vi "UHR-Fleezers Control (host) - 9.4.vi"() -> ()   [LabVIEW 2009]
uses:
  <vilib>/Utility/miscctls.llb/LVPoint32TypeDef.ctl
  <vilib>/Utility/miscctls.llb/LVMinMaxIncTypeDef.ctl
  <vilib>/userDefined/High Color/nirio_resource_hc.ctl
  <vilib>/Instr/_visa.llb/VISA Configure Serial Port (Instr).vi
  <vilib>/Platform/TimedLoop/XDataNode/XDataNode.xnode
  <vilib>/Platform/TimedLoop/XDataNode/loadlvalarms.vi
  <vilib>/Platform/TimedLoop/XDataNode/timing_clust.ctl
  <vilib>/Platform/TimedLoop/XDataNode/nitl_modes.ctl
  <vilib>/Platform/TimedLoop/XDataNode/wakeup.ctl
  <vilib>/rvi/interface/nirviOpenFPGA/nirviOpenFPGA.xnode
  FPGA Bitfiles/UHR-Fleezers Instr~3C_FPGA Target_UHR-Fleezers Contr~C3.lvbitx
  UHR-Fleezers Control (fpga) - 9.2.vi
  <vilib>/FPGAPlugInAG/PCIe-7852R/nirviIntfOpen_PCIe-7852R.vi
  <vilib>/rvi/interface/nirviMethod/nirviMethod.xnode
  <vilib>/Utility/error.llb/Merge Errors.vi
  <vilib>/LabVIEW Targets/FPGA/Rio/nirio_HostInterface/nirio_Reset.vi
  <vilib>/LabVIEW Targets/FPGA/Rio/nirio_HostInterface/nirio_DMAStopAll.vi
  <vilib>/rvi/interface/common/niFpgaNodeNameForErrorReporting.ctl
  <vilib>/rvi/errors/niLvFpgaWhatHappensToTopLevelVI.ctl
  <vilib>/LabVIEW Targets/FPGA/Rio/nirio_HostInterface/nirio_DisableInterrupts.vi
  <vilib>/Utility/error.llb/Error Cluster From Error Code.vi
  <vilib>/rvi/errors/niLvFpgaAdjustHostInterfaceError.vi
  <vilib>/rvi/interface/nirviReadWriteControl/nirviReadWriteControl.xnode
  <vilib>/LabVIEW Targets/FPGA/Rio/nirio_HostInterface/nirio_WriteBig.vi
  <vilib>/LabVIEW Targets/FPGA/Rio/nirio_HostInterface/nirio_DMAConfigure.vi
  <vilib>/LabVIEW Targets/FPGA/Rio/nirio_HostInterface/nirio_DMAStop.vi
  <vilib>/RVI Host/nirviSupport.llb/nirviErrorClusterFromErrorCode.vi
  <vilib>/LabVIEW Targets/FPGA/Rio/nirio_HostInterface/nirio_EnableInterrupts.vi
  <vilib>/rvi/errors/niLvFpgaReportInternalErrorWithAdditionalInfo.vi
  <vilib>/express/express analysis/Spectral/XNode/ExpressSpectralMeasurementsBlockNode.xnode
  <vilib>/express/express analysis/Spectral/Block/exnSpectralBlock spectral measurements PSD poly.vi
  <vilib>/express/express analysis/Spectral/Block/exnSpectralBlock spectral measurements PSD WFM.vi
  <vilib>/Waveform/WDTOps.llb/WDT Append Waveforms DBL.vi
  <vilib>/LabVIEW Targets/FPGA/Rio/nirio_HostInterface/nirio_ReadBig.vi
  <vilib>/rvi/interface/nirviCloseFPGA/nirviCloseFPGA.xnode
  <vilib>/FPGAPlugInAG/PCIe-7852R/nirviIntfClose_PCIe-7852R.vi
  <vilib>/vision/Avi1.llb/AviRefnum.ctl
  <vilib>/Analysis/NI_AALBase.lvlib
  <vilib>/Platform/TimedLoop/XDataNode/XDNodeRunTimeDep.lvlib
  openfpgaref.8.6.ctl
  NiRioSrv.dll
  <vilib>/vision/NI_Vision_Development_Module.lvlib
panel:
  out "Primary Video Display":T1(plugin-control)
  in  "Force Reset":bool
  in  "Force Yank":bool
  in  "Random Choice":bool=TRUE
  in  "N Array El":u8=3 min=1 step=1
  in  "Yank to Delta Array (MHz)":dbl[](array[numeric])=[16.3, 15.85, 14.85]
  in  "Yank Delay (s)":dbl=3.5
  in  "N pts to average":u16=6
  out "Fl. High":bool
  out "Waiting":bool
  in  "Fl. Delta Thresh. (kHz)":dbl=0.6
  in  "Fl. Triggered...":bool
  in  "Action":string(combo)="Yank"
  out "Duration (s)":dbl
  out "Waveform Graph":dbl[](graph) caption="APD Line Scan"
  in  "Total Volume\nFlushed (uL)":dbl
  in  "Inject Pump 2":bool caption="Inject Pump 2\n(Flush Center)"
  in  "Inject Pump 3":bool caption="Inject Pump 3\n(ADig Beads)"
  in  "Inject Pump 1 (DNA)":bool caption="Inject Pump 1 \n(DNA Beads)"
  out "Messages":string
  in  "APD Ave N":dbl=10.0
  out "Int. Time (s)":dbl
  in  "Stop All":bool
  out "sigma/mean":dbl
  out "Rate sigma (Hz)":dbl format="%0.2f"
  in  "Index":dbl=1.0 caption="Save File Index" min=1.0 step=1.0
  in  "Tab Control 6":T2(tab)=enum."Dual Display (Trap + APD)"
  out "All Signals":waveform(dbl)[](graph)
  in  "Signals to Plot":i32(listbox)
  out "Trap Disp. Freq. (Hz)":dbl caption="Freq. (Hz)" format="%#_6p"
  out "Display Period (s)":dbl caption="Period (s)" format="%#_6p"
  in  "Trap Disp. Downsample":dbl=20000.0 caption="Downsample"
  in  "APD Disp. Scale":dbl=0.1 caption="Scale (Divide,\nfor above plot only)"
  in  "APD Disp. Downsample":dbl=30.0 caption="Integrate" min=1.0 step=1.0
  out "APD Display Freq. (Hz)":dbl caption="Freq. (Hz)"
  out "APD Display Period (s)":dbl caption="Period (s)"
  out "RMS (Ang)":dbl format="%_2g"
  in  "Bead Sep. Int. Time (s)":dbl=5.0 caption="Int. Time (s)"
  in  "Below (kHz)":dbl=0.5
  in  "Above (kHz)":dbl=2.0
  in  "Adjust Scale\nto Mean":bool
  in  "Rescale on Mean":bool
  in  "Offset (nm)":dbl
  out "Mean":dbl caption="Mean (pN)" format="%#_3g"
  out "Force":waveform(dbl)[](graph)
  out "APD 1 Chart":waveform(dbl)(graph)
  in  "Calibration":u16(ring)=2 items=["None", "Position", "Force"]
  out "T1 X":dbl caption="T1 X (pN)" format="%0.2f"
  out "T2 X":dbl caption="T2 X (pN)" format="%0.2f"
  out "Bead Separation":waveform(dbl)(graph)
  in  "Amplitude (nm)":dbl=1.0
  out "Bead Mean (nm)":dbl caption="Mean (nm)" format="%0.2f"
  out "Difference":dbl caption="Difference (pN)" format="%.2g"
  out "APD 1 Graph":dbl[](graph) caption="Most Recent Time Trace"
  out "Trap Delta Graph":dbl[](graph) caption="Most Recent Time Trace"
  out "size(s) APD array":i32
  out "size(s) of 1 acq array":i32
  out "Delta Fl. (Hz)":dbl
  out "APD 1 Graph 2":dbl[](graph) caption="Most Recent Time Trace"
  in  "Flip Green Filter":bool
  in  "Set X Only":bool
  in  "Set Y Only":bool
  out "Detection Laser X":T1(plugin-control)
  out "APD 1":T1(plugin-control)
  out "Detection Laser Y":T1(plugin-control)
  out "Pointer Y (V)":dbl format="%_3g"
  out "Pointer X (V)":dbl format="%_3g"
  in  "Set Confocal Spot (X-Y)":bool
  out "FFT 1":cluster{"f0":dbl, "df":dbl, "magnitude":dbl[]}[](graph)
  out "FFT 2":cluster{"f0":dbl, "df":dbl, "magnitude":dbl[]}[](graph)
  in  "FFT 1 Choice 1":u16(ring) items=["T1 Y", "T1 X", "T1 Sum", "T2 Y", "T2 X", "T2 Sum", "T1 FB X", "T1 FB Sum", "T2 FB X", "T2 FB Sum", "PSD Y", "PSD X", "PSD Y Sum", "none"]
  in  "FFT 2 Choice 1":u16(ring)=13 items=["T1 Y", "T1 X", "T1 Sum", "T2 Y", "T2 X", "T2 Sum", "T1 FB X", "T1 FB Sum", "T2 FB X", "T2 FB Sum", "PSD Y", "PSD X", "PSD Y Sum", "none"]
  in  "FFT 1 Choice 2":u16(ring)=1 items=["T1 Y", "T1 X", "T1 Sum", "T2 Y", "T2 X", "T2 Sum", "T1 FB X", "T1 FB Sum", "T2 FB X", "T2 FB Sum", "PSD Y", "PSD X", "PSD Y Sum", "none"]
  in  "FFT 2 Choice 2":u16(ring)=13 items=["T1 Y", "T1 X", "T1 Sum", "T2 Y", "T2 X", "T2 Sum", "T1 FB X", "T1 FB Sum", "T2 FB X", "T2 FB Sum", "PSD Y", "PSD X", "PSD Y Sum", "none"]
  in  "Compute FFT":bool
  in  "Reset FFT":bool
  in  "# Spectra to Ave.":dbl=100.0
  out "Ave. Time (s)":dbl
  out "1 Channel":waveform(dbl)(graph)
  out "Slow mean":dbl format="%0.2f"
  in  "Slow mean N ave.":dbl=1.0 min=1.0 step=1.0
  out "Mean Intensity":dbl
  out "Sigma":dbl
  out "Sigma/Mean":dbl
  in  "Subtract mean":bool
  in  "High Res. Display":u16(ring) items=["T1 Y", "T1 X", "T1 Sum", "T2 Y", "T2 X", "T2 Sum", "T1 FB X", "T1 FB Sum", "T2 FB X", "T2 FB Sum", "PSD Y", "PSD X", "PSD Y Sum"]
  out "APD 1 Rate (Hz)":dbl format="%#_3p"
  in  "Tab Control":T3(tab)
  in  "TA Green Off?":bool
  in  "TA Cancel Save?":bool
  in  "Cal @ (MHz)":dbl=15.0
  out "Stage Moving":bool
  in  "Lower Ch. Cap.":bool
  in  "W/ Offset":bool=TRUE
  in  "Read Cal":bool
  out "Tether":bool
  in  "Tether Alarm?":bool=TRUE
  in  "Move to Delta 1 (MHz)":dbl=14.85
  in  "Then...":string(combo)="5"
  in  "Data Acq. Spot":bool
  in  "Confocal Linescan":bool
  in  "Speed (nm/s)":dbl=100.0
  in  "Stop F (pN)":dbl=3.0
  in  "Furthest Withdraw (MHz)":dbl=15.0
  in  "Closest Delta (MHz)":dbl=9.75 step=0.25
  in  "Fish for Tether":bool
  in  "Confocal Image":bool
  in  "Round T1 X":bool caption="Round"
  in  "T1 offset_x (mV)":dbl=-26.302542012392074 format="%#_2g"
  in  "T1 kappa_x (pN/nm)":dbl=0.22546432407642192 min=0.0 step=0.001 format="%#_2g"
  out "Time (s)":dbl
  out "Total Time (s)":dbl
  in  "Start Saving":bool
  in  "Limits Enable":bool=TRUE caption="Enable"
  in  "Limit Max (MHz)":dbl=16.0 caption="Max (MHz)"
  in  "Limit Min (MHz)":dbl=10.0 caption="Min (MHz)"
  in  "Cal sets to save":u32=50 min=1 step=1
  in  "Comment (data description)":string="testing confocal setup"
  out "Calibrating Trap...":bool
  in  "Trap 2 (ON/OFF)":bool
  in  "Trap 1 (ON/OFF)":bool
  in  "Save Calibration":bool
  in  "N sets to save":u32=200 caption="N Sets"
  in  "Save N Sets":bool
  out "Save file name":path
  in  "Save ave N":dbl=500.0 caption="Averaging Factor"
  out "Saving...":bool
  in  "Stop Saving":bool
  out "Progress":u16(slide) scale=0.0..100.0
  out "Manipulating Trap":bool
  out "Buffer Status":dbl(slide) scale=0.0..1.0
  out "Overflow (data lost)":bool
  in  "Reset":bool
  out "Data Rate (Hz)":dbl caption="Trap Data Rate (Hz)" format="%#_3p"
  out "Data Period (s)":dbl caption="Trap Data Period (s)" format="%#_6p"
  out "Save Data Rate (Hz)":dbl caption="Rate (Hz)" format="%#_6p"
  out "Save Data Period (s)":dbl caption="Period (s)" format="%#_6p"
  in  "T1 alpha_x (nm/V)":dbl=630.439304367558 step=10.0 format="%#_3g"
  in  "T2 alpha_x (nm/V)":dbl=704.7738222964198 step=10.0 format="%#_3g"
  in  "T2 kappa_x (pN/nm)":dbl=0.2030110880477556 min=0.0 step=0.001 format="%#_2g"
  in  "T2 offset_x (mV)":dbl=-26.67973517613748 format="%#_2g"
  in  "BD 1 Frequency 1 (MHz)":dbl=70.15 caption="T1 X (MHz)" min=60.0 max=90.0 step=1.0 format="%#_6p"
  in  "BD 1 Frequency 2 (MHz)":dbl=85.0 caption="T2 X (MHz)" min=60.0 max=90.0 step=1.0 format="%#_6p"
  in  "Green Laser ON/Interlacing":bool
  in  "Round T2 X":bool caption="Round"
  in  "AO1":dbl(slide)=5.61 caption="Confocal Y (V)" min=0.0 max=10.0 step=0.01 scale=0.0..10.0 scale format="%_1f"
  in  "AO2":dbl(slide)=3.9 caption="Confocal X (V)" min=0.0 max=10.0 step=0.01 scale=0.0..10.0 scale format="%_1f"
  in  "Upper Cap.":bool
  in  "Lower Cap.":bool
  in  "Trap Raster Scan":bool
  out "Raster Scanning...":bool
  in  "Trap Delta (MHz)":dbl=15.0
  in  "Dump Beads":bool
  in  "Wait Before Save (s)":u32=1
  out "Attempts":dbl
  in  "Attempt Limit":dbl=30.0 caption="Limit"
  in  "Setpoints (V)":cluster{"Set 1":dbl, "Set 2":dbl}={"Set 1"=9.0, "Set 2"=9.0}
  in  "Offset @ (MHz)":dbl=13.0
  in  "Move to Delta 2 (MHz)":dbl=15.0
  in  "Position Label 5":string="Lower Channel Cap" caption="5"
  in  "Move to Position":bool
  in  "Position":dbl=1.0 min=1.0 max=10.0 step=1.0
  in  "Set Position":bool
  in  "Saved Stage Positions":dbl[][](array[numeric])=[[1.0, 1.06186, -0.64809, -0.00713], [2.0, 0.0, 0.0, 0.0], [3.0, 2.01611, -0.29927, -0.00713], [4.0, 2.01611, 0.31655, -0.00713], [5.0, 0.0, 0.0, 0.0], [6.0, 0.0, 0.0, 0.0], [7.0, 0.0, 0.0, 0.0], [8.0, 0.0, 0.0, 0.0], [9.0, 0.0, 0.0, 0.0], [10.0, 0.0, 0.0, 0.0]]
  in  "Move to Position 5":bool
  in  "z nudge increment (um)":dbl=0.5
  in  "+z":bool
  in  "Position 1 Label":string="Upper capillary" caption="1"
  in  "Set Position 1":bool
  in  "Set Position 2":bool
  in  "Set Position 3":bool
  in  "Set Position 4":bool
  in  "Move to Position 3":bool
  in  "Move to Position 4":bool
  in  "Move to Position 2":bool
  in  "Move to Position 1":bool
  in  "Position 2 Label":string="Lower capillary" caption="2"
  in  "Position 3 Label":string="Measurement spot" caption="3"
  in  "Position 4 Label":string="Dump beads" caption="4"
  in  "-z":bool
  in  "Set Position 5":bool
  out "Stage Control Serial Error":errorcluster
  in  "Top Ch Inject Rate (ul/h)":dbl=10.0
  in  "Pump write delay (ms)":dbl=300.0
  in  "All Pump Parameters":T4={"Pump 1"={"Diameter (mm)"=4.61, "Units"=3.0, "Volume"=0.0, "Rate"=0.0}, "Pump 2"={"Diameter (mm)"=4.61, "Units"=3.0, "Volume"=0.0, "Rate"=0.0}, "Pump 3"={"Diameter (mm)"=4.61, "Units"=3.0, "Volume"=0.0, "Rate"=0.0}}
  in  "Top Ch Inject Volume (uL)":dbl=100.0
  in  "Pump pause delay (ms)":u32
  in  "Bottom Ch Inject Volume (uL)":dbl=100.0
  in  "Bottom Ch Inject Rate (ul/h)":dbl=10.0
  in  "Flush Center Ch Volume (uL)":dbl=15.0
  in  "Flush Center Ch Rate (ul/m)":dbl=100.0
  in  "Tab Control 2":T5(tab)=enum."AOD Raster Scan"
  out "Total Counts (ticks)":u32
  in  "Trap ON/OFF X or Y Amp?":bool=TRUE
  in  "Oscillate Set 1":bool
  in  "Trap 1 ON":bool
  in  "Number Interlace Sets":u8=3 min=1 max=3
  in  "DIO count 3 (ticks)":u32=200
  in  "DIO count 2 (ticks)":u32=200
  in  "DIO count 1 (ticks)":u32=200
  in  "BD 2 Amplitude 3 (%)":dbl min=0.0 max=50.0 step=1.0
  in  "BD 2 Amplitude 2 (%)":dbl min=0.0 max=50.0 step=1.0
  in  "BD 2 Amplitude 1 (%)":dbl min=0.0 max=50.0 step=1.0
  in  "BD 1 Amplitude 3 (%)":dbl min=0.0 max=50.0 step=1.0
  in  "BD 1 Amplitude 2 (%)":dbl=35.0 min=0.0 max=50.0 step=1.0
  in  "BD 1 Amplitude 1 (%)":dbl=10.0 min=0.0 max=50.0 step=1.0
  in  "BD 2 Frequency 3 (MHz)":dbl=26.0 min=0.0 max=40.0 step=1.0 format="%#_6p"
  in  "BD 1 Frequency 3 (MHz)":dbl=70.0 min=60.0 max=90.0 step=1.0 format="%#_6p"
  in  "BD 2 Frequency 2 (MHz)":dbl=26.0 min=0.0 max=40.0 step=1.0 format="%#_6p"
  in  "BD 2 Frequency 1 (MHz)":dbl=26.0 min=0.0 max=40.0 step=1.0 format="%#_6p"
  in  "Not-Interlacing Set":enum32{"Set 1", "Set 2", "Set 3"}(radio)
  in  "Interlace":bool=TRUE
  in  "Trap 2 ON":bool
  in  "Trap 3 ON":bool
  in  "Scan axis 2":bool=TRUE
  in  "Osc. freq. (Hz)":dbl=0.25
  in  "Osc. amp. (MHz)":dbl=2.0
  out "Coords":T6
  in  "Manipulation Scaling":cluster{"Horizontal":dbl, "Vertical":dbl}={"Horizontal"=0.075, "Vertical"=0.01}
  in  "Freq or Amp switch first":bool=TRUE
  in  "Swap F1 and F2":bool
  in  "Freq switch delay":u16
  in  "Amp switch delay":u16=5
  in  "MCL Step Increment (V_int)":dbl=3.0
  out "Time to Finish All (min)":dbl format="%#_2p"
  in  "Scan Speed (nm/s)":dbl=100.0
  in  "Scan Range (nm)":dbl=200.0
  in  "Step Size (nm)":dbl=1.0
  in  "MCL/AOM Scale Tweak":dbl=1.0
  in  "MCL Step Position Ratio":dbl=0.5
  in  "Move MCL Also?":bool=TRUE
  out "Final sep (nm)":dbl
  out "Initial sep (nm)":dbl
  out "Save index":dbl
  out "Final delta (MHz)":dbl
  out "Initial delta (MHz)":dbl
  out "Final freq. (MHz)":dbl
  out "Initial freq. (MHz)":dbl
  in  "Saved AOD Raster Scan Parameter Sets":T7(array[cluster])=[{"Scan Range AOD (nm) 2"=500.0, "Step Size AOD (nm) 2"=1.0, "Scan Speed AOD (nm/s) 2"=200.0, "Number of scans (AOD) 2"=1, "Label"=""}, {"Scan Range AOD (nm) 2"=1000.0, "Step Size AOD (nm) 2"=1.0, "Scan Speed AOD (nm/s) 2"=200.0, "Number of scans (AOD) 2"=5, "Label"="wide offset scan"}, {"Scan Range AOD (nm) 2"=20.0, "Step Size AOD (nm) 2"=0.68, "Scan Speed AOD (nm/s) 2"=0.68, "Number of scans (AOD) 2"=1, "Label"="2 bp steps"}]
  in  "Load parameters":bool
  out "Scan Range (MHz)":dbl=10.0
  in  "Restart DMA? (AOD)":bool=TRUE caption="Restart DMA?"
  out "Incr. int (AOD)":i64
  out "Time/Scan (s) (AOD)":dbl format="%#_2p"
  out "Data points/scans":dbl
  out "Data points/scan (f/b)":dbl
  in  "Save scans":bool=TRUE
  out "AOD Scan I":u64 caption="Scan I"
  in  "Continuous AOD Scanning":bool caption="Continuous Scanning"
  in  "Abort AOD Scan":bool caption="Abort Scan"
  in  "Scan BD":bool=TRUE
  out "Cycles/step (AOD)":u64=400 format="%.0p"
  in  "Number of F/B Scans (AOD)":u16=3 min=1
  out "Scan steps (AOD)":u64=1000
  out "Scan Increment (MHz)":dbl=0.2
  out "AOD Scanning":bool caption="Scanning"
  in  "Start AOD Scan":bool caption="Start Scan"
  out "N sets should be saved":dbl
  out "Progress 2":u16(slide) caption="Progress" scale=0.0..100.0
  in  "Abort save 2":bool caption="Abort save"
  in  "Trap 1 Bead Size (nm)":dbl=860.0
  in  "Trap 2 Bead Size (nm)":dbl=790.0
  out "MCL Count":dbl
  in  "All FB On/Off":bool=TRUE
  in  "AI2 to Setpoint":cluster{"Set 1":bool, "Set 2":bool}
  out "AI2 (V)":cluster{"Set 1":dbl, "Set 2":dbl}
  in  "Reset Feedback":cluster{"Set 1":bool, "Set 2":bool}
  in  "PID Gains":T8={"Set 1"={"proportional gain (Kc)"=0, "integral gain (Kc*Ts/Ti)"=5, "derivative gain (Kc*Td/Ts)"=0}, "Set 2"={"proportional gain (Kc)"=0, "integral gain (Kc*Ts/Ti)"=5, "derivative gain (Kc*Td/Ts)"=0}}
  in  "Feedback On/Off":cluster{"Set 1":bool, "Set 2":bool}={"Set 1"=TRUE, "Set 2"=TRUE}
  in  "Tab Control 3":enum32{"Timing", "MCL Scan", "Analog Out"}(tab)=enum."MCL Scan"
  out "APD Gate Late Counter":u32
  in  "- phase (APD Gate)":bool
  in  "+ phase (APD Gate)":bool
  out "APD Gate Relative Phase":i16
  in  "Phase Adj. (APD Gate)":i16=20
  in  "Initial Phase Adjustment (APD Gate)":i16=50
  in  "Save APD Data\nwith Trap Data":bool=TRUE
  out "APD FIFO Elements Remaining":u32
  in  "- phase (APD Acq)":bool
  in  "+ phase (APD Acq)":bool
  out "APD Acq Late Counter":u32
  out "APD Acq Relative Phase":i16
  in  "Phase Adj. (APD Acq)":i16=20
  in  "Initial Phase Adjustment (APD Acq)":i16
  in  "Invert APD Gate":bool caption="Invert Gate"
  in  "APD Gate OFF Count":u32=450 caption="Gate OFF Count"
  in  "APD Gate ON Count":u32=150 caption="Gate ON Count"
  in  "APD Gate":enum32{"ON", "OFF", "Interlace"}(radio)=enum."Interlace"
  in  "APD Integration Time (s)":dbl=0.01 caption="Integration Time (s)"
  out "APD Acq Rate (Hz)":dbl=20000000.0 caption="Rate (Hz)"
  out "APD Samples/FIFO Acq.":dbl
  out "APD Elements/DMA read":u32
  out "APD Int. Count":u32 format="%.0p"
  in  "Tab Control 5":enum32{"PSD X", "PSD Y", "Other Data Channel"}(tab)
  out "Data map":dbl[][](graph)
  in  "Channel":i32=4
  in  "Abort MCL Scan":bool
  out "MCL Scan I":u64
  out "MCL Scanning":bool
  in  "Start MCL Scan":bool
  out "wait to reset values":bool
  in  "Tab Control 4":enum32{"Scan Settings", "MCL FPGA Loop Timing"}(tab)
  out "Total Time (s)":dbl
  in  "Scan lines (y)":u64=20
  in  "Fast Scan Dir":bool=TRUE
  in  "2D or 1D Scan":bool=TRUE
  out "Initial X":dbl
  out "Initial Y":dbl
  out "Time/f+b scan (s) (MCL)":dbl caption="Time/scan (s)"
  in  "Number of scans (MCL)":u64=1 caption="Scans"
  in  "Scan steps (MCL)":u64=40 caption="Scan steps (x)"
  in  "N APD Samp/step":dbl=3.0
  in  "Scan Range (V)\n(of steps)":dbl=3.5
  in  "Restart DMA? (MCL)":bool=TRUE caption="Restart DMA?"
  in  "Continuous MCL Scanning":bool caption="Cont. Scanning"
  in  "Center Scan":bool=TRUE
  in  "Save Data (MCL)":bool=TRUE caption="Save Data"
  out "Actual Incr. int (MCL)":i16 caption="Incr. int"
  out "Desired incr (int)":dbl
  out "Desired Scan Incr (V)":dbl
  out "N sets should be saved (MCL)":dbl caption="N sets should be saved"
  out "Data points/scans (MCL)":dbl caption="Data points/scans"
  out "Data points/scan (f+b)":dbl caption="points/scan (f+b)"
  out "Cycles/step (MCL)":u64 caption="Cycles/step" format="%.0p"
  out "Actual MCL Inc (V)":dbl
  in  "Phase adjust (MCL)":i16 caption="Phase adjust"
  out "Relative Phase (MCL)":i16 caption="Relative Phase"
  in  "Initial Phase Adj. (MCL)":i16 caption="Initial Phase Adj."
  in  "Update Count (MCL)":u32=600
  in  "+ phase (MCL)":bool
  in  "- phase (MCL)":bool
  out "MCL Late Counter":u32
  in  "APD 1 AO Mult.":i16=1 min=1
  in  "APD 2 AO Mult.":i16=1 min=1
  in  "APD 1 AO offset":i16
  in  "APD 2 AO offset":i16
  in  "Tab Control 7":enum32{"Green FB Signals", "Slow MCL Scan"}(tab)
  out "Green FB Plot":dbl(graph)
  out "MCL Scan 2":cluster{"Begin (V)":dbl, dbl, dbl[]}(graph)
  out "MCL Scan":cluster{"Begin (V)":dbl, dbl, dbl[]}(graph)
  in  "Green laser mode":enum32{"Laser ON", "Laser OFF", "Interlace"}(radio)=enum."Interlace"
  in  "GI Frequency, ON count":u32=150 min=1 step=1
  in  "Invert GI":bool
  out "GI Late Counter":u32
  in  "Phase adj. (GI)":i16=5
  out "GI relative phase":i16
  in  "+ phase (GI)":bool
  in  "Initial Phase Adjustment (GI)":i16=15
  in  "GI Frequency, OFF count":u32=450 min=1 step=1
  in  "- phase (GI)":bool
  out "Green FB Signals (V)":cluster{"Y":dbl, "X":dbl, "Sum":dbl}
  out "Relative phase (Green FB)":i16
  in  "+ phase (Green FB)":bool
  in  "- phase (Green FB)":bool
  in  "Green FB Count":u32=600
  in  "Phase adj. (Green FB)":i16=10
  in  "Initial Phase Adjustment (Green FB)":i16=50
  in  "Green FB On/Off":bool=TRUE
  in  "Current When FB OFF (%)":dbl=87.0 min=0.0 max=100.0 step=1.0
  in  "Green int current ON count adj":u32=150
  in  "Green FB Gains":T9={"proportional gain (Kc)"=10, "integral gain (Kc*Ts/Ti)"=5, "derivative gain (Kc*Td/Ts)"=0}
  in  "Green FB Setpoint (mV)":dbl=100.0
  in  "- phase (GI) 2":bool
  in  "Initial Phase Adjustment (GI) 2":i16=-100
  in  "+ phase (GI) 2":bool
  out "GI relative phase 2":i16
  in  "Phase adj. (GI) 2":i16=20
  out "GI Late Counter 2":u32
  in  "# Samples/trap":dbl=20000.0 format="%#_6p"
  out "Elements/DMA read":u32 format="%.0p"
  out "Ave. Rate (Hz)":dbl format="%#_6p"
  out "FIFO El. Rem.":u32 format="%.0p"
  in  "Phase adj. (AI1)":i16=15
  out "Relative phase (AI1)":i16
  in  "+ phase (AI1)":bool
  in  "- phase (AI1)":bool
  out "Late Counter (AI1)":u32
  in  "Initial Phase Adjustment (AI1)":i16=220
  out "AI rate (Hz)":dbl=50000.0 format="%#_6p"
  in  "AI Count (ticks)":u32=200
  out "# Samples/channel":u32=20000 format="%.0p"
  in  "FIFO Depth":u32=600000 format="%.0p"
  in  "Detector Type":string(combo)="IR-QPD + PSD + FB-QPD X position"
  in  "N Acq Sets (Traps + Fl.)":i16=3
  in  "Sets to FIFO (Traps)":T10={"Set 1"=TRUE, "Set 2"=TRUE, "Set 3"=FALSE}
  in  "FPGA Ave.":dbl=1.0 min=1.0 step=1.0
  out "Ave. Period (s)":dbl format="%#_6p"
  out "DMA Update Period (s)":dbl
  out "FPGA Averaging":bool
  out "Trap Sets":i16
  out "Counts/DMA":dbl format="%#_6p"
  in  "Video Capture Rate (Hz)":dbl=30.0
  in  "Video Index":dbl=1.0 min=1.0 step=1.0
  in  "New Video File":bool
  in  "Save Video":bool
  in  "Reset Averaging":bool
  in  "Averaging":bool
  in  "Save Image":bool
  in  "Image Index":dbl=1.0 min=1.0
  out "Path Out":path
  in  "Center Point":cluster{"X":i32, "Y":i32}={"X"=335, "Y"=271}
  in  "Zoom Factor":sgl=7.0
  out "Window Size":cluster{"Width":i32, "Height":i32}
  out "Window Position":cluster{"X Position":i32, "Y Position":i32}={"X Position"=40, "Y Position"=40}
  in  "Initial Window Size":cluster{"Width":i32, "Height":i32}={"Width"=884, "Height"=619}
  in  "Initial Window Position":cluster{"X Position":i32, "Y Position":i32}={"X Position"=796, "Y Position"=4}
  in  "Intensity Upper":dbl=88.0
  in  "Intensity Lower":dbl=66.0
  out "error out":errorcluster
  out "error out 2":errorcluster
  in  "Lost Tether Alarm Threshold (pN)":dbl=0.5
  in  "AOM X Cal (nm/MHz)":dbl=123.0
  in  "MCL X Cal (nm/V)":dbl=1070.0
  out "X RF Amplitude Limits (%)":T11={"Minimum"=0.0, "Maximum"=50.0, "Increment"=1.0}
  out "X RF Frequency Limits (MHz)":T11={"Minimum"=60.0, "Maximum"=90.0, "Increment"=1.0}
  out "Y RF Frequency Limits (MHz)":T11={"Minimum"=60.0, "Maximum"=90.0, "Increment"=1.0}
  out "Y RF Amplitude Limits (%)":T11={"Minimum"=0.0, "Maximum"=50.0, "Increment"=1.0}
  in  "Manip. X?":bool=TRUE
  in  "Manip. Y?":bool
  in  "Force Manip Abort":bool
  out "Read cal error":errorcluster
  in  "DAQ Delay (ms)":u32=1000
  in  "Start Scan":bool
  in  "Scan axis":bool=TRUE
  in  "Osc. amp. (V)":dbl=5.0
  in  "Osc. center (V)":dbl=5.0
  in  "Osc. freq. (Hz) 2":dbl=1.0
  in  "MCL Mode":u16(ring) items=["Manual Positioning", "Sinusoidal Wave", "Linear Scan"]
  in  "Begin (V)":dbl
  in  "End (V)":dbl=10.0
  in  "N Points":dbl=20.0
  in  "Delay to Interlace (s)":dbl
  in  "Delayed Interlace Start":bool
  in  "Read Lateness and Rel Phase":bool
  out "Vec Mean of T1 T2":dbl[](array[numeric])
  in  "Cal read wait (s)":u32=5
  out "Time tether formed":timestamp
  in  "Sample Chamber Stage Serial Port":refnum<visa-resource-name>="ChamberStageCOM4"
  in  "Syringe Pump Serial Port":refnum<visa-resource-name>="ChemyxPumpCOM3"
  # "Trap Display:"
  # "APD Display:"
  # "DAQ"
  # "Move Stage and Take Action"
  # "Trap Manipulation"
  # "Data Saving"
  # "Bead Calibration"
  # "Trap Position Difference Limits"
  # "DNA Beads"
  # "ADig Beads"
  # "Center channel"
  # "Units: \n1 = ml/m\n2 = ml/h\n3 = ul/m\n4 = ul/h"
  # "Rate param is ul/h\nVolume param is ul"
  # "X"
  # "Y"
  # "Oscillate Set 1 freq. (debugging)"
  # "BD 1"
  # "BD 2"
  # "AOD Raster Scan"
  # "Approx. trap separations"
  # "X"
  # "Y"
  # "Gate"
  # "X"
  # "2D"
  # "Y"
  # "1D"
  # "Green Laser Interlacing"
  # "Green FB Measurement"
  # "Digital Gate"
  # "Current Analog Control"
  # "Total AI Rates (NOT rates/trap)"
  # "(Samples/trap x Trap Sets)"
  # "(Samples/channel x\n8 if averaging (8 channels)\n4 if no averaging)"
  # "Trap 1"
  # "Trap 2"
  # "Flour./Trap 3"
  # "External Video Window"
  # "MCL Position Debugging"
  # "Temporary Control Storage\n(these used to be somewhere else, still want to keep them)"
  # "Y"
  # "X"
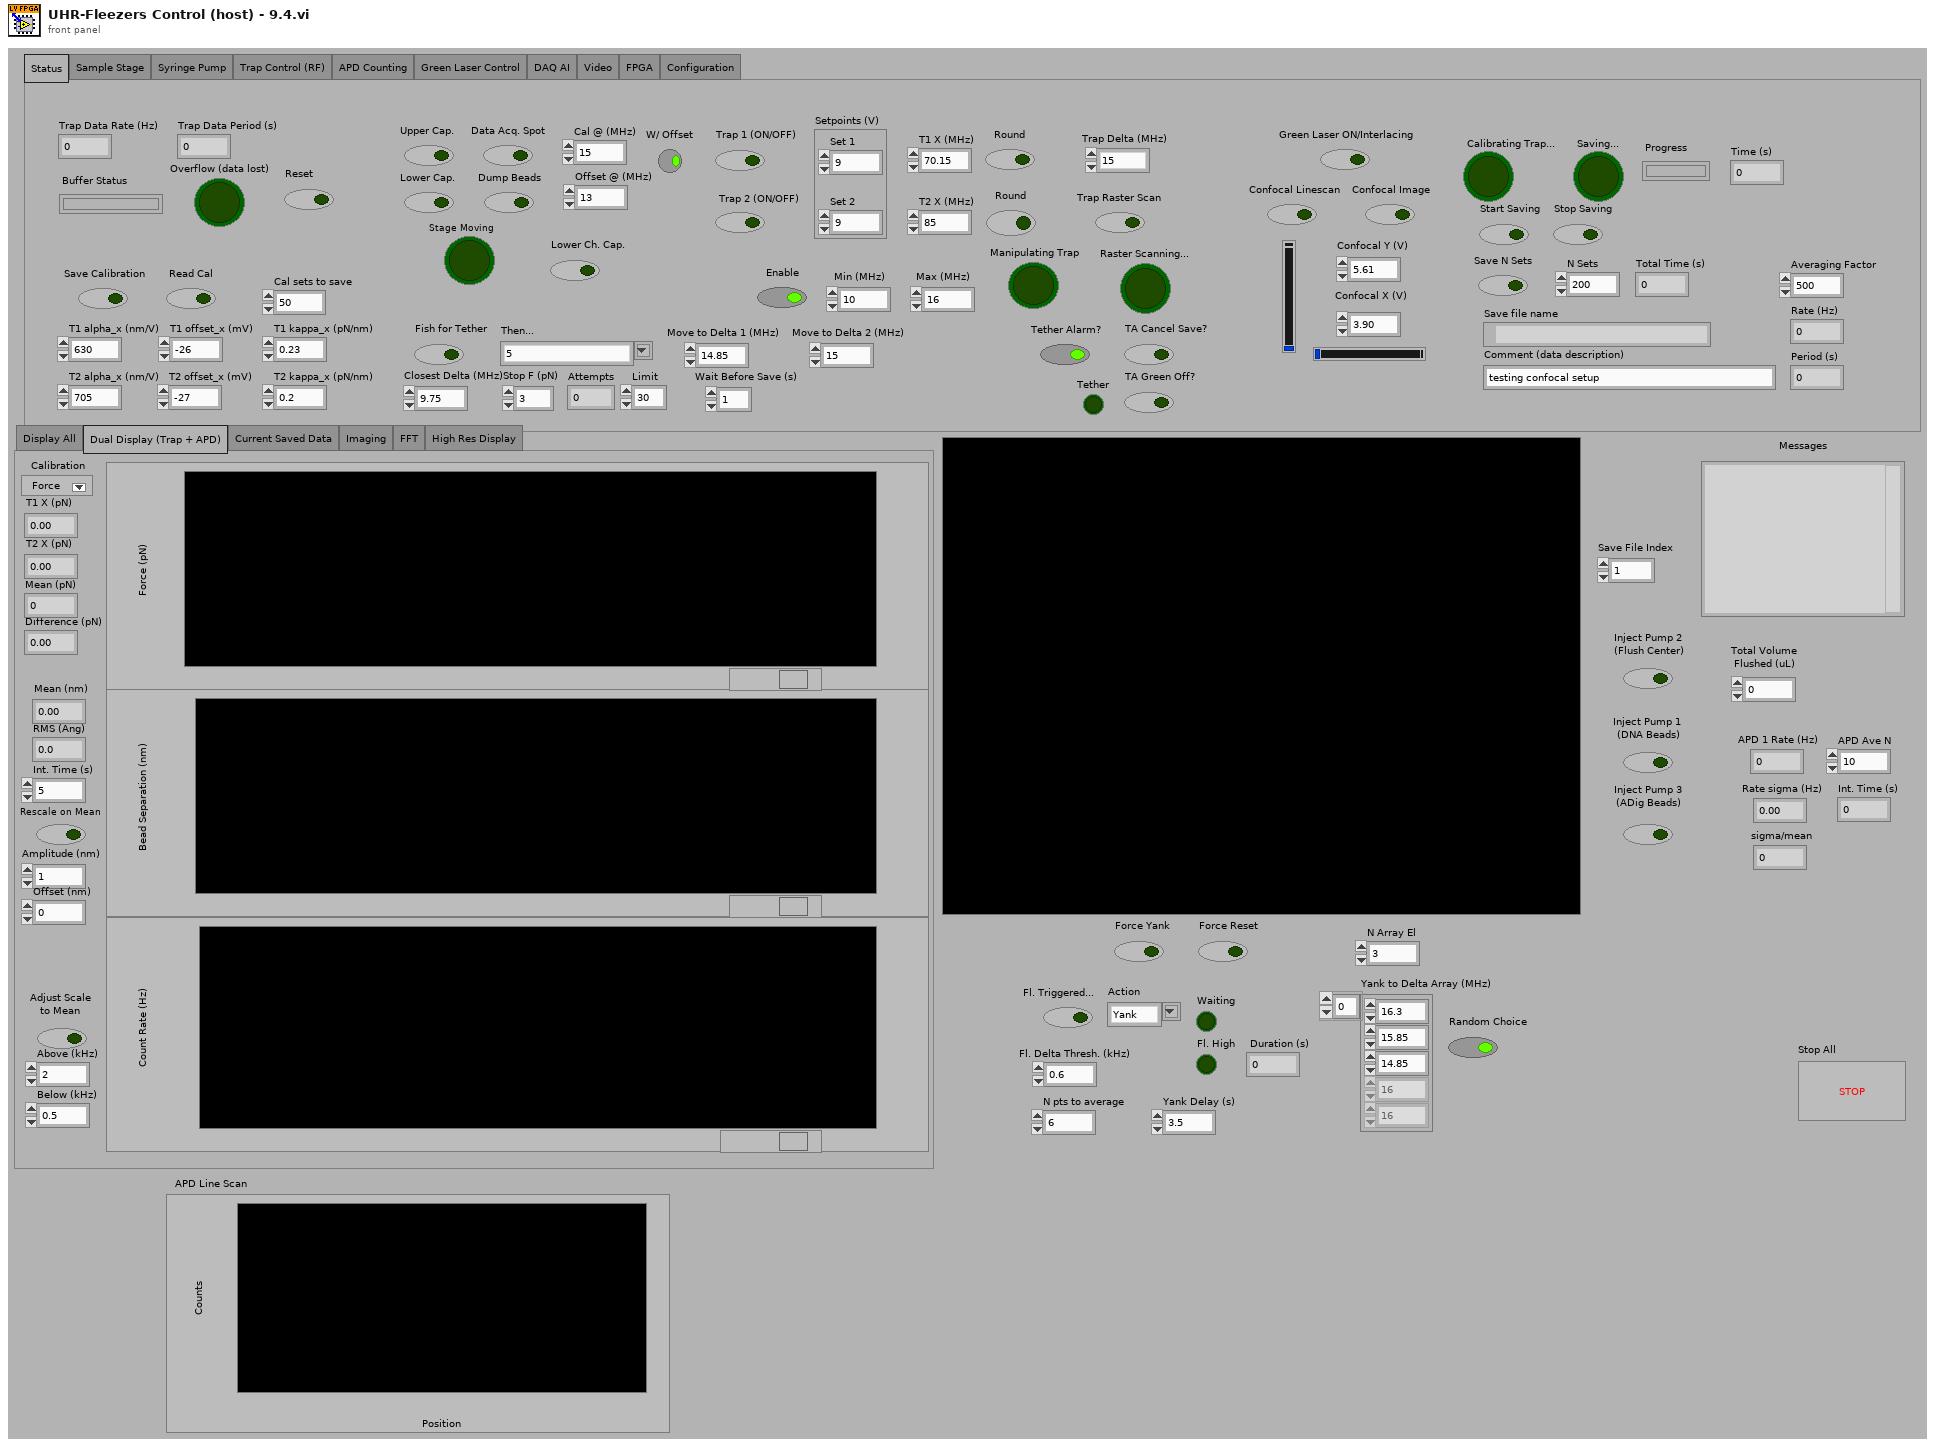
[diagram p1: front panel]
types:
  T1 = typedef "IMAQ Image.ctl" = refnum<image>
  T2 = enum32{"Display All", "Dual Display (Trap + APD)", "Current Saved Data", "Imaging", "FFT", "High Res Display"}
  T3 = enum32{"Status", "Sample Stage", "Syringe Pump", "Trap Control (RF)", "APD Counting", "Green Laser Control", "DAQ AI", "Video", "FPGA", "Configuration"}
  T4 = cluster{"Pump 1":cluster{"Diameter (mm)":dbl, "Units":dbl, "Volume":dbl, "Rate":dbl}, "Pump 2":cluster{"Diameter (mm)":dbl, "Units":dbl, "Volume":dbl, "Rate":dbl}, "Pump 3":cluster{"Diameter (mm)":dbl, "Units":dbl, "Volume":dbl, "Rate":dbl}}
  T5 = enum32{"IR Laser Interlacing (Direct RF Board Control Method)", "AOD Raster Scan", "Feedback on BD 1 Amp to Control AI2"}
  T6 = typedef "LVPoint32TypeDef.ctl" = cluster{"Horizontal":i32, "Vertical":i32}
  T7 = cluster{"Scan Range AOD (nm) 2":dbl, "Step Size AOD (nm) 2":dbl, "Scan Speed AOD (nm/s) 2":dbl, "Number of scans (AOD) 2":u16, "Label":string}[]
  T8 = cluster{"Set 1":cluster{"proportional gain (Kc)":i16, "integral gain (Kc*Ts/Ti)":i16, "derivative gain (Kc*Td/Ts)":i16}, "Set 2":cluster{"proportional gain (Kc)":i16, "integral gain (Kc*Ts/Ti)":i16, "derivative gain (Kc*Td/Ts)":i16}}
  T9 = cluster{"proportional gain (Kc)":i16, "integral gain (Kc*Ts/Ti)":i16, "derivative gain (Kc*Td/Ts)":i16}
  T10 = cluster{"Set 1":bool, "Set 2":bool, "Set 3":bool}
  T11 = typedef "LVMinMaxIncTypeDef.ctl" = cluster{"Minimum":dbl, "Maximum":dbl, "Increment":dbl}
  T12 = typedef "Image Type" = u32
  T13 = typedef "nirio_resource_hc.ctl" = tag
  T14 = typedef "openfpgaref.8.6.ctl" = refnum<k20>
  T15 = typedef "niFpgaNodeNameForErrorReporting.ctl" = enum16{"Open FPGA VI Reference", "Read/Write Control", "Invoke Method: Abort", "Invoke Method: Acknowledge IRQ", "Invoke Method: Download", "Invoke Method: FIFO.Configure", "Invoke Method: FIFO.Read", "Invoke Method: FIFO.Start", "Invoke Method: FIFO.Stop", "Invoke Method: FIFO.Write", "Invoke Method: Reset", "Invoke Method: Run", "Invoke Method: Wait on IRQ", "Close FPGA VI Reference"}
  T16 = typedef "niLvFpgaWhatHappensToTopLevelVI.ctl" = enum16{"top level VI scripted behind XNode", "top level VI inlined behind XNode"}
  T17 = typedef "XDNodeRunTimeDep.lvlib/timing_clust.ctl" = cluster{"Expected End [f-1]":u64, "Actual End [f-1]":u64, "Finished Late? [f-1]":bool, "Expected End [i-1]":u64, "Actual End [i-1]":u64, "Finished Late? [i-1]":bool, "Expected Start [i]":u64, "Actual Start [i]":u64, "Expected Start [f]":u64, "Actual Start [f]":u64, "Source Name":string, "Structure Name":string, "Period":i64, "Deadline":i64, "Offset":i64, "Start":i64, "Priority":i32, "Timeout":i32, "Mode":T18, "Wakeup Reason":T19, "Error":errorcluster, "Source Type":string, "Secondary Source Type":string, "Global End Time":u64, "Global Start Time":u64, "Frame Duration":u64, "Iteration Duration":u64, "Assigned CPU":i32, "I/O Scan Engine Mode":u32}
  T18 = typedef "XDNodeRunTimeDep.lvlib/nitl_modes.ctl" = enum32{"No Change", "Process missed periods, maintain original phase", "Discard missed periods, maintain original phase", "Process missed periods, ignore original phase", "Discard missed periods, ignore original phase"}
  T19 = typedef "XDNodeRunTimeDep.lvlib/wakeup.ctl" = enum32{"Normal", "Aborted", "Asynchronous wakeup", "Timing source error", "Timed loop error", "Timeout"}
  T20 = enum16{"big-endian, network order", "native, host order", "little-endian"}
  T21 = enum16{"open", "replace", "create", "open or create", "replace or create", "replace or create with confirmation"}
  T22 = cluster{"Scan Range AOD (nm) 2":dbl, "Step Size AOD (nm) 2":dbl, "Scan Speed AOD (nm/s) 2":dbl, "Number of scans (AOD) 2":u16, "Label":string}
  T23 = cluster{"[0]":dbl, "[1]":dbl, "[2]":dbl, "[3]":dbl, "[4]":dbl, "[5]":dbl}
  T24 = cluster{"Diameter (mm)":dbl, "Units":dbl, "Volume":dbl, "Rate":dbl}
  T25 = cluster{"Left":i32, "Top":i32, "Width":u32, "Height":u32}
  T26 = cluster{cluster{"Left":i32, "Top":i32, "Width":u32, "Height":u32}}[]
  T27 = enum32{"setting", "request", "request control", "info", "statistics", "system settings", "I/O sub system", "HRT control", "camera descriptions", "device specific data", "event sub system settings", "event sub system results", "image memory manager"}
  T28 = typedef "AviRefnum.ctl" = refnum<k1>
  T29 = typedef "imagedata.ctl" = cluster{"image type":i32, "image depth":i32, "image":u8[], "mask":u8[], "colors":u32[], "Rectangle":cluster{"left":i16, "top":i16, "right":i16, "bottom":i16}}
  T30 = enum32{"Normal Display", "Dual Display (APD)", "FFT", "High Res Display"}
  T31 = cluster{"Origin Pixel":cluster{"X":sgl, "Y":sgl}, "Angle Relative to Horizontal (deg)":sgl, "Axis Reference":u32}
  T32 = typedef "Simple Grid Descriptor" = cluster{"X Step":sgl, "Y Step":sgl, "Unit":T33}
  T33 = typedef "Image Unit" = enum32{"Undefined", "Angström", "Micrometer", "Millimeter", "Centimeter", "Meter", "Kilometer", "Microinch", "Inch", "Feet", "Nautical miles", "Standard miles", "Steps"}
  T34 = cluster{"averaging mode":u16, "weighting mode":u16, "number of averages":u32}
  T35 = cluster{"dB On (F)":bool, "unwrap phase (F)":bool, "convert to degree (F)":bool}
  T36 = cluster{"Green FB Ch 0":i16, "Green FB Ch 1":i16, "Green FB Ch 2":i16}
  T37 = cluster{string, string, string, string, string, string, string, string}
  T38 = cluster{string, string, string, string, string, string, string, string, string, string, string, string}
  T39 = cluster{string, string, string, string, string, string, string, string, string, string, string, string, string}
  T40 = cluster{string, string, string, string, string, string, string, string, string, string, string, string, string, string}
  T41 = cluster{"f0":dbl, "df":dbl, "magnitude":dbl[]}[][]
  T42 = cluster{"Green FB Ch 0":dbl, "Green FB Ch 1":dbl, "Green FB Ch 2":dbl}
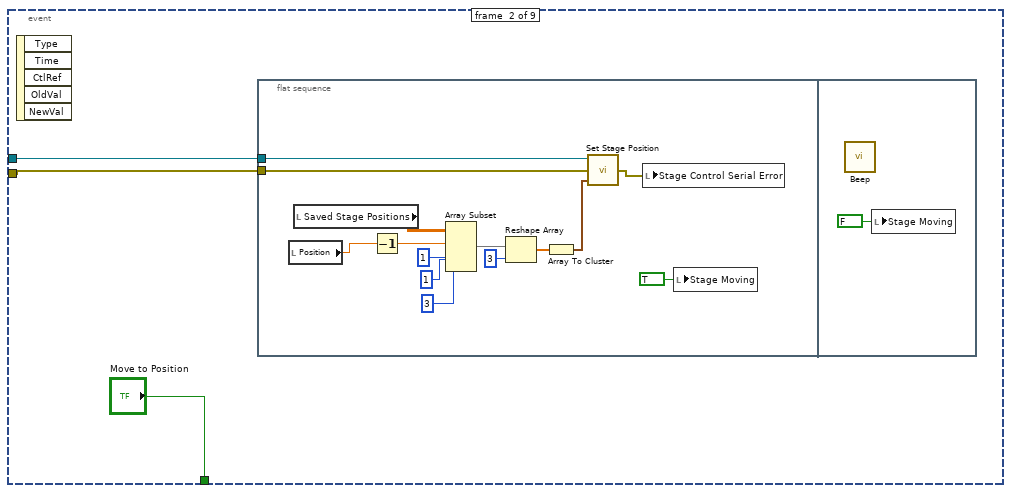
[diagram p2: hidden frame]
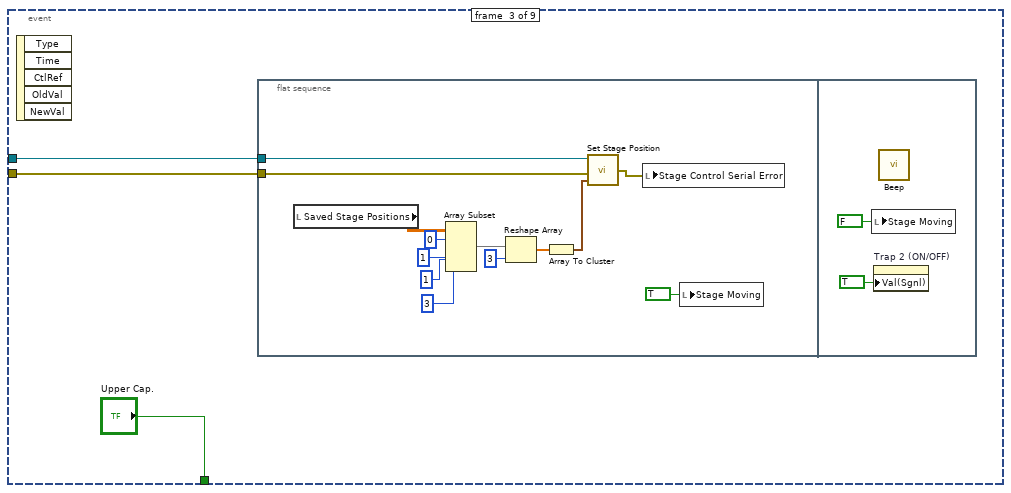
[diagram p3: hidden frame]
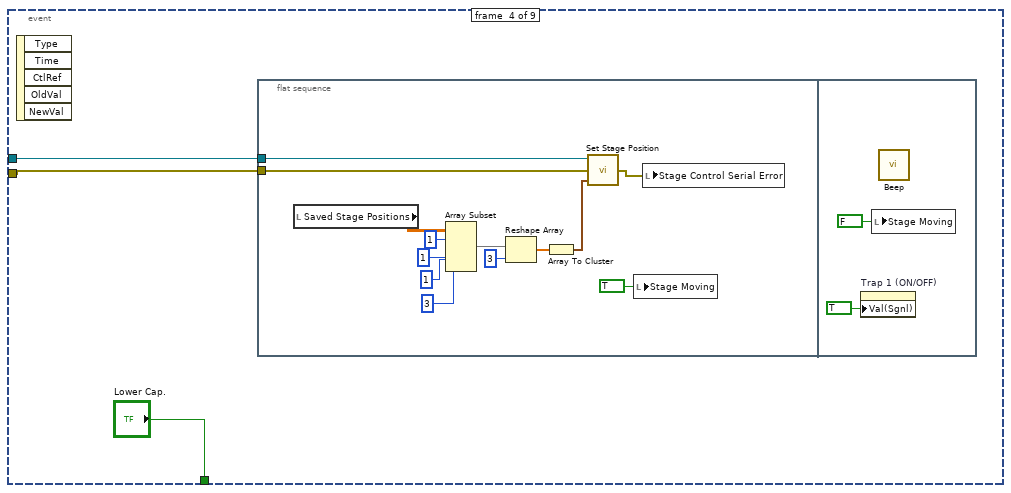
[diagram p4: hidden frame]
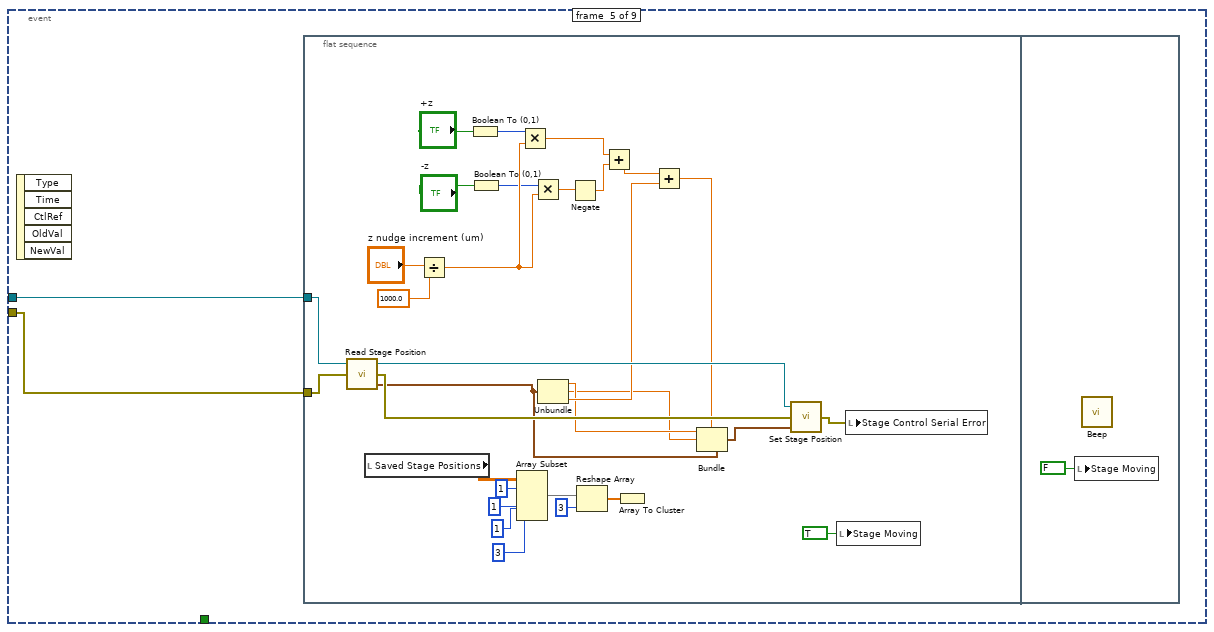
[diagram p5: hidden frame]
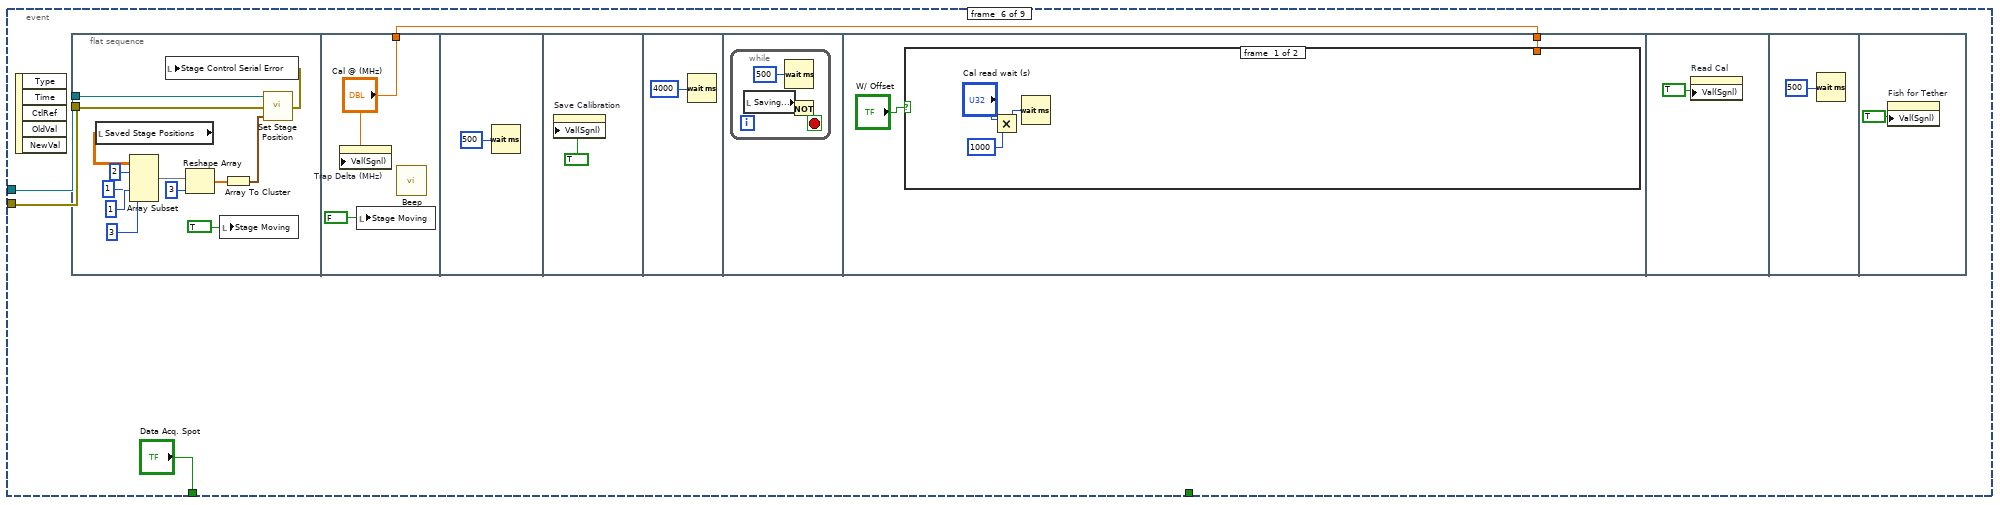
[diagram p6: hidden frame]
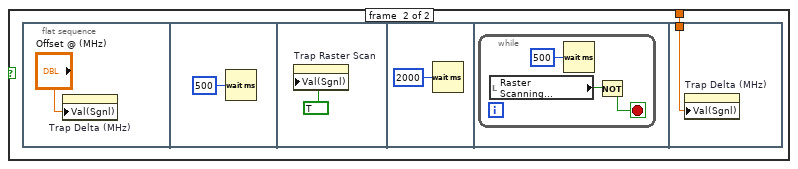
[diagram p7: hidden frame]
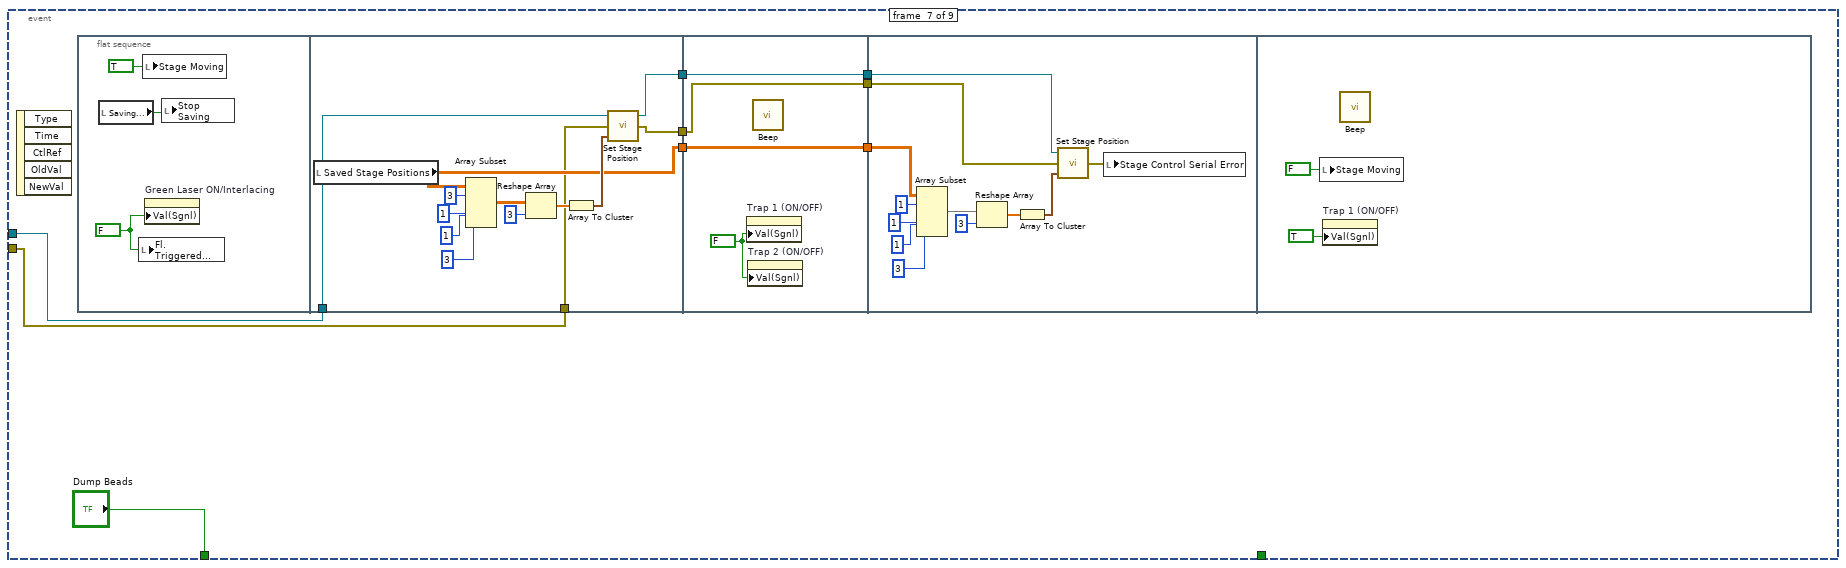
[diagram p8: hidden frame]
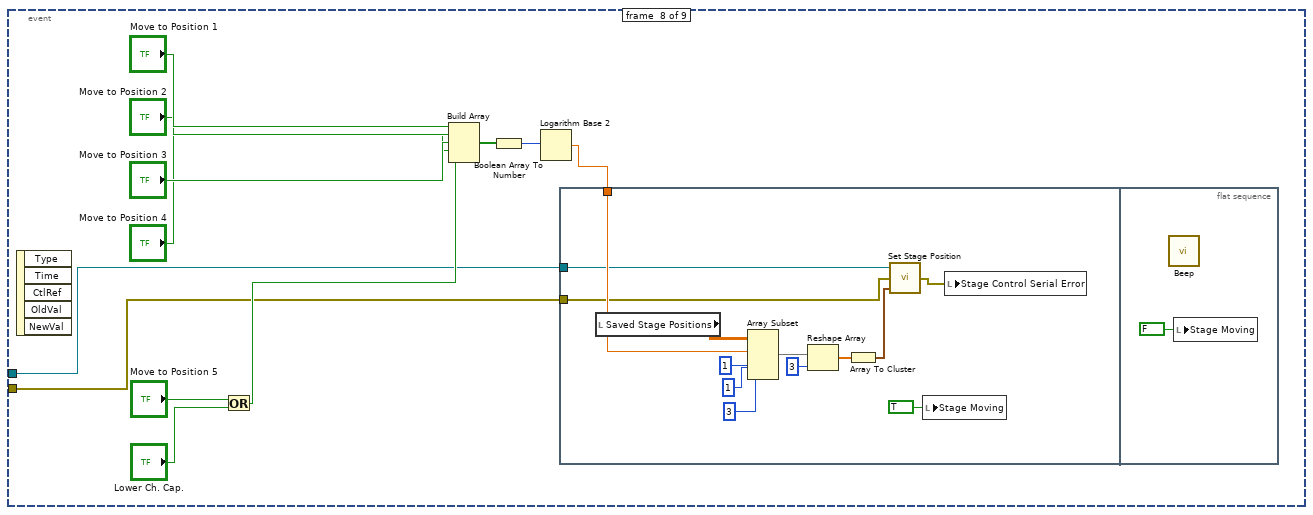
[diagram p9: hidden frame]
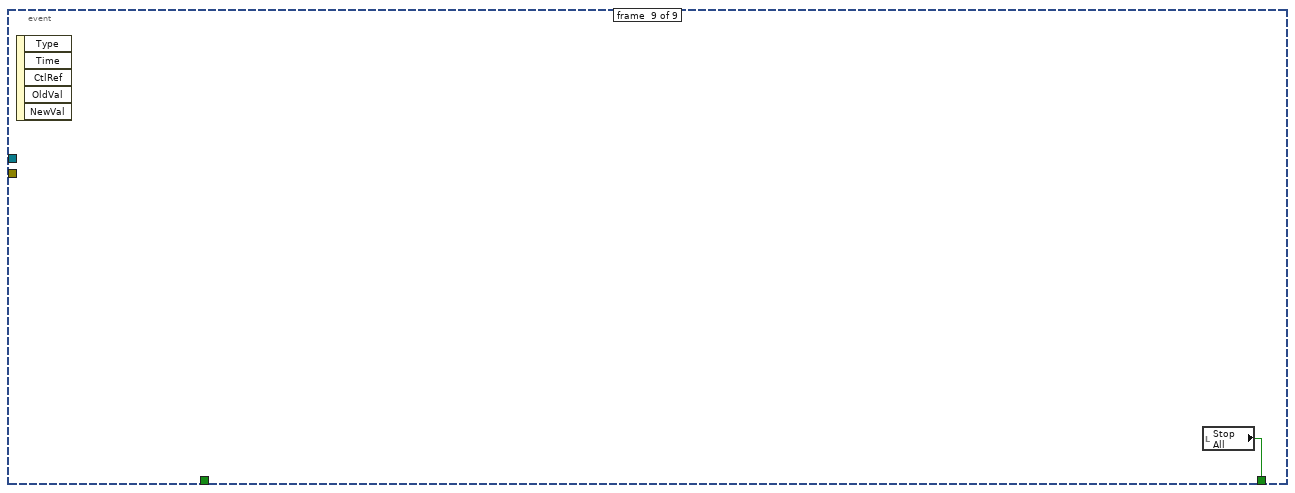
[diagram p10: hidden frame]
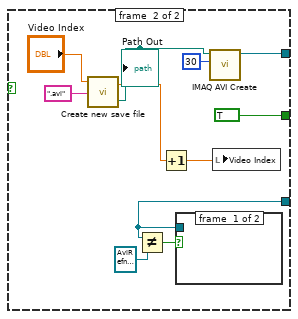
[diagram p11: hidden frame]
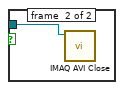
[diagram p12: hidden frame]
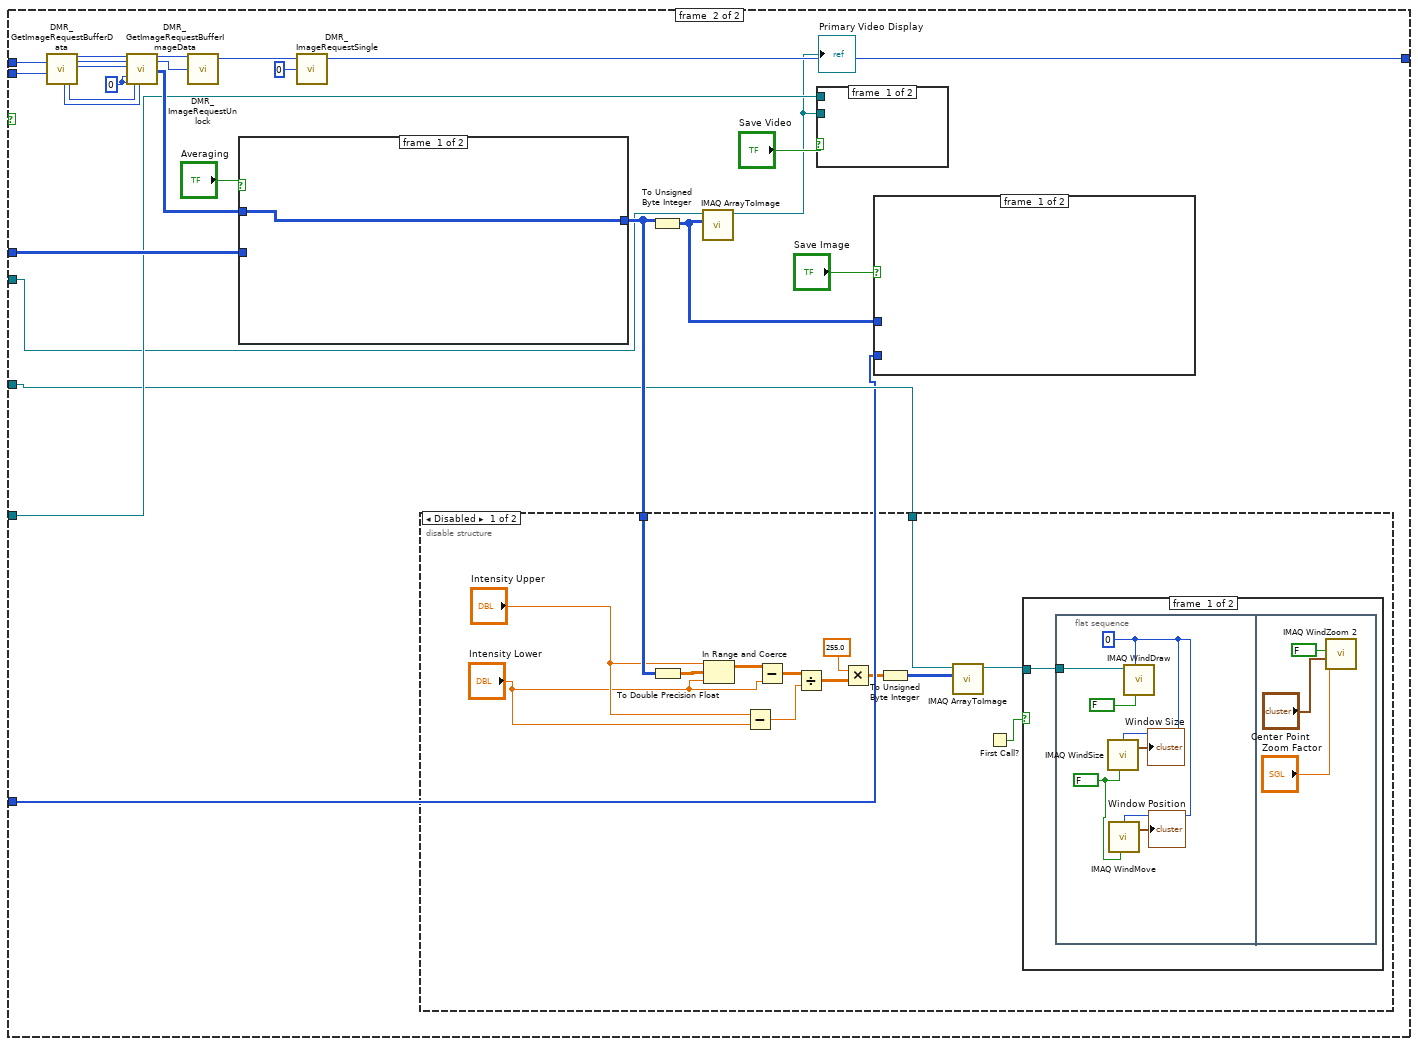
[diagram p13: hidden frame]
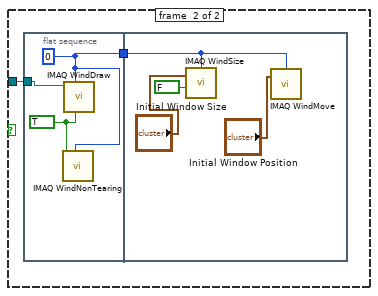
[diagram p14: hidden frame]
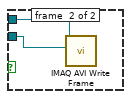
[diagram p16: hidden frame]
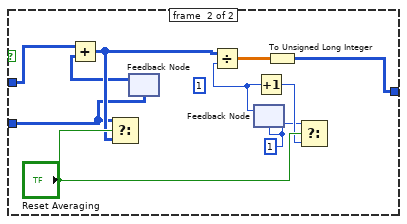
[diagram p17: hidden frame]
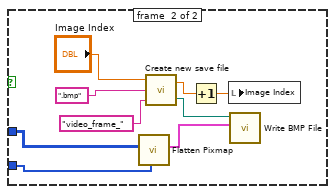
[diagram p18: hidden frame]
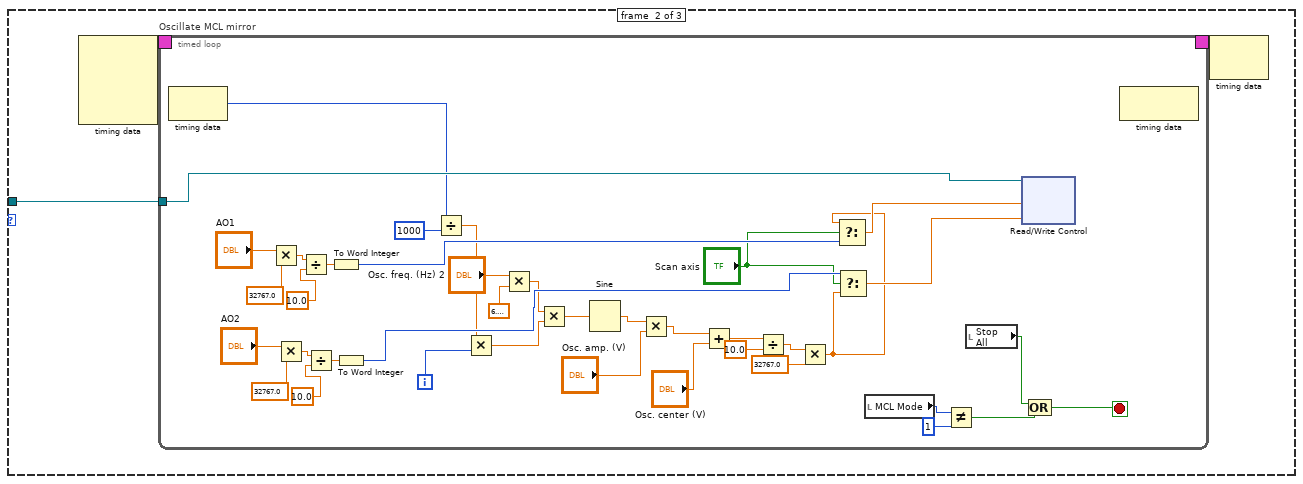
[diagram p19: hidden frame]
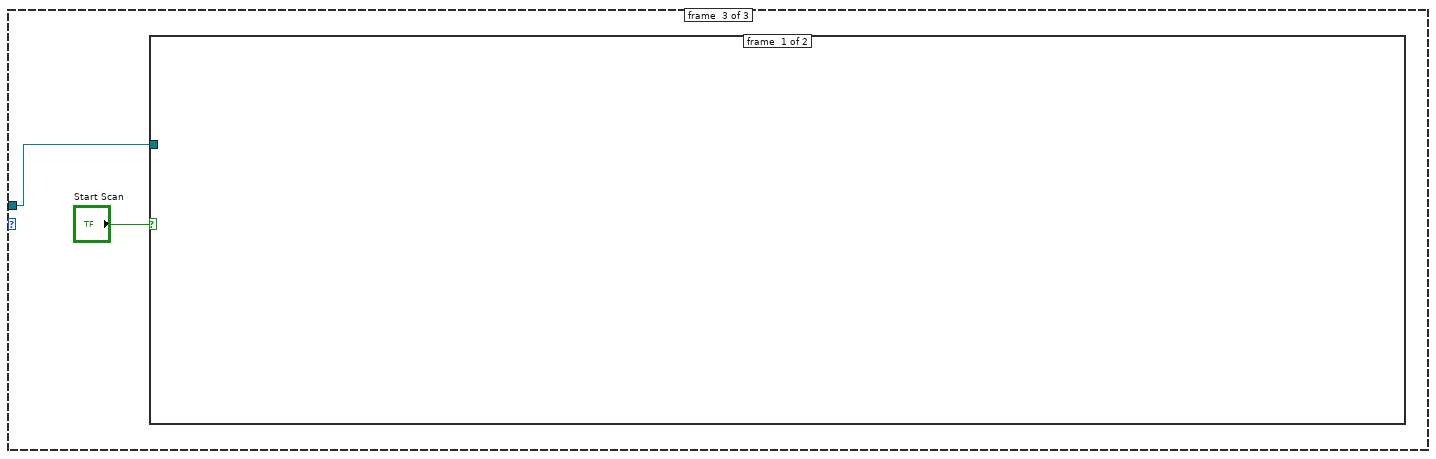
[diagram p20: hidden frame]
diagram:
  w10 = T12 2 items=["Grayscale (U8)", "Grayscale (I16)", "Grayscale (SGL)", "Complex (CSG)", "RGB (U32)", "HSL (U32)", "RGB (U64)", "Grayscale (U16)"] ("Image Type")
  w69 = cluster{"output high":i16, "output low":i16} {"output high"=3000, "output low"=0} ("FB output range 1")
  w75 = TRUE ("AI to FIFO")
  w160 = 10.0 ("y")
  w159 = 32767.0 ("y")
  w175 = 6.0  # clock mult.
  w176 = 49152000.0  # TCXO frequ.
  n1 = Build Array("DIO count 1 (ticks)", "DIO count 2 (ticks)", "DIO count 3 (ticks)") -> (w56:u32[])
  n2 = Multiply(x="APD Integration Time (s)", y=40000000.0) -> (x*y=w83:dbl)
  n3 = Reciprocal(x="APD Integration Time (s)") -> (1/x=w80:dbl)
  n4 = local write "APD Acq Rate (Hz)"(w80) -> ()
  n5 = local read "AO1"() -> (w154:dbl)
  n6 = local read "AO2"() -> (w153:dbl)
  n7 = To Unsigned Long Integer(number=w83) -> (unsigned 32bit integer=w82:u32)
  "APD Int. Count" <- w82
  n8 = local read "Scan Increment (MHz)"() -> (w171:dbl)
  n9 = local read "Continuous MCL Scanning"() -> (w141:bool)
  n10 = local read "Fast Scan Dir"() -> (w140:bool)
  n11 = Multiply(x=w154, y=w159) -> (x*y=w156:dbl)
  n12 = local read "Number of scans (MCL)"() -> (w142:u64)
  n13 = Multiply(x=w153, y=w159) -> (x*y=w158:dbl)
  n14 = Divide(x=w156, y=w160) -> (x/y=w155:dbl)
  n15 = Divide(x=w158, y=w160) -> (x/y=w157:dbl)
  n16 = To Word Integer(number=w155) -> (16bit integer=w152:i16)
  n17 = To Word Integer(number=w157) -> (16bit integer=w151:i16)
  n18 = Not(x=w140) -> (.not. x?=w135:bool)
  n19 = local read "Cycles/step (MCL)"() -> (w143:u64)
  n20 = Multiply(x=w171, y=1000.0) -> (x*y=w178:dbl)
  n21 = local read "Scan steps (MCL)"() -> (w144:u64)
  n22 = local read "Desired Scan Incr (V)"() -> (w146:dbl)
  n23 = Scale By Power Of 2(n=48, x=w178) -> (x*2^n=w179:dbl)
  n24 = Multiply(x=w176, y=w175) -> (x*y=w174:dbl)
  n25 = Divide(x=w179, y=w174) -> (x/y=w173:dbl)
  n26 = local read "Setpoints (V)"() -> (w196:cluster{"Set 1":dbl, "Set 2":dbl})
  n27 = property on="AI Count (ticks)" class="DigNum (strict)"("Val(Sgnl)"="AI Count (ticks)") -> ()  [unwired: 2 in, 2 out]
  n28 = local read "Number Interlace Sets"() -> (w49:u8)
  n29 = Split 1D Array(array=w56, index=w49) -> (first subarray=w58:u32[])  [unwired: 1 out]
  n30 = Add Array Elements(numeric array=w58) -> (sum=w57:u32)
  n31 = local read "# Samples/channel"() -> (w163:u32)
  n32 = To Quad Integer(1:w173) -> (0:w170:i64)
  n33 = local read "Sets to FIFO (Traps)"() -> (w203:T10)
  n34 = local read "Number of F/B Scans (AOD)"() -> (w164:u16)
  n35 = local read "Not-Interlacing Set"() -> (w48:enum32{"Set 1", "Set 2", "Set 3"})
  n36 = To Unsigned Byte Integer(number=w48) -> (unsigned 8bit integer=w54:u8)
  n37 = Index Array(array=w56, index=w54) -> (element=w55:u32)
  n38 = Divide(x=40000000.0, y="AI Count (ticks)") -> (x/y=w131:dbl)
  n39 = Multiply(x=w146, y=32767.0) -> (x*y=w148:dbl)
  n40 = local read "Feedback On/Off"() -> (w199:cluster{"Set 1":bool, "Set 2":bool})
  n41 = local read "PID Gains"() -> (w191:T8)
  n42 = local read "Scan steps (AOD)"() -> (w169:u64)
  n43 = local read "All FB On/Off"() -> (w200:bool)
  n44 = local read "Cycles/step (AOD)"() -> (w168:u64)
  n45 = local write "AI rate (Hz)"(w131) -> ()
  n46 = Divide(x=w148, y=10.0) -> (x/y=w147:dbl)
  n47 = Multiply(x=w169, y=w168) -> (x*y=w167:u64)
  n48 = Multiply(x=3276.7, y=w196) -> (x*y=w195:cluster{"Set 1":dbl, "Set 2":dbl})
  n49 = To Word Integer(number=w147) -> (16bit integer=w145:i16)
  n50 = Multiply(x=w167, y=u64 2) -> (x*y=w165:u64)
  n51 = Divide(x=w131, y="FPGA Ave.") -> (x/y=w132:dbl)
  n52 = To Word Integer(number=w195) -> (16bit integer=w194:cluster{"Set 1":i16, "Set 2":i16})
  n53 = xnode "Open FPGA VI Reference"("resource name"=T13 "750kHzDAQ") -> ("FPGA VI Reference Out"=w186:T14, "error out"=w185:errorcluster)  [unwired: 1 in]
  n54 = Unbundle By Name(w191) -> ("Set 1"=w190:T9, "Set 2"=w189:T9)
  n55 = Multiply(x=w165, y=w164) -> (x*y=w162:u64)
  n56 = Divide(x=w162, y=w163) -> (x/y=w161:dbl)
  n57 = local write "Ave. Rate (Hz)"(w132) -> ()
  n58 = Unbundle By Name(w194) -> ("Set 1"=w193:i16, "Set 2"=w192:i16)
  n59 = local read "2D or 1D Scan"() -> (w72:bool)
  n60 = local write "Data points/scans"(w162) -> ()
  n61 = And(x=w199, y=w200) -> (x .and. y?=w198:cluster{"Set 1":bool, "Set 2":bool})
  n62 = local read "Scan BD"() -> (w180:bool)
  n63 = Reciprocal(x=w132) -> (1/x=w133:dbl)
  n64 = local write "Data points/scan (f/b)"(w165) -> ()
  n65 = local read "N Acq Sets (Traps + Fl.)"() -> (w124:i16)
  n66 = local write "N sets should be saved"(w161) -> ()
  n67 = Unbundle By Name(w198) -> ("Set 1"=w202:bool, "Set 2"=w201:bool)
  n68 = xnode "Invoke Method"("FPGA VI Reference In"=w186, "error in"=w185) -> ("FPGA VI Reference Out"=w68:T14, "error out"=w98:errorcluster)
  n69 = local read "Interlace"() -> (w50:bool)
  n70 = Select(t=w57, s=w50, f=w55) -> (s? t:f=w47:u32)
  n71 = local write "Update Count (MCL)"(w47) -> ()
  n72 = local write "Total Counts (ticks)"(w47) -> ()
  n73 = local write "Ave. Period (s)"(w133) -> ()
  n74 = property on="2D or 1D Scan" class="Bool (strict)"("Val(Sgnl)"=w72) -> ()  [unwired: 2 in, 2 out]
  n75 = xnode "Read/Write Control"("FPGA VI Reference In"=w67, "error in"=w98, "ai count"="AI Count (ticks)", "AI Averages"="FPGA Ave.", "DMA buffer timeout"=0, "AI to FIFO"=FALSE, "Interlace ON/OFF"=w50, "Number Interlace Cycles"=w49, "AI1 Sets to FIFO"=w203, "FB On/Off Set 1"=w202, "FB On/Off Set 2"=w201, "Interlace Off Parameters"=w48, "FB Setpoint Set 1"=w193, "FB Setpoint Set 2"=w192, "FB Gains Set 1"=w190, "FB Gains Set 2"=w189, "FB output range 1"=w69, "FB output range 2"=w69, "Cycles per step"=w168, "Scan BD"=w180, "Number of scans"=w164, "Scan steps"=w169, "Scan freq.  increment"=w170, "AO1"=w152, "AO2"=w151, "Scan freq.  increment (MCL)"=w145, "Scan steps (MCL)"=w144, "Cycles per step (MCL)"=w143, "Number of scans (MCL)"=w142, "MCL count"=w47, "Cont. Scan (MCL)"=w141, "MCL Scan Axis"=w135, "1D or 2D Scan?"=w72, "N of AI1 Int Acq Sets"=w124, "Freq or Amp switch first"="Freq or Amp switch first", "Freq switch delay"="Freq switch delay", "Amp switch delay"="Amp switch delay", "Swap F1 and F2"="Swap F1 and F2", "APD Acq Rate Count"=w82, "APD to FIFO"=FALSE, "APD Gate Operating Mode"="APD Gate", "APD Gate ON Count"="APD Gate ON Count", "APD Gate OFF Count"="APD Gate OFF Count", "Invert APD Gate"="Invert APD Gate", "DIO count 1 (ticks)"="DIO count 1 (ticks)", "DIO count 2 (ticks)"="DIO count 2 (ticks)", "DIO count 3 (ticks)"="DIO count 3 (ticks)", "APD 1 AO scale factor"="APD 1 AO Mult.", "APD 2 AO scale factor"="APD 2 AO Mult.", "APD 1 AO offset"="APD 1 AO offset", "APD 2 AO offset"="APD 2 AO offset") -> ("FPGA VI Reference Out"=w42:T14, "error out"=w44:errorcluster)
  n76 = local read "Green Laser ON/Interlacing"() -> (w45:bool)
  n77 = local read "GI Frequency, OFF count"() -> (w38:u32)
  n78 = local read "GI Frequency, ON count"() -> (w37:u32)
  n79 = Multiply(x="Current When FB OFF (%)", y=655.35) -> (x*y=w28:dbl)
  n80 = local read "Green laser mode"() -> (w46:enum32{"Laser ON", "Laser OFF", "Interlace"})
  n81 = local read "Green FB Count"() -> (w36:u32)
  n82 = To Unsigned Word Integer(number=w28) -> (unsigned 16bit integer=w26:u16)
  n83 = local read "Invert GI"() -> (w40:bool)
  n84 = Multiply(x="Green FB Setpoint (mV)", y=3.2767) -> (x*y=w25:dbl)
  n85 = case shown="False" w45 {
    tunnel: w46 -> [_ w230]
    tunnel: [enum32{"Laser ON", "Laser OFF", "Interlace"}."Laser OFF" ("Green laser mode") w230] -> w39
    frame #0 {
    }
    frame #1 {
    }
  }
  n86 = To Word Integer(number=w25) -> (16bit integer=w23:i16)
  n87 = xnode "Read/Write Control"("FPGA VI Reference In"=w42, "error in"=w44, "Green interlace ON count 2"=w37, "Green interlace OFF count 2"=w38, "Invert GI 2"=w40, "Operating Mode 2"=w39, "Green FB Gains"="Green FB Gains", "Green FB Setpoint"=w23, "Green FB On/Off"="Green FB On/Off", "Current Out"=w26, "Green int current ON count adj"="Green int current ON count adj", "Green FB Count"=w36, "Operating Mode"=w39, "Green interlace OFF count"=w38, "Green interlace ON count"=w37, "Invert GI"=w40) -> ("FPGA VI Reference Out"=w41:T14, "error out"=w43:errorcluster)
  n88 = flat-sequence {
    tunnel: w68 -> [w235]
    tunnel: [w235] -> w67
    tunnel: [w234] -> w66
    tunnel: [w233] -> w65
    tunnel: [w231] -> w63
    tunnel: [w232] -> w64
    frame #0 {
      w232 = T11 {"Minimum"=0.0, "Maximum"=40.0, "Increment"=1.0} ("Min Max Inc")
      w231 = T11 {"Minimum"=0.0, "Maximum"=50.0, "Increment"=1.0} ("Data Entry Limits")
      w234 = T11 {"Minimum"=60.0, "Maximum"=90.0, "Increment"=1.0} ("Min Max Inc")
      w233 = T11 {"Minimum"=0.0, "Maximum"=50.0, "Increment"=1.0} ("Data Entry Limits")
      n89 = property on="BD 2 Frequency 1 (MHz)" class="DigNum (strict)"("Data Range"=w232) -> ()  [unwired: 2 in, 2 out]
      n90 = property on="BD 2 Frequency 3 (MHz)" class="DigNum (strict)"("Data Range"=w232) -> ()  [unwired: 2 in, 2 out]
      n91 = property on="BD 2 Frequency 2 (MHz)" class="DigNum (strict)"("Data Range"=w232) -> ()  [unwired: 2 in, 2 out]
      n92 = property on="BD 1 Frequency 1 (MHz)" class="DigNum (strict)"("Data Range"=w234) -> ()  [unwired: 2 in, 2 out]
      n93 = property on="BD 1 Frequency 2 (MHz)" class="DigNum (strict)"("Data Range"=w234) -> ()  [unwired: 2 in, 2 out]
      n94 = property on="BD 1 Frequency 3 (MHz)" class="DigNum (strict)"("Data Range"=w234) -> ()  [unwired: 2 in, 2 out]
      n95 = property on="BD 2 Amplitude 1 (%)" class="DigNum (strict)"("Data Range"=w231) -> ()  [unwired: 2 in, 2 out]
      n96 = property on="BD 2 Amplitude 2 (%)" class="DigNum (strict)"("Data Range"=w231) -> ()  [unwired: 2 in, 2 out]
      n97 = property on="BD 2 Amplitude 3 (%)" class="DigNum (strict)"("Data Range"=w231) -> ()  [unwired: 2 in, 2 out]
      n98 = property on="BD 1 Amplitude 3 (%)" class="DigNum (strict)"("Data Range"=w233) -> ()  [unwired: 2 in, 2 out]
      n99 = property on="BD 1 Amplitude 2 (%)" class="DigNum (strict)"("Data Range"=w233) -> ()  [unwired: 2 in, 2 out]
      n100 = property on="BD 1 Amplitude 1 (%)" class="DigNum (strict)"("Data Range"=w233) -> ()  [unwired: 2 in, 2 out]
      "X RF Frequency Limits (MHz)" <- w234
      "X RF Amplitude Limits (%)" <- w233
      "Y RF Amplitude Limits (%)" <- w231
      "Y RF Frequency Limits (MHz)" <- w232
    }
  }
  n101 = xnode "Invoke Method"("FPGA VI Reference In"=w41, "error in"=w43, "Depth"="FIFO Depth") -> ("FPGA VI Reference Out"=w188:T14, "error out"=w187:errorcluster)
  n102 = xnode "Invoke Method"("FPGA VI Reference In"=w188, "error in"=w187) -> ("FPGA VI Reference Out"=w97:T14, "error out"=w96:errorcluster)
  n103 = xnode "Invoke Method"("FPGA VI Reference In"=w97, "error in"=w96) -> ("FPGA VI Reference Out"=w95:T14, "error out"=w94:errorcluster)  [unwired: 1 out]
  n104 = flat-sequence "Initial FPGA Loop Relative Phase Adjustment" {
    tunnel: "Initial Phase Adjustment (AI1)" -> [w245]
    tunnel: "Initial Phase Adjustment (GI)" -> [w244]
    tunnel: w95 -> [w243]
    tunnel: w94 -> [w242]
    tunnel: "Initial Phase Adj. (MCL)" -> [w241]
    tunnel: [w246] -> w106
    tunnel: [w240] -> w102
    tunnel: "Initial Phase Adjustment (APD Acq)" -> [w239]
    tunnel: "Initial Phase Adjustment (APD Gate)" -> [w238]
    tunnel: "Initial Phase Adjustment (Green FB)" -> [w237]
    tunnel: "Initial Phase Adjustment (GI) 2" -> [w236]
    tunnel: w106 -> [w398]
    tunnel: [w399] -> w103
    tunnel: w102 -> [w399]
    tunnel: [w398] -> w101
    tunnel: w103 -> [w402]
    tunnel: w101 -> [w401]
    tunnel: [w404] -> w100
    tunnel: [w403] -> w99
    tunnel: [w563] -> w104
    tunnel: [w564] -> w105
    tunnel: w100 -> [w564]
    tunnel: w99 -> [w563]
    frame #0 {
      n105 = xnode "Read/Write Control"("FPGA VI Reference In"=w243, "error in"=w242, "Phase count adjustment"=w245, "Phase count adjustment (GI)"=w244, "Phase count adjustment (MCL)"=w241, "Phase Count Adjustment (APD Acq)"=w239, "Phase count adjustment (APD Gate)"=w238, "Phase count adjustment (Green FB)"=w237, "Phase count adjustment (GI) 2"=w236) -> ("FPGA VI Reference Out"=w240:T14, "error out"=w246:errorcluster)
    }
    frame #1 {
      n106 = Wait (ms)(milliseconds to wait=u32 1000) -> ()  [unwired: 1 out]
    }
    frame #2 {
      w400 = TRUE
      n107 = xnode "Read/Write Control"("FPGA VI Reference In"=w402, "error in"=w401, "+ phase"=w400, "+ phase (GI)"=w400, "+ phase (MCL)"=w400, "+ phase (APD Acq)"=w400, "+ phase (APD Gate)"=w400, "+ phase (Green FB)"=w400, "+ phase (GI) 2"=w400) -> ("FPGA VI Reference Out"=w403:T14, "error out"=w404:errorcluster)
    }
    frame #3 {
      n108 = Wait (ms)(milliseconds to wait=u32 1000) -> ()  [unwired: 1 out]
    }
  }
  n109 = local read "Phase adj. (Green FB)"() -> (w59:i16)
  n110 = local read "Phase adj. (GI) 2"() -> (w29:i16)
  n111 = local read "Phase adjust (MCL)"() -> (w136:i16)
  n112 = local read "Phase adj. (AI1)"() -> (w138:i16)
  n113 = local read "Phase adj. (GI)"() -> (w137:i16)
  n114 = xnode "Read/Write Control"("FPGA VI Reference In"=w104, "error in"=w105, "Phase count adjustment"=w138, "Phase count adjustment (GI)"=w137, "Phase count adjustment (MCL)"=w136, "Phase Count Adjustment (APD Acq)"="Phase Adj. (APD Acq)", "Phase count adjustment (APD Gate)"="Phase Adj. (APD Gate)", "Phase count adjustment (Green FB)"=w59, "Phase count adjustment (GI) 2"=w29) -> ("FPGA VI Reference Out"=w15:T14, "error out"=w113:errorcluster)
  n115 = call "Initialize RF boards - interlace 3.vi"("error in"=w113, "FPGA VI Reference In"=w15) -> ("error out"=w111:errorcluster, "FPGA VI Reference Out"=w112:T14)
  n116 = call "set RF board frequency - interlace.vi"("Board 2 Frequency Limits"=w64, "Board 1 Frequency Limits"=w66, "error in"=w111, "FPGA VI Reference In"=w112, "Board 2 Frequency 3 (MHz)"="BD 2 Frequency 3 (MHz)", "Board 1 Frequency 3 (MHz)"="BD 1 Frequency 3 (MHz)", "Board 2 Frequency 2 (MHz)"="BD 2 Frequency 2 (MHz)", "Board 2 Frequency 1 (MHz)"="BD 2 Frequency 1 (MHz)", "Board 1 Frequency 2 (MHz)"="BD 1 Frequency 2 (MHz)", "Board 1 Frequency 1  (MHz)"="BD 1 Frequency 1 (MHz)") -> ("error out"=w219:errorcluster, "FPGA VI Reference Out"=w220:T14)
  n117 = call "set RF board amplitude - interlace.vi"("Board 2 Amplitude Limits"=w63, "Board 1 Amplitude Limits"=w65, "error in"=w219, "FPGA VI Reference In"=w220, "Board 2 Amplitude 3 (%)"="BD 2 Amplitude 3 (%)", "Board 1 Amplitude 3 (%)"="BD 1 Amplitude 3 (%)", "Board 2 Amplitude 2 (%)"="BD 2 Amplitude 2 (%)", "Board 2 Amplitude 1 (%)"="BD 2 Amplitude 1 (%)", "Board 1 Amplitude 2 (%)"="BD 1 Amplitude 2 (%)", "Board 1 Amplitude 1 (%)"="BD 1 Amplitude 1 (%)") -> ("error out"=w207:errorcluster, "FPGA VI Reference Out"=w208:T14)
  n118 = flat-sequence {
    tunnel: w208 -> [w573]
    tunnel: w207 -> [w572]
    tunnel: [w571] -> w212
    tunnel: [w570] -> w211
    tunnel: [w614] -> w210
    tunnel: w212 -> [w614]
    tunnel: [w613] -> w209
    tunnel: w211 -> [w613]
    tunnel: w210 -> [w622]
    tunnel: w209 -> [w621]
    tunnel: [w620] -> w77
    tunnel: [w619] -> w76
    frame #0 {
      n119 = local read "Trap 1 (ON/OFF)"() -> (w565:bool)
      n120 = xnode "Read/Write Control"("FPGA VI Reference In"=w573, "error in"=w572, "Direct RF Box  Communication"=FALSE) -> ("FPGA VI Reference Out"=w571:T14, "error out"=w570:errorcluster)
      n121 = local write "Saving..."(FALSE ("Saving Data")) -> ()
      n122 = local write "Stop All"(FALSE ("Stop All")) -> ()
      n123 = local write "Index"(1.0 ("Index")) -> ()
      n124 = property on="Trap 1 ON" class="Bool (strict)"("Value"=w565) -> ()  [unwired: 2 in, 2 out]
      "Manipulating Trap" <- FALSE ("Manipulating Trap")
    }
    frame #1 {
      n125 = local read "Trap 2 (ON/OFF)"() -> (w612:bool)
      n126 = Wait (ms)(milliseconds to wait=u32 10) -> ()  [unwired: 1 out]
      n127 = property on="Trap 2 ON" class="Bool (strict)"("Val(Sgnl)"=w612) -> ()  [unwired: 2 in, 2 out]
    }
    frame #2 {
      n128 = xnode "Read/Write Control"("FPGA VI Reference In"=w622, "error in"=w621, "FPGA Controls  RF Box"=TRUE ("Direct RF Box  Communication")) -> ("FPGA VI Reference Out"=w620:T14, "error out"=w619:errorcluster)
      n129 = call "Update messages.vi"("Message to add"="UHR-Fleezers ready.", "Old message string"="") -> ("New message string"=w618:string)
      n130 = local write "Messages"(w618) -> ()
    }
  }
  n131 = Subtract(x="BD 1 Frequency 1 (MHz)", y="BD 1 Frequency 2 (MHz)") -> (x-y=w123:dbl)
  n132 = Subtract(x="BD 2 Frequency 1 (MHz)", y="BD 2 Frequency 2 (MHz)") -> (x-y=w122:dbl)
  n133 = Square(x=w122) -> (x^2=w120:dbl)
  n134 = Square(x=w123) -> (x^2=w121:dbl)
  n135 = Add(x=w121, y=w120) -> (x+y=w119:dbl)
  n136 = Square Root(x=w119) -> (sqrt(x)=w118:dbl)
  n137 = local write "Trap Delta (MHz)"(w118) -> ()
  n138 = xnode "Read/Write Control"("FPGA VI Reference In"=w77, "error in"=w76, "AI to FIFO"=w75, "APD to FIFO"=w75) -> ("FPGA VI Reference Out"=w74:T14, "error out"=w73:errorcluster)
  n139 = call "IMAQ Create"("Image Name"="Det. Y Image", "Image Type"=w10) -> ("New Image"=w8:T1)  [unwired: 3 in, 1 out]
  n140 = call "IMAQ Create"("Image Name"="Det. X Image", "Image Type"=w10) -> ("New Image"=w9:T1)  [unwired: 3 in, 1 out]
  n141 = call "IMAQ Create"("Image Name"="APD1 Image", "Image Type"=w10) -> ("New Image"=w13:T1)  [unwired: 3 in, 1 out]
  n142 = call-poly "VISA Configure Serial Port"("VISA resource name"="Sample Chamber Stage Serial Port") -> ("VISA resource name out"=w6:refnum<visa-resource-name>, "error out"=w7:errorcluster)  [unwired: 5 in, 8 out]
  "Stage Control Serial Error" <- w7
  n143 = node-c288() -> (w19:T17)  [unwired: 4 out]
  n144 = node-c288() -> (w21:T17)  [unwired: 4 out]
  n145 = node-c288() -> (w2:T17)  [unwired: 4 in]
  n146 = timed-loop "Control parameters (event loop)" {
    tunnel: w77 -> [w664]
    shift-right: [w663] -> _
    shift-left: errorcluster {"status"=FALSE, "code"=0, "source"=""} ("error out") -> [w662]
    tunnel: [w661] -> w181
    timing: w19 -> [_]
    timing-out: [_] -> w18
    stop <- w661 stop-if-true
    n147 = node-c288() -> ()  [unwired: 2 out]
    n148 = event shown="[5] \"BD 1 Frequency 1 (MHz)\", \"BD 1 Frequency 2 (MHz)\", \"BD 1 Frequency 3 (MHz)\", \"BD 2 Frequency 1 (MHz)\", \"BD 2 Frequency 2 (MHz)\", \"BD 2 Frequency 3 (MHz)\", \"Trap Delta (MHz)\": Value Change" {
      selector: _ -> [_ _ _ _ _ _ _ _ _ _ _ _ _ _ _ _ _ _ _ _ _ _ _ _ _ _ _ _ _ _ _ _ _ _ _ _ _ _ _ _ _ _]
      dyn-events: _ -> [_ _ _ _ _ _ _ _ _ _ _ _ _ _ _ _ _ _ _ _ _ _ _ _ _ _ _ _ _ _ _ _ _ _ _ _ _ _ _ _ _ _]
      timeout: _ -> [_ _ _ _ _ _ _ _ _ _ _ _ _ _ _ _ _ _ _ _ _ _ _ _ _ _ _ _ _ _ _ _ _ _ _ _ _ _ _ _ _ _]
      tunnel: w664 -> [w705 _ _ w832 _ w927 _ _ _ _ w993 _ _ w1093 w1231 w1293 w1336 w1486 w1561 w1672 w1765 w1849 w1933 w2017 w2101 w2194 w2389 w2589 w2682 w2815 _ w2985 w3026 w3073 w3150 w3191 _ w3236 _ _ _ w3384]
      tunnel: [w704 _ _ w822 _ w926 _ _ w958 _ w972 _ _ w1092 w1227 w1290 w1333 w1485 w1559 w1671 w1759 w1843 w1927 w2011 w2095 w2192 w2388 w2587 w2680 w2813 _ w2983 w3024 w3063 w3148 w3189 _ w3234 _ _ _ w3382] -> w663
      tunnel: w662 -> [w703 _ _ w831 _ w925 _ _ w958 _ w992 _ _ w1091 w1226 w1289 w1332 w1484 w1560 w1670 w1764 w1848 w1932 w2016 w2100 w2193 w2387 w2588 w2681 w2814 _ w2984 w3025 w3072 w3149 w3190 _ w3235 _ _ _ w3383]
      tunnel: [_ _ _ _ _ _ _ _ w957 _ _ _ _ _ _ _ _ _ _ _ _ _ _ _ _ _ _ _ _ _ _ _ _ _ _ _ _ _ _ _ _ _] -> w661
      tunnel: [_ _ _ _ _ _ "Round T1 X" _ _ _ _ "Load parameters" _ _ _ _ _ _ _ _ _ _ _ _ _ _ _ _ _ _ _ _ _ _ _ _ _ _ _ _ _ _] -> _
      tunnel: [_ _ "Adjust Scale\nto Mean" _ _ _ _ _ _ _ _ _ _ _ _ _ _ _ _ _ _ _ _ _ _ _ _ _ _ _ _ _ _ _ _ _ _ _ _ _ _ _] -> _
      tunnel: [_ _ _ _ _ _ _ "Round T2 X" _ "Delayed Interlace Start" _ _ _ _ _ _ _ _ _ _ _ _ _ _ _ _ _ _ _ _ _ _ _ _ _ _ _ _ _ _ _ _] -> _
      tunnel: [_ "Rescale on Mean" _ _ _ _ _ _ _ _ _ _ _ _ _ _ _ _ _ _ _ _ _ _ _ _ _ _ _ _ _ _ _ _ _ _ _ _ _ _ _ _] -> _
      tunnel: [_ _ _ _ _ _ _ _ _ _ _ _ _ _ _ _ _ _ _ _ _ _ _ _ _ _ _ _ _ _ _ _ _ _ _ _ _ _ _ _ _ "Flip Green Filter"] -> _
      event #0 {
        # "So that if 'Save ave N' is updated, the AOD scanning code updates too."
        n149 = event-data() -> ()  [unwired: 6 out]
        n150 = local read "AI Count (ticks)"() -> (w675:u32)
        n151 = local read "FPGA Ave."() -> (w679:dbl)
        n152 = Boolean To (0,1)(Boolean="Sets to FIFO (Traps)") -> (0, 1=w693:cluster{"Set 1":i16, "Set 2":i16, "Set 3":i16})
        n153 = xnode "Read/Write Control"("FPGA VI Reference In"=w705, "error in"=w703, "ai count"=w675, "AI1 Sets to FIFO"="Sets to FIFO (Traps)", "AI Averages"=w679, "N of AI1 Int Acq Sets"="N Acq Sets (Traps + Fl.)") -> ("error out"=w704:errorcluster)  [unwired: 1 out]
        n154 = Cluster To Array(cluster=w693) -> (array=w692:i16[])
        n155 = local read "Scan steps (AOD)"() -> (w694:u64)
        n156 = Multiply(x=w675, y="N Acq Sets (Traps + Fl.)") -> (x*y=w673:u32)
        n157 = Divide(x=40000000.0, y=w675) -> (x/y=w701:dbl)
        "AI rate (Hz)" <- w701
        n158 = Add Array Elements(numeric array=w692) -> (sum=w677:i16)
        "Trap Sets" <- w677
        n159 = Divide(x=w701, y=w679) -> (x/y=w702:dbl)
        "Ave. Rate (Hz)" <- w702
        n160 = Reciprocal(x=w702) -> (1/x=→"Ave. Period (s)":dbl)
        n161 = property on="Scan steps (AOD)" class="DigNum (strict)"("Val(Sgnl)"=w694) -> ()  [unwired: 2 in, 2 out]
        n162 = Divide(x=w702, y="N Acq Sets (Traps + Fl.)") -> (x/y=w698:dbl)
        "Data Rate (Hz)" <- w698
        n163 = Reciprocal(x=w698) -> (1/x=→"Data Period (s)":dbl)
        n164 = local read "Save ave N"() -> (w697:dbl)
        n165 = Divide(x=w698, y=w697) -> (x/y=w696:dbl)
        "Save Data Rate (Hz)" <- w696
        n166 = Reciprocal(x=w696) -> (1/x=→"Save Data Period (s)":dbl)
        n167 = Multiply(x=w673, y="# Samples/trap") -> (x*y=w669:dbl)
        "Counts/DMA" <- w669
        n168 = Multiply(x=w677, y="# Samples/trap") -> (x*y=w676:dbl)
        "# Samples/channel" <- w676
        n169 = Greater?(x=w679, y=1.0) -> (0:w682:bool)
        "FPGA Averaging" <- w682
        n170 = local read "APD Int. Count"() -> (w671:u32)
        n171 = Divide(x=w676, y=u32 2) -> (x/y=w685:dbl)
        n172 = Select(t=w676, s=w682, f=w685) -> (s? t:f=w690:dbl)
        n173 = Divide(x=w669, y=w671) -> (x/y=w670:dbl)
        "APD Samples/FIFO Acq." <- w670
        n174 = Divide(x=w669, y=40000000.0) -> (x/y=w667:dbl)
        "DMA Update Period (s)" <- w667
        n175 = Multiply(x=w690, y=u32 8) -> (x*y=→"Elements/DMA read":dbl)
        n176 = Multiply(x=2.0, y=w670) -> (x*y=→"APD Elements/DMA read":dbl)
        n177 = local read "N sets to save"() -> (w687:u32)
        n178 = Multiply(x=w667, y=w687) -> (x*y=→"Total Time (s)":dbl)
      }
      event #1 {
        n179 = event-data() -> ()  [unwired: 7 out]
        n180 = local read "Bead Mean (nm)"() -> (w810:dbl)
        n181 = Add(x="Amplitude (nm)", y=w810) -> (x+y=w808:dbl)
        n182 = Subtract(x=w810, y="Amplitude (nm)") -> (x-y=w807:dbl)
        n183 = property on="Bead Separation" class="WFChart (strict)"("YScale.Minimum"=w807) -> ()  [unwired: 2 in, 2 out]
        n184 = property on="Bead Separation" class="WFChart (strict)"("YScale.Maximum"=w808) -> ()  [unwired: 2 in, 2 out]
      }
      event #2 {
        n185 = event-data() -> ()  [unwired: 7 out]
        n186 = local read "APD 1 Rate (Hz)"() -> (w819:dbl)
        n187 = Multiply(x=1000.0, y="Above (kHz)") -> (x*y=w817:dbl)
        n188 = Multiply(x=1000.0, y="Below (kHz)") -> (x*y=w815:dbl)
        n189 = Add(x=w817, y=w819) -> (x+y=w812:dbl)
        n190 = Subtract(x=w819, y=w815) -> (x-y=w813:dbl)
        n191 = property on="APD 1 Chart" class="WFChart (strict)"("YScale.Minimum"=w813) -> ()  [unwired: 2 in, 2 out]
        n192 = property on="APD 1 Chart" class="WFChart (strict)"("YScale.Maximum"=w812) -> ()  [unwired: 2 in, 2 out]
      }
      event #3 {
        n193 = event-data() -> ()  [unwired: 7 out]
        n194 = Negate(x="Phase adj. (AI1)") -> (-x=w829:i16)
        n195 = Select(t=w829, s="- phase (AI1)", f="Phase adj. (AI1)") -> (s? t:f=w828:i16)
        n196 = xnode "Read/Write Control"("FPGA VI Reference In"=w832, "error in"=w831, "Phase count adjustment"=w828) -> ("FPGA VI Reference Out"=w827:T14, "error out"=w826:errorcluster)
        n197 = Or(x="- phase (AI1)", y="+ phase (AI1)") -> (x .or. y?=w823:bool)
        n198 = xnode "Read/Write Control"("FPGA VI Reference In"=w827, "error in"=w826, "+ phase"=w823) -> ("error out"=w822:errorcluster)  [unwired: 1 out]
      }
      event #4 {
        w908 = u32 9868950 ("Color Box")
        n199 = event-data() -> ("Row"=w910:i32)  [unwired: 9 out]
        n200 = property on="All Signals" class="WFChart (strict)"("Active Plot"=w910) -> (error out=w921:errorcluster)  [unwired: 2 in, 1 out]
        n201 = property on="All Signals" class="WFChart (strict)" props=["Plot", "Visible?", "Plot", "Plot Color"](error in=w921) -> (error out=w920:errorcluster, "Plot.Visible?"=w919:bool)  [unwired: 1 in, 2 out]
        n202 = Select(t=FALSE ("Plot.Visible"), s=w919, f=TRUE ("Plot.Visible")) -> (s? t:f=w914:bool)
        n203 = property on="All Signals" class="WFChart (strict)"(error in=w920, "Plot.Visible?"=w914) -> (error out=w916:errorcluster)  [unwired: 1 in, 1 out]
        n204 = property on="All Signals" class="WFChart (strict)"(error in=w916) -> (error out=w911:errorcluster, "Plot.Plot Color"=w915:u32)  [unwired: 1 in, 1 out]
        n205 = property on="Signals to Plot" class="LstBox (strict)"(error in=w911, "Active Row"=w910) -> (error out=w909:errorcluster)  [unwired: 1 in, 1 out]
        n206 = Select(t=w915, s=w914, f=u32 0) -> (s? t:f=w912:u32)
        n207 = property on="Signals to Plot" class="LstBox (strict)"(error in=w909, "CellFontColor"=w912, "SelColor"=w908, "CellBG"=w908, "CellFontSize"=u32 20 ("Active Row:Cell Font:Size"), "CellFontBold"=TRUE ("Active Row:Cell Font:Bold")) -> ()  [unwired: 1 in, 2 out]
      }
      event #5 {
        n208 = event-data() -> ("CtlRef"=w924:refnum<vi>)  [unwired: 6 out]
        n209 = control-ref of="Trap Delta (MHz)"() -> (w923:refnum<vi>)
        n210 = Equal?(x=w923, y=w924) -> (x = y?=w922:bool)
        n211 = case shown="False" "Oscillate Set 1" {
          tunnel: w927 -> [w947 _]
          tunnel: [w946 w950] -> w926
          tunnel: w925 -> [w945 w950]
          tunnel: w922 -> [w930 _]
          frame #0 {
            n212 = local read "BD 1 Frequency 2 (MHz)"() -> (w934:dbl)
            n213 = local read "BD 1 Frequency 1 (MHz)"() -> (w932:dbl)
            n214 = Subtract(x=w934, y="Trap Delta (MHz)") -> (x-y=w931:dbl)
            n215 = Select(t=w931, s=w930, f=w932) -> (s? t:f=w929:dbl)
            n216 = local read "Y RF Frequency Limits (MHz)"() -> (w935:T11)
            n217 = local read "X RF Frequency Limits (MHz)"() -> (w936:T11)
            n218 = local read "BD 1 Frequency 3 (MHz)"() -> (w948:dbl)
            n219 = local write "BD 1 Frequency 1 (MHz)"(w929) -> ()
            n220 = local read "BD 2 Frequency 1 (MHz)"() -> (w939:dbl)
            n221 = local read "BD 2 Frequency 2 (MHz)"() -> (w938:dbl)
            n222 = local read "BD 2 Frequency 3 (MHz)"() -> (w949:dbl)
            n223 = call "set RF board frequency - interlace.vi"("Board 2 Frequency Limits"=w935, "Board 1 Frequency Limits"=w936, "error in"=w945, "FPGA VI Reference In"=w947, "Board 2 Frequency 3 (MHz)"=w949, "Board 1 Frequency 3 (MHz)"=w948, "Board 2 Frequency 2 (MHz)"=w938, "Board 2 Frequency 1 (MHz)"=w939, "Board 1 Frequency 2 (MHz)"=w934, "Board 1 Frequency 1  (MHz)"=w929) -> ("error out"=w946:errorcluster)  [unwired: 1 out]
            n224 = Subtract(x=w939, y=w938) -> (x-y=w943:dbl)
            n225 = Subtract(x=w929, y=w934) -> (x-y=w944:dbl)
            n226 = Square(x=w943) -> (x^2=w941:dbl)
            n227 = Square(x=w944) -> (x^2=w942:dbl)
            n228 = Add(x=w942, y=w941) -> (x+y=w940:dbl)
            n229 = Square Root(x=w940) -> (sqrt(x)=w937:dbl)
            n230 = local write "Trap Delta (MHz)"(w937) -> ()
            n231 = property on="Initial delta (MHz)" class="DigNum (strict)"("Val(Sgnl)"=w937) -> ()  [unwired: 2 in, 2 out]
          }
          frame #1 {
          }
        }
      }
      event #6 {
        n232 = event-data() -> ()  [unwired: 7 out]
        n233 = local read "BD 1 Frequency 1 (MHz)"() -> (w953:dbl)
        n234 = Round To Nearest(number=w953) -> (nearest integer value=w952:dbl)
        n235 = property on="BD 1 Frequency 1 (MHz)" class="DigNum (strict)"("Val(Sgnl)"=w952) -> ()  [unwired: 2 in, 2 out]
      }
      event #7 {
        n236 = event-data() -> ()  [unwired: 7 out]
        n237 = local read "BD 1 Frequency 2 (MHz)"() -> (w955:dbl)
        n238 = Round To Nearest(number=w955) -> (nearest integer value=w954:dbl)
        n239 = property on="BD 1 Frequency 2 (MHz)" class="DigNum (strict)"("Val(Sgnl)"=w954) -> ()  [unwired: 2 in, 2 out]
      }
      event #8 {
        n240 = event-data() -> ()  [unwired: 7 out]
        n241 = local read "Stop All"() -> (w957:bool)
      }
      event #9 {
        n242 = event-data() -> ()  [unwired: 7 out]
        n243 = flat-sequence {
          frame #0 {
            n244 = Multiply(x="Delay to Interlace (s)", y=1000.0) -> (x*y=w960:dbl)
            n245 = Wait (ms)(milliseconds to wait=w960) -> ()  [unwired: 1 out]
          }
          frame #1 {
            n246 = property on="Green laser mode" class="RadioBtnsControl (strict)"("Val(Sgnl)"=enum32{"Laser ON", "Laser OFF", "Interlace"}."Interlace" ("Value (Signaling)")) -> ()  [unwired: 2 in, 2 out]
          }
        }
      }
      event #10 {
        w984 = i16 1 ("f")
        n247 = event-data() -> ()  [unwired: 7 out]
        n248 = local write "Trap 1 (ON/OFF)"("Trap 1 ON") -> ()
        n249 = local write "Trap 2 (ON/OFF)"("Trap 2 ON") -> ()
        n250 = Boolean To (0,1)(Boolean="Trap 3 ON") -> (0, 1=w985:i16)
        n251 = Boolean To (0,1)(Boolean="Trap 1 ON") -> (0, 1=w986:i16)
        n252 = Boolean To (0,1)(Boolean="Trap 2 ON") -> (0, 1=w987:i16)
        n253 = Select(t=w987, s="Trap ON/OFF X or Y Amp?", f=w984) -> (s? t:f=w982:i16)
        n254 = Select(t=w986, s="Trap ON/OFF X or Y Amp?", f=w984) -> (s? t:f=w983:i16)
        n255 = Select(t=w985, s="Trap ON/OFF X or Y Amp?", f=w984) -> (s? t:f=w981:i16)
        n256 = Select(t=w984, s="Trap ON/OFF X or Y Amp?", f=w987) -> (s? t:f=w979:i16)
        n257 = Select(t=w984, s="Trap ON/OFF X or Y Amp?", f=w986) -> (s? t:f=w980:i16)
        n258 = Select(t=w984, s="Trap ON/OFF X or Y Amp?", f=w985) -> (s? t:f=w978:i16)
        n259 = And(x="All FB On/Off", y="Feedback On/Off") -> (x .and. y?=w976:cluster{"Set 1":bool, "Set 2":bool})
        n260 = local read "BD 1 Amplitude 1 (%)"() -> (w996:dbl)
        n261 = local read "BD 1 Amplitude 2 (%)"() -> (w995:dbl)
        n262 = local read "BD 1 Amplitude 3 (%)"() -> (w994:dbl)
        n263 = Unbundle By Name(w976) -> ("Set 1"=w971:bool, "Set 2"=w968:bool)
        n264 = local read "Y RF Amplitude Limits (%)"() -> (w964:T11)
        n265 = local read "X RF Amplitude Limits (%)"() -> (w965:T11)
        n266 = local read "BD 2 Amplitude 1 (%)"() -> (w997:dbl)
        n267 = local read "BD 2 Amplitude 2 (%)"() -> (w998:dbl)
        n268 = local read "BD 2 Amplitude 3 (%)"() -> (w999:dbl)
        n269 = And(x="Trap 2 ON", y=w968) -> (x .and. y?=w966:bool)
        n270 = And(x="Trap 1 ON", y=w971) -> (x .and. y?=w969:bool)
        n271 = Multiply(x=w983, y=w996) -> (x*y=w991:dbl)
        n272 = Multiply(x=w995, y=w982) -> (x*y=w989:dbl)
        n273 = Multiply(x=w994, y=w981) -> (x*y=w990:dbl)
        n274 = Multiply(x=w997, y=w980) -> (x*y=w1000:dbl)
        n275 = Multiply(x=w998, y=w979) -> (x*y=w1001:dbl)
        n276 = Multiply(x=w999, y=w978) -> (x*y=w1002:dbl)
        n277 = call "set RF board amplitude - interlace.vi"("Board 2 Amplitude Limits"=w964, "Board 1 Amplitude Limits"=w965, "error in"=w992, "FPGA VI Reference In"=w993, "Board 2 Amplitude 3 (%)"=w1002, "Board 1 Amplitude 3 (%)"=w990, "Board 2 Amplitude 2 (%)"=w1001, "Board 2 Amplitude 1 (%)"=w1000, "Board 1 Amplitude 2 (%)"=w989, "Board 1 Amplitude 1 (%)"=w991) -> ("error out"=w973:errorcluster, "FPGA VI Reference Out"=w974:T14)
        n278 = xnode "Read/Write Control"("FPGA VI Reference In"=w974, "error in"=w973, "FB On/Off Set 1"=w969, "FB On/Off Set 2"=w966) -> ("error out"=w972:errorcluster)  [unwired: 1 out]
      }
      event #11 {
        n279 = event-data() -> ()  [unwired: 7 out]
        n280 = property on="Saved AOD Raster Scan Parameter Sets" class="Arr (strict)"() -> ("Index Values"=w1069:u32[])  [unwired: 2 in, 2 out]
        n281 = Index Array(array=w1069, index=0) -> (element=w1066:u32)
        n282 = Index Array(array="Saved AOD Raster Scan Parameter Sets", index=w1066) -> (element=w1065:T22)
        n283 = Unbundle By Name(w1065) -> ("Scan Range AOD (nm) 2"=w1064:dbl, "Step Size AOD (nm) 2"=w1063:dbl, "Scan Speed AOD (nm/s) 2"=w1062:dbl, "Number of scans (AOD) 2"=w1061:u16)
        n284 = flat-sequence {
          tunnel: w1064 -> [w1073]
          tunnel: w1063 -> [w1072]
          tunnel: w1062 -> [w1071]
          tunnel: w1061 -> [w1074]
          frame #0 {
            n285 = local write "Scan Speed (nm/s)"(w1071) -> ()
            n286 = local write "Scan Range (nm)"(w1073) -> ()
            n287 = local write "Step Size (nm)"(w1072) -> ()
          }
          frame #1 {
            n288 = property on="Number of F/B Scans (AOD)" class="DigNum (strict)"("Val(Sgnl)"=w1074) -> ()  [unwired: 2 in, 2 out]
          }
        }
      }
      event #12 {
        n289 = event-data() -> ()  [unwired: 7 out]
        n290 = property on="Trap 2 ON" class="Bool (strict)"("Val(Sgnl)"="Trap 2 (ON/OFF)") -> ()  [unwired: 2 in, 2 out]
        n291 = property on="Trap 1 ON" class="Bool (strict)"("Val(Sgnl)"="Trap 1 (ON/OFF)") -> ()  [unwired: 2 in, 2 out]
      }
      event #13 {
        n292 = event-data() -> ()  [unwired: 7 out]
        n293 = local read "DIO count 3 (ticks)"() -> (w1087:u32)
        n294 = local read "DIO count 1 (ticks)"() -> (w1089:u32)
        n295 = local read "DIO count 2 (ticks)"() -> (w1088:u32)
        n296 = To Unsigned Byte Integer(number="Not-Interlacing Set") -> (unsigned 8bit integer=w1078:u8)
        n297 = Add(x=w1078, y=u8 1) -> (x+y=w1082:u8)
        n298 = xnode "Read/Write Control"("FPGA VI Reference In"=w1093, "error in"=w1091, "DIO count 1 (ticks)"=w1089, "DIO count 2 (ticks)"=w1088, "DIO count 3 (ticks)"=w1087, "Interlace ON/OFF"="Interlace", "Number Interlace Cycles"="Number Interlace Sets", "Interlace Off Parameters"=w1082) -> ("error out"=w1092:errorcluster)  [unwired: 1 out]
        n299 = Build Array(w1089, w1088, w1087) -> (w1080:u32[])
        n300 = Split 1D Array(array=w1080, index="Number Interlace Sets") -> (first subarray=w1090:u32[])  [unwired: 1 out]
        n301 = Index Array(array=w1080, index=w1078) -> (element=w1079:u32)
        n302 = Add Array Elements(numeric array=w1090) -> (sum=w1084:u32)
        n303 = Select(t=w1084, s="Interlace", f=w1079) -> (s? t:f=→"Total Counts (ticks)":u32)
      }
      event #14 {
        n304 = event-data() -> ()  [unwired: 7 out]
        n305 = Unbundle By Name("Reset Feedback") -> ("Set 1"=w1229:bool, "Set 2"=w1228:bool)
        n306 = xnode "Read/Write Control"("FPGA VI Reference In"=w1231, "error in"=w1226, "FB Reset Set 1"=w1229, "FB Reset Set 2"=w1228) -> ("error out"=w1227:errorcluster)  [unwired: 1 out]
      }
      event #15 {
        n307 = event-data() -> ()  [unwired: 7 out]
        n308 = Unbundle By Name("PID Gains") -> ("Set 1"=w1292:T9, "Set 2"=w1291:T9)
        n309 = xnode "Read/Write Control"("FPGA VI Reference In"=w1293, "error in"=w1289, "FB Gains Set 1"=w1292, "FB Gains Set 2"=w1291) -> ("error out"=w1290:errorcluster)  [unwired: 1 out]
      }
      event #16 {
        n310 = event-data() -> ()  [unwired: 7 out]
        n311 = xnode "Read/Write Control"("FPGA VI Reference In"=w1336, "error in"=w1332) -> ("FPGA VI Reference Out"=w1335:T14, "error out"=w1334:errorcluster, "AI2 Y Sum Set 1"=w1343:i16, "AI2 Y Sum Set 2"=w1342:i16)
        n312 = Cluster To Array(cluster="AI2 to Setpoint") -> (array=w1346:bool[])
        n313 = local read "AI2 (V)"() -> (w1344:cluster{"Set 1":dbl, "Set 2":dbl})
        n314 = Or Array Elements(Boolean array=w1346) -> (logical OR=w1347:bool)
        n315 = Bundle By Name(cluster=w1344, "Set 1"=w1343, "Set 2"=w1342) -> (w1341:cluster{"Set 1":dbl, "Set 2":dbl})
        n316 = Divide(x=w1341, y=3276.7) -> (x/y=w1340:cluster{"Set 1":dbl, "Set 2":dbl})
        "AI2 (V)" <- w1340
        n317 = case shown="True" w1347 {
          tunnel: [w1409 w1426] -> w1339
          tunnel: "AI2 to Setpoint" -> [_ w1422]
          tunnel: "Setpoints (V)" -> [w1410 w1425]
          tunnel: w1340 -> [_ w1419]
          frame #0 {
            n318 = Multiply(x=3276.7, y=w1410) -> (x*y=w1411:cluster{"Set 1":dbl, "Set 2":dbl})
            n319 = To Word Integer(number=w1411) -> (16bit integer=w1409:cluster{"Set 1":i16, "Set 2":i16})
          }
          frame #1 {
            n320 = Unbundle By Name(w1419) -> ("Set 1"=w1418:dbl, "Set 2"=w1417:dbl)
            n321 = Unbundle By Name(w1425) -> ("Set 1"=w1424:dbl, "Set 2"=w1423:dbl)
            n322 = Unbundle By Name(w1422) -> ("Set 1"=w1421:bool, "Set 2"=w1420:bool)
            n323 = Select(t=w1418, s=w1421, f=w1424) -> (s? t:f=w1416:dbl)
            n324 = Select(t=w1417, s=w1420, f=w1423) -> (s? t:f=w1415:dbl)
            n325 = Bundle By Name(cluster=w1425, "Set 1"=w1416, "Set 2"=w1415) -> (w1413:cluster{"Set 1":dbl, "Set 2":dbl})
            n326 = Multiply(x=3276.7, y=w1413) -> (x*y=w1414:cluster{"Set 1":dbl, "Set 2":dbl})
            n327 = local write "Setpoints (V)"(w1413) -> ()
            n328 = To Word Integer(number=w1414) -> (16bit integer=w1426:cluster{"Set 1":i16, "Set 2":i16})
          }
        }
        n329 = Unbundle By Name(w1339) -> ("Set 1"=w1338:i16, "Set 2"=w1337:i16)
        n330 = xnode "Read/Write Control"("FPGA VI Reference In"=w1335, "error in"=w1334, "FB Setpoint Set 1"=w1338, "FB Setpoint Set 2"=w1337) -> ("error out"=w1333:errorcluster)  [unwired: 1 out]
      }
      event #17 {
        n331 = event-data() -> ()  [unwired: 7 out]
        n332 = xnode "Read/Write Control"("FPGA VI Reference In"=w1486, "error in"=w1484, "Invert GI"="Invert GI", "Invert GI 2"="Invert GI") -> ("error out"=w1485:errorcluster)  [unwired: 1 out]
      }
      event #18 {
        n333 = event-data() -> ()  [unwired: 7 out]
        n334 = local read "Green FB Setpoint (mV)"() -> (w1550:dbl)
        n335 = local read "Current When FB OFF (%)"() -> (w1553:dbl)
        n336 = Multiply(x=w1550, y=3.2767) -> (x*y=w1549:dbl)
        n337 = Multiply(x=w1553, y=655.35) -> (x*y=w1554:dbl)
        n338 = To Unsigned Word Integer(number=w1554) -> (unsigned 16bit integer=w1552:u16)
        n339 = local read "Green int current ON count adj"() -> (w1557:u32)
        n340 = local read "Green FB Gains"() -> (w1556:T9)
        n341 = local read "Green Laser ON/Interlacing"() -> (w1547:bool)
        n342 = local read "Green laser mode"() -> (w1546:enum32{"Laser ON", "Laser OFF", "Interlace"})
        n343 = local read "Green FB On/Off"() -> (w1558:bool)
        n344 = Equal?(x=w1546, y=enum32{"Laser ON", "Laser OFF", "Interlace"}."Interlace") -> (x = y?=w1544:bool)
        n345 = Compound Arithmetic op=AND(w1544, w1558, w1547) -> (w1548:bool)
        n346 = xnode "Read/Write Control"("FPGA VI Reference In"=w1561, "error in"=w1560, "Green FB Setpoint"=w1549, "Green FB On/Off"=w1548, "Current Out"=w1552, "Green int current ON count adj"=w1557, "Green FB Gains"=w1556) -> ("error out"=w1559:errorcluster)  [unwired: 1 out]
      }
      event #19 {
        n347 = event-data() -> ()  [unwired: 7 out]
        n348 = case shown="True" "Green Laser ON/Interlacing" {
          tunnel: "Green laser mode" -> [_ w1679]
          tunnel: [enum32{"Laser ON", "Laser OFF", "Interlace"}."Laser OFF" ("Green laser mode") w1679] -> w1667
          tunnel: [FALSE w1675] -> w1666
          frame #0 {
          }
          frame #1 {
            n349 = local read "Green FB On/Off"() -> (w1676:bool)
            n350 = Equal?(x=w1679, y=enum32{"Laser ON", "Laser OFF", "Interlace"}."Interlace") -> (x = y?=w1677:bool)
            n351 = And(x=w1677, y=w1676) -> (x .and. y?=w1675:bool)
          }
        }
        n352 = xnode "Read/Write Control"("FPGA VI Reference In"=w1672, "error in"=w1670, "Operating Mode"=w1667, "Operating Mode 2"=w1667, "Green FB On/Off"=w1666) -> ("error out"=w1671:errorcluster)  [unwired: 1 out]
      }
      event #20 {
        n353 = event-data() -> ()  [unwired: 7 out]
        n354 = local read "Phase Adj. (APD Gate)"() -> (w1755:i16)
        n355 = Negate(x=w1755) -> (-x=w1763:i16)
        n356 = Select(t=w1763, s="- phase (APD Gate)", f=w1755) -> (s? t:f=w1762:i16)
        n357 = Or(x="- phase (APD Gate)", y="+ phase (APD Gate)") -> (x .or. y?=w1758:bool)
        n358 = xnode "Read/Write Control"("FPGA VI Reference In"=w1765, "error in"=w1764, "Phase count adjustment (APD Gate)"=w1762) -> ("FPGA VI Reference Out"=w1760:T14, "error out"=w1761:errorcluster)
        n359 = xnode "Read/Write Control"("FPGA VI Reference In"=w1760, "error in"=w1761, "+ phase (APD Gate)"=w1758) -> ("error out"=w1759:errorcluster)  [unwired: 1 out]
      }
      event #21 {
        n360 = event-data() -> ()  [unwired: 7 out]
        n361 = local read "Phase Adj. (APD Acq)"() -> (w1841:i16)
        n362 = Negate(x=w1841) -> (-x=w1847:i16)
        n363 = Select(t=w1847, s="+ phase (APD Acq)", f=w1841) -> (s? t:f=w1846:i16)
        n364 = Or(x="+ phase (APD Acq)", y="- phase (APD Acq)") -> (x .or. y?=w1842:bool)
        n365 = xnode "Read/Write Control"("FPGA VI Reference In"=w1849, "error in"=w1848, "Phase Count Adjustment (APD Acq)"=w1846) -> ("FPGA VI Reference Out"=w1844:T14, "error out"=w1845:errorcluster)
        n366 = xnode "Read/Write Control"("FPGA VI Reference In"=w1844, "error in"=w1845, "+ phase (APD Acq)"=w1842) -> ("error out"=w1843:errorcluster)  [unwired: 1 out]
      }
      event #22 {
        n367 = event-data() -> ()  [unwired: 7 out]
        n368 = Negate(x="Phase adj. (GI)") -> (-x=w1931:i16)
        n369 = Select(t=w1931, s="+ phase (GI)", f="Phase adj. (GI)") -> (s? t:f=w1930:i16)
        n370 = Or(x="+ phase (GI)", y="- phase (GI)") -> (x .or. y?=w1926:bool)
        n371 = xnode "Read/Write Control"("FPGA VI Reference In"=w1933, "error in"=w1932, "Phase count adjustment (GI)"=w1930) -> ("FPGA VI Reference Out"=w1928:T14, "error out"=w1929:errorcluster)
        n372 = xnode "Read/Write Control"("FPGA VI Reference In"=w1928, "error in"=w1929, "+ phase (GI)"=w1926) -> ("error out"=w1927:errorcluster)  [unwired: 1 out]
      }
      event #23 {
        n373 = event-data() -> ()  [unwired: 7 out]
        n374 = Negate(x="Phase adj. (GI) 2") -> (-x=w2015:i16)
        n375 = Select(t=w2015, s="+ phase (GI) 2", f="Phase adj. (GI) 2") -> (s? t:f=w2014:i16)
        n376 = Or(x="+ phase (GI) 2", y="- phase (GI) 2") -> (x .or. y?=w2010:bool)
        n377 = xnode "Read/Write Control"("FPGA VI Reference In"=w2017, "error in"=w2016, "Phase count adjustment (GI) 2"=w2014) -> ("FPGA VI Reference Out"=w2012:T14, "error out"=w2013:errorcluster)
        n378 = xnode "Read/Write Control"("FPGA VI Reference In"=w2012, "error in"=w2013, "+ phase (GI) 2"=w2010) -> ("error out"=w2011:errorcluster)  [unwired: 1 out]
      }
      event #24 {
        n379 = event-data() -> ()  [unwired: 7 out]
        n380 = Negate(x="Phase adj. (Green FB)") -> (-x=w2099:i16)
        n381 = Select(t=w2099, s="+ phase (Green FB)", f="Phase adj. (Green FB)") -> (s? t:f=w2098:i16)
        n382 = Or(x="+ phase (Green FB)", y="- phase (Green FB)") -> (x .or. y?=w2094:bool)
        n383 = xnode "Read/Write Control"("FPGA VI Reference In"=w2101, "error in"=w2100, "Phase count adjustment (Green FB)"=w2098) -> ("FPGA VI Reference Out"=w2096:T14, "error out"=w2097:errorcluster)
        n384 = xnode "Read/Write Control"("FPGA VI Reference In"=w2096, "error in"=w2097, "+ phase (Green FB)"=w2094) -> ("error out"=w2095:errorcluster)  [unwired: 1 out]
      }
      event #25 {
        n385 = event-data() -> ()  [unwired: 7 out]
        n386 = local read "APD Integration Time (s)"() -> (w2175:dbl)
        n387 = local read "APD Gate ON Count"() -> (w2190:u32)
        n388 = local read "APD Gate OFF Count"() -> (w2189:u32)
        n389 = local read "Invert APD Gate"() -> (w2191:bool)
        n390 = local read "APD Gate"() -> (w2188:enum32{"ON", "OFF", "Interlace"})
        n391 = Multiply(x=w2175, y=40000000.0) -> (x*y=w2186:dbl)
        n392 = Reciprocal(x=w2175) -> (1/x=→"APD Acq Rate (Hz)":dbl)
        n393 = To Unsigned Long Integer(number=w2186) -> (unsigned 32bit integer=w2185:u32)
        n394 = local read "DMA Update Period (s)"() -> (w2176:dbl)
        n395 = Divide(x=w2176, y=w2175) -> (x/y=w2179:dbl)
        n396 = local read "APD 1 AO offset"() -> (w2181:i16)
        n397 = local read "APD 1 AO Mult."() -> (w2183:i16)
        n398 = local read "APD 2 AO Mult."() -> (w2182:i16)
        n399 = local read "APD 2 AO offset"() -> (w2180:i16)
        n400 = Multiply(x=2.0, y=w2179) -> (x*y=w2178:dbl)
        n401 = local write "APD Samples/FIFO Acq."(w2179) -> ()
        n402 = local write "APD Elements/DMA read"(w2178) -> ()
        n403 = xnode "Read/Write Control"("FPGA VI Reference In"=w2194, "error in"=w2193, "Invert APD Gate"=w2191, "APD Gate ON Count"=w2190, "APD Gate OFF Count"=w2189, "APD Acq Rate Count"=w2185, "APD Gate Operating Mode"=w2188, "APD 1 AO scale factor"=w2183, "APD 2 AO scale factor"=w2182, "APD 1 AO offset"=w2181, "APD 2 AO offset"=w2180) -> ("error out"=w2192:errorcluster)  [unwired: 1 out]
      }
      event #26 {
        n404 = event-data() -> ()  [unwired: 7 out]
        n405 = xnode "Read/Write Control"("FPGA VI Reference In"=w2389, "error in"=w2387, "Green interlace ON count"="GI Frequency, ON count", "Green interlace OFF count"="GI Frequency, OFF count", "Green interlace ON count 2"="GI Frequency, ON count", "Green interlace OFF count 2"="GI Frequency, OFF count", "Green FB Count"="Green FB Count") -> ("error out"=w2388:errorcluster)  [unwired: 1 out]
      }
      event #27 {
        w2557 = 123.0  # AOM cal (nm/MHz)
        n406 = event-data() -> ()  [unwired: 7 out]
        n407 = local read "BD 1 Frequency 1 (MHz)"() -> (w2540:dbl)
        n408 = local read "AOM X Cal (nm/MHz)"() -> (w2532:dbl)
        n409 = local read "X RF Frequency Limits (MHz)"() -> (w2544:T11)
        n410 = local read "Y RF Frequency Limits (MHz)"() -> (w2541:T11)
        n411 = local read "BD 2 Frequency 1 (MHz)"() -> (w2546:dbl)
        n412 = Negate(x="Scan Range (nm)") -> (-x=w2509:dbl)
        n413 = Divide(x=w2509, y=w2532) -> (x/y=w2513:dbl)
        n414 = Select(t=w2544, s="Scan BD", f=w2541) -> (s? t:f=w2543:T11)
        n415 = Select(t=w2540, s="Scan BD", f=w2546) -> (s? t:f=w2545:dbl)
        n416 = Unbundle By Name(w2543) -> ("Maximum"=w2552:dbl, "Minimum"=w2551:dbl)
        n417 = Add(x=w2513, y=w2545) -> (x+y=w2549:dbl)
        n418 = Divide(x=w2509, y="Step Size (nm)") -> (x/y=w2529:dbl)
        n419 = Divide(x="Step Size (nm)", y=w2532) -> (x/y=w2538:dbl)
        n420 = Absolute Value(x=w2529) -> (abs(x)=w2512:dbl)
        n421 = Sign(1:w2509) -> (0:w2510:dbl)
        n422 = In Range and Coerce(upper limit=w2552, x=w2549, lower limit=w2551) -> (coerced(x)=w2548:dbl, In Range?=w2550:bool)
        n423 = To Unsigned Quad Integer(1:w2512) -> (0:w2528:u64)
        "Scan steps (AOD)" <- w2528
        n424 = call "IR AOM freq to word.vi"("Frequency In (MHz)"=w2538) -> ("Frequency Word Out (double)"=w2535:dbl)
        n425 = Multiply(x=w2510, y=w2535) -> (x*y=w2511:dbl)
        n426 = Subtract(x=w2549, y=w2548) -> (x-y=w2547:dbl)
        n427 = To Quad Integer(1:w2511) -> (0:w2534:i64)
        "Incr. int (AOD)" <- w2534
        n428 = Subtract(x=w2513, y=w2547) -> (x-y=w2533:dbl)
        "Scan Range (MHz)" <- w2533
        n429 = Select(t=w2513, s=w2550, f=w2533) -> (s? t:f=w2553:dbl)
        n430 = Multiply(x=w2533, y=w2532) -> (x*y=w2531:dbl)
        n431 = Decrement(x=w2528) -> (x-1=w2581:u64)
        n432 = Negate(x=w2531) -> (-x=w2527:dbl)
        n433 = local write "Scan Range (nm)"(w2527) -> ()
        n434 = Divide(x=w2553, y=w2581) -> (x/y=w2537:dbl)
        "Scan Increment (MHz)" <- w2537
        n435 = call "IR AOM freq to word.vi"("Frequency In (MHz)"=w2537) -> ("Frequency Word Out (double)"=w2536:dbl)
        n436 = Divide(x="Step Size (nm)", y="Scan Speed (nm/s)") -> (x/y=w2524:dbl)
        n437 = To Quad Integer(1:w2536) -> ()  [unwired: 1 out]
        n438 = local read "Number Interlace Sets"() -> (w2507:u8)
        n439 = local read "AI Count (ticks)"() -> (w2508:u32)
        n440 = local read "Total Counts (ticks)"() -> (w2506:u32)
        n441 = local read "# Samples/trap"() -> (w2539:dbl)
        n442 = Multiply(x=w2508, y=w2507) -> (x*y=w2505:u32)
        n443 = Divide(x=w2506, y=w2505) -> (x/y=w2504:dbl)
        n444 = Select(t=w2540, s="Scan BD", f=w2546) -> (s? t:f=w2578:dbl)
        "Initial freq. (MHz)" <- w2578
        n445 = Add(x=w2553, y=w2578) -> (x+y=→"Final freq. (MHz)":dbl)
        n446 = Divide(x=w2506, y=40000000.0) -> (x/y=w2523:dbl)
        n447 = Divide(x=w2524, y=w2523) -> (x/y=w2522:dbl)
        n448 = To Unsigned Quad Integer(1:w2522) -> (0:w2521:u64)
        "Cycles/step (AOD)" <- w2521
        n449 = xnode "Read/Write Control"("FPGA VI Reference In"=w2589, "error in"=w2588, "Scan steps"=w2528, "Number of scans"="Number of F/B Scans (AOD)", "Cycles per step"=w2521, "Scan freq.  increment"=w2534, "Scan BD"="Scan BD") -> ("error out"=w2587:errorcluster)  [unwired: 1 out]
        n450 = Multiply(x=w2528, y=w2521) -> (x*y=w2582:u64)
        n451 = Multiply(x=w2582, y=u64 2) -> (x*y=w2503:u64)
        n452 = Multiply(x=w2504, y=w2503) -> (x*y=w2502:dbl)
        "Data points/scan (f/b)" <- w2502
        n453 = Multiply(x=w2502, y="Number of F/B Scans (AOD)") -> (x*y=w2585:dbl)
        "Data points/scans" <- w2585
        n454 = Divide(x=w2585, y=w2539) -> (x/y=→"N sets should be saved":dbl)
        n455 = Multiply(x=w2582, y=w2523) -> (x*y=w2520:dbl)
        "Time/Scan (s) (AOD)" <- w2520
        n456 = Select(t=w2553, s="Scan BD", f=0.0) -> (s? t:f=w2579:dbl)
        n457 = Select(t=0.0, s="Scan BD", f=w2553) -> (s? t:f=w2575:dbl)
        n458 = local read "BD 2 Frequency 2 (MHz)"() -> (w2571:dbl)
        n459 = local read "BD 1 Frequency 2 (MHz)"() -> (w2574:dbl)
        n460 = Add(x=w2575, y=w2546) -> (x+y=w2572:dbl)
        n461 = Add(x=w2540, y=w2579) -> (x+y=w2573:dbl)
        n462 = Multiply(x=w2520, y=2.0) -> (x*y=w2519:dbl)
        n463 = Multiply(x=w2519, y="Number of F/B Scans (AOD)") -> (x*y=w2516:dbl)
        n464 = Divide(x=w2516, y=60.0) -> (x/y=→"Time to Finish All (min)":dbl)
        n465 = Add(x="Trap 2 Bead Size (nm)", y="Trap 1 Bead Size (nm)") -> (x+y=w2561:dbl)
        n466 = Divide(x=w2561, y=2.0) -> (x/y=w2555:dbl)
        n467 = Subtract(x=w2572, y=w2571) -> (x-y=w2569:dbl)
        n468 = Subtract(x=w2573, y=w2574) -> (x-y=w2570:dbl)
        n469 = local read "Initial delta (MHz)"() -> (w2558:dbl)
        n470 = Square(x=w2569) -> (x^2=w2568:dbl)
        n471 = Square(x=w2570) -> (x^2=w2567:dbl)
        n472 = Add(x=w2567, y=w2568) -> (x+y=w2566:dbl)
        n473 = Square Root(x=w2566) -> (sqrt(x)=w2565:dbl)
        "Final delta (MHz)" <- w2565
        n474 = Multiply(x=w2557, y=w2565) -> (x*y=w2564:dbl)
        n475 = Multiply(x=w2558, y=w2557) -> (x*y=w2556:dbl)
        n476 = Subtract(x=w2556, y=w2555) -> (x-y=→"Initial sep (nm)":dbl)
        n477 = Subtract(x=w2564, y=w2555) -> (x-y=→"Final sep (nm)":dbl)
      }
      event #28 {
        n478 = event-data() -> ()  [unwired: 7 out]
        n479 = local read "Freq or Amp switch first"() -> (w2676:bool)
        n480 = local read "Amp switch delay"() -> (w2677:u16)
        n481 = local read "Freq switch delay"() -> (w2679:u16)
        n482 = local read "Swap F1 and F2"() -> (w2678:bool)
        n483 = xnode "Read/Write Control"("FPGA VI Reference In"=w2682, "error in"=w2681, "Freq switch delay"=w2679, "Swap F1 and F2"=w2678, "Amp switch delay"=w2677, "Freq or Amp switch first"=w2676) -> ("error out"=w2680:errorcluster)  [unwired: 1 out]
      }
      event #29 {
        w2779 = 32767.0 ("y")
        n484 = event-data() -> ()  [unwired: 7 out]
        n485 = Select(t="Scan lines (y)", s="2D or 1D Scan", f="Number of scans (MCL)") -> (s? t:f=w2784:u64)
        n486 = Decrement(x="Scan steps (MCL)") -> (x-1=w2800:u64)
        n487 = Divide(x="Scan Range (V)\n(of steps)", y=w2800) -> (x/y=w2799:dbl)
        "Desired Scan Incr (V)" <- w2799
        n488 = local read "APD Integration Time (s)"() -> (w2792:dbl)
        n489 = Multiply(x=w2799, y=w2779) -> (x*y=w2808:dbl)
        n490 = Divide(x=w2808, y=10.0) -> (x/y=w2798:dbl)
        "Desired incr (int)" <- w2798
        n491 = local read "Update Count (MCL)"() -> (w2804:u32)
        n492 = Round Toward -Infinity(1:w2798) -> (0:w2807:dbl)
        n493 = To Word Integer(number=w2807) -> (16bit integer=w2782:i16)
        "Actual Incr. int (MCL)" <- w2782
        n494 = Multiply(x=w2792, y=40000000.0) -> (x*y=w2805:dbl)
        n495 = Divide(x=w2805, y=w2804) -> (x/y=w2803:dbl)
        n496 = Multiply(x=i16 10, y=w2782) -> (x*y=w2780:i16)
        n497 = Multiply(x="N APD Samp/step", y=w2803) -> (x*y=w2802:dbl)
        "Cycles/step (MCL)" <- w2802
        n498 = Divide(x=w2780, y=w2779) -> (x/y=→"Actual MCL Inc (V)":dbl)
        n499 = Multiply(x="N APD Samp/step", y="Scan steps (MCL)") -> (x*y=w2794:dbl)
        n500 = local read "APD Samples/FIFO Acq."() -> (w2791:dbl)
        n501 = Multiply(x=w2794, y=u64 2) -> (x*y=w2793:dbl)
        "Data points/scan (f+b)" <- w2793
        n502 = Multiply(x=w2793, y=w2784) -> (x*y=w2811:dbl)
        "Data points/scans (MCL)" <- w2811
        n503 = Multiply(x=w2792, y=w2793) -> (x*y=w2785:dbl)
        "Time/f+b scan (s) (MCL)" <- w2785
        n504 = Divide(x=w2811, y=w2791) -> (x/y=→"N sets should be saved (MCL)":dbl)
        n505 = Multiply(x=w2785, y=w2784) -> (x*y=→"Total Time (s)":dbl)
        n506 = Not(x="Fast Scan Dir") -> (.not. x?=w2789:bool)
        n507 = xnode "Read/Write Control"("FPGA VI Reference In"=w2815, "error in"=w2814, "Scan steps (MCL)"="Scan steps (MCL)", "Number of scans (MCL)"=w2784, "Cycles per step (MCL)"=w2802, "Scan freq.  increment (MCL)"=w2782, "1D or 2D Scan?"="2D or 1D Scan", "MCL Scan Axis"=w2789, "Cont. Scan (MCL)"="Continuous MCL Scanning") -> ("error out"=w2813:errorcluster)  [unwired: 1 out]
      }
      event #30 {
        w2952 = 1000.0 ("y")
        n508 = event-data() -> ()  [unwired: 7 out]
        n509 = local read "Save file name"() -> (w2977:path)
        n510 = local write "Read Cal"(FALSE ("Read Cal")) -> ()
        n511 = Strip Path(path=w2977) -> (stripped path=w2976:path)  [unwired: 1 out]
        n512 = Path To String(path=w2976) -> (string=w2975:string)
        n513 = Concatenate Strings(w2975, "\\current.cal" ("string")) -> (w2973:string)
        n514 = String To Path(string=w2973) -> (path=w2972:path)
        n515 = Open/Create/Replace File(file path (use dialog)=w2972, operation (0:open)=T21."open", access (0:read/write)=enum16{"read/write", "read-only", "write-only"}."read-only") -> (refnum out=w2980:refnum<file>, error out=w2966:errorcluster)  [unwired: 1 in, 3 out]
        n516 = Deny Access(4:w2966, 7:w2980) -> (0:w2965:errorcluster, 3:w2971:refnum<file>)  [unwired: 1 out]
        n517 = Read from Binary File(5:0.0, 8:w2965, 9:T20."big-endian, network order" ("byte order (0:big-endian, network order)"), 10:-1 ("count (1)"), 11:w2971) -> (0:w2964:errorcluster, 2:w2962:dbl[], 3:w2967:refnum<file>)  [unwired: 2 out]
        n518 = Array To Cluster(array=w2962) -> (cluster=w2961:T23)
        n519 = Unbundle(w2961) -> ("[0]"=w2960:dbl, "[1]"=w2959:dbl, "[2]"=w2958:dbl, "[3]"=w2957:dbl, "[4]"=w2956:dbl, "[5]"=w2955:dbl)
        n520 = Close File(refnum=w2967, error in=w2964) -> (error out=→"Read cal error":errorcluster)  [unwired: 1 out]
        n521 = Multiply(x=w2955, y=w2952) -> (x*y=w2953:dbl)
        n522 = local write "T2 kappa_x (pN/nm)"(w2957) -> ()
        n523 = local write "T1 kappa_x (pN/nm)"(w2958) -> ()
        n524 = local write "T1 alpha_x (nm/V)"(w2960) -> ()
        n525 = local write "T2 alpha_x (nm/V)"(w2959) -> ()
        n526 = Multiply(x=w2956, y=w2952) -> (x*y=w2954:dbl)
        n527 = local write "T1 offset_x (mV)"(w2954) -> ()
        n528 = local write "T2 offset_x (mV)"(w2953) -> ()
      }
      event #31 {
        n529 = event-data() -> ()  [unwired: 7 out]
        n530 = local write "MCL Scanning"(FALSE ("MCL Scanning")) -> ()
        n531 = xnode "Read/Write Control"("FPGA VI Reference In"=w2985, "error in"=w2984, "Abort scan (MCL)"="Abort MCL Scan") -> ("error out"=w2983:errorcluster)  [unwired: 1 out]
      }
      event #32 {
        n532 = event-data() -> ()  [unwired: 7 out]
        n533 = xnode "Read/Write Control"("FPGA VI Reference In"=w3026, "error in"=w3025, "MCL count"="Update Count (MCL)") -> ("error out"=w3024:errorcluster)  [unwired: 1 out]
      }
      event #33 {
        n534 = event-data() -> ()  [unwired: 7 out]
        n535 = Negate(x="Phase adjust (MCL)") -> (-x=w3071:i16)
        n536 = Select(t=w3071, s="- phase (MCL)", f="Phase adjust (MCL)") -> (s? t:f=w3069:i16)
        n537 = Or(x="- phase (MCL)", y="+ phase (MCL)") -> (x .or. y?=w3064:bool)
        n538 = xnode "Read/Write Control"("FPGA VI Reference In"=w3073, "error in"=w3072, "Phase count adjustment (MCL)"=w3069) -> ("FPGA VI Reference Out"=w3065:T14, "error out"=w3066:errorcluster)
        n539 = xnode "Read/Write Control"("FPGA VI Reference In"=w3065, "error in"=w3066, "+ phase (MCL)"=w3064) -> ("error out"=w3063:errorcluster)  [unwired: 1 out]
      }
      event #34 {
        n540 = event-data() -> ()  [unwired: 7 out]
        n541 = xnode "Read/Write Control"("FPGA VI Reference In"=w3150, "error in"=w3149, "Abort scan"="Abort AOD Scan") -> ("error out"=w3148:errorcluster)  [unwired: 1 out]
      }
      event #35 {
        n542 = event-data() -> ()  [unwired: 7 out]
        n543 = xnode "Read/Write Control"("FPGA VI Reference In"=w3191, "error in"=w3190, "Cont. Scan"="Continuous AOD Scanning") -> ("error out"=w3189:errorcluster)  [unwired: 1 out]
      }
      event #36 {
        n544 = event-data() -> ()  [unwired: 7 out]
        n545 = call "Create new save file.vi"("Insert"="", "Ext"=".dat" ("string"), "Index In"="Index") -> ("Path Out"=→"Save file name":path, "Index Out"=w3229:dbl)
        "Save index" <- w3229
        n546 = local write "Index"(w3229) -> ()
      }
      event #37 {
        w3244 = 10.0 ("y")
        w3243 = 32767.0 ("y")
        n547 = event-data() -> ()  [unwired: 7 out]
        n548 = local read "AO2"() -> (w3242:dbl)
        n549 = local read "AO1"() -> (w3239:dbl)
        n550 = Multiply(x=w3239, y=w3243) -> (x*y=w3238:dbl)
        n551 = Multiply(x=w3242, y=w3243) -> (x*y=w3241:dbl)
        n552 = Divide(x=w3238, y=w3244) -> (x/y=w3237:dbl)
        n553 = Divide(x=w3241, y=w3244) -> (x/y=w3240:dbl)
        n554 = To Word Integer(number=w3237) -> (16bit integer=w3245:i16)
        n555 = To Word Integer(number=w3240) -> (16bit integer=w3246:i16)
        n556 = xnode "Read/Write Control"("FPGA VI Reference In"=w3236, "error in"=w3235, "AO1"=w3245, "AO2"=w3246) -> ("error out"=w3234:errorcluster)  [unwired: 1 out]
      }
      event #38 {
        n557 = event-data() -> ()  [unwired: 7 out]
        n558 = local read "Syringe Pump Serial Port"() -> (w3302:refnum<visa-resource-name>)
        n559 = local read "Pump write delay (ms)"() -> (w3303:dbl)
        n560 = case shown="True" "Inject Pump 1 (DNA)" {
          tunnel: w3303 -> [w3308 w3316]
          tunnel: w3302 -> [w3305 w3315]
          frame #0 {
            n561 = flat-sequence {
              tunnel: w3305 -> [w3309]
              tunnel: [w3309] -> w3306
              tunnel: w3308 -> [_]
              tunnel: [w3312] -> w3307
              tunnel: w3306 -> [w3312]
              tunnel: w3307 -> [w3313]
              frame #0 {
                n562 = call "Write to pump.vi"("string"="enter pump1", "VISA resource name"=w3309) -> ()  [unwired: 1 out]
              }
              frame #1 {
                n563 = Wait (ms)(milliseconds to wait="Pump pause delay (ms)") -> ()  [unwired: 1 out]
              }
              frame #2 {
                n564 = call "Write to pump.vi"("string"="stop", "VISA resource name"=w3313) -> ()  [unwired: 1 out]
              }
            }
          }
          frame #1 {
            n565 = flat-sequence {
              tunnel: w3315 -> [w3325]
              tunnel: w3316 -> [w3320]
              tunnel: w3316 -> [w3327]
              tunnel: w3315 -> [w3328]
              frame #0 {
                n566 = local read "All Pump Parameters"() -> (w3319:T4)
                n567 = Unbundle By Name(w3319) -> ("Pump 1"=w3326:T24)
                n568 = call "Set pump parameters.vi"("Pump write delay (ms)"=w3320, "Volume (uL)"="Top Ch Inject Volume (uL)", "Rate (uL/h)"="Top Ch Inject Rate (ul/h)", "Units"=4.0, "Pump #"=1.0, "Pump Parameters In"=w3326, "VISA resource name"=w3325) -> ("Pump Parameters Out"=w3318:T24)  [unwired: 3 in]
                n569 = Bundle By Name(cluster=w3319, "Pump 1"=w3318) -> (w3317:T4)
                n570 = local write "All Pump Parameters"(w3317) -> ()
              }
              frame #1 {
                n571 = Wait (ms)(milliseconds to wait=w3327) -> ()  [unwired: 1 out]
              }
              frame #2 {
                n572 = call "Write to pump.vi"("string"="start", "VISA resource name"=w3328) -> ()  [unwired: 1 out]
              }
            }
          }
        }
      }
      event #39 {
        n573 = event-data() -> ()  [unwired: 7 out]
        n574 = local read "Pump write delay (ms)"() -> (w3331:dbl)
        n575 = case shown="True" "Inject Pump 3" {
          tunnel: w3331 -> [w3336 w3344]
          tunnel: "Syringe Pump Serial Port" -> [w3333 w3343]
          frame #0 {
            n576 = flat-sequence {
              tunnel: w3333 -> [w3337]
              tunnel: [w3337] -> w3334
              tunnel: w3336 -> [_]
              tunnel: [w3340] -> w3335
              tunnel: w3334 -> [w3340]
              tunnel: w3335 -> [w3341]
              frame #0 {
                n577 = call "Write to pump.vi"("string"="enter pump3", "VISA resource name"=w3337) -> ()  [unwired: 1 out]
              }
              frame #1 {
                n578 = local read "Pump pause delay (ms)"() -> (w3339:u32)
                n579 = Wait (ms)(milliseconds to wait=w3339) -> ()  [unwired: 1 out]
              }
              frame #2 {
                n580 = call "Write to pump.vi"("string"="stop", "VISA resource name"=w3341) -> ()  [unwired: 1 out]
              }
            }
          }
          frame #1 {
            n581 = flat-sequence {
              tunnel: w3343 -> [w3353]
              tunnel: w3344 -> [w3348]
              tunnel: w3344 -> [w3355]
              tunnel: w3343 -> [w3356]
              frame #0 {
                n582 = local read "All Pump Parameters"() -> (w3347:T4)
                n583 = Unbundle By Name(w3347) -> ("Pump 3"=w3354:T24)
                n584 = call "Set pump parameters.vi"("Pump write delay (ms)"=w3348, "Volume (uL)"="Bottom Ch Inject Volume (uL)", "Rate (uL/h)"="Bottom Ch Inject Rate (ul/h)", "Units"=4.0, "Pump #"=3.0, "Pump Parameters In"=w3354, "VISA resource name"=w3353) -> ("Pump Parameters Out"=w3346:T24)  [unwired: 3 in]
                n585 = Bundle By Name(cluster=w3347, "Pump 3"=w3346) -> (w3345:T4)
                n586 = local write "All Pump Parameters"(w3345) -> ()
              }
              frame #1 {
                n587 = Wait (ms)(milliseconds to wait=w3355) -> ()  [unwired: 1 out]
              }
              frame #2 {
                n588 = call "Write to pump.vi"("string"="start", "VISA resource name"=w3356) -> ()  [unwired: 1 out]
              }
            }
          }
        }
      }
      event #40 {
        n589 = event-data() -> ()  [unwired: 7 out]
        n590 = local read "Pump write delay (ms)"() -> (w3360:dbl)
        n591 = flat-sequence {
          tunnel: w3358 -> [w3373]
          tunnel: w3360 -> [w3369]
          tunnel: "Inject Pump 2" -> [_]
          tunnel: w3360 -> [w3375]
          tunnel: w3358 -> [w3376]
          frame #0 {
            n592 = local read "All Pump Parameters"() -> (w3368:T4)
            n593 = Multiply(x=60.0, y="Flush Center Ch Rate (ul/m)") -> (x*y=w3365:dbl)
            n594 = Unbundle By Name(w3368) -> ("Pump 2"=w3374:T24)
            n595 = call "Set pump parameters.vi"("Pump write delay (ms)"=w3369, "Volume (uL)"="Flush Center Ch Volume (uL)", "Rate (uL/h)"=w3365, "Units"=3.0, "Pump #"=2.0, "Pump Parameters In"=w3374, "VISA resource name"=w3373) -> ("Pump Parameters Out"=w3367:T24)  [unwired: 3 in]
            n596 = Bundle By Name(cluster=w3368, "Pump 2"=w3367) -> (w3366:T4)
            n597 = local write "All Pump Parameters"(w3366) -> ()
            n598 = Add(x="Flush Center Ch Volume (uL)", y="Total Volume\nFlushed (uL)") -> (x+y=w3362:dbl)
            n599 = local write "Total Volume\nFlushed (uL)"(w3362) -> ()
          }
          frame #1 {
            n600 = Wait (ms)(milliseconds to wait=w3375) -> ()  [unwired: 1 out]
          }
          frame #2 {
            n601 = call "Write to pump.vi"("string"="start", "VISA resource name"=w3376) -> ()  [unwired: 1 out]
          }
        }
        n602 = local read "Syringe Pump Serial Port"() -> (w3358:refnum<visa-resource-name>)
      }
      event #41 {
        n603 = event-data() -> ()  [unwired: 7 out]
        n604 = flat-sequence {
          tunnel: w3384 -> [w3390]
          tunnel: w3383 -> [w3389]
          tunnel: [w3387] -> w3381
          tunnel: [w3386] -> w3380
          tunnel: [w3429] -> w3379
          tunnel: w3381 -> [w3429]
          tunnel: [w3428] -> w3378
          tunnel: w3380 -> [w3428]
          tunnel: w3379 -> [w3433]
          tunnel: w3378 -> [w3432]
          tunnel: [w3431] -> w3382
          frame #0 {
            n605 = xnode "Read/Write Control"("FPGA VI Reference In"=w3390, "error in"=w3389, "Green Filter Flipper"=TRUE) -> ("FPGA VI Reference Out"=w3387:T14, "error out"=w3386:errorcluster)
          }
          frame #1 {
            n606 = Wait (ms)(milliseconds to wait=u32 500) -> ()  [unwired: 1 out]
          }
          frame #2 {
            n607 = xnode "Read/Write Control"("FPGA VI Reference In"=w3433, "error in"=w3432, "Green Filter Flipper"=FALSE) -> ("error out"=w3431:errorcluster)  [unwired: 1 out]
          }
        }
      }
    }
    "error out 2" <- w663
    n608 = node-c288() -> ()  [unwired: 2 out]
  }
  n609 = disable-structure shown="Disabled" {
    disable-tunnel: [w3473 _] -> w183
    disable-tunnel: w77 -> [w3472 _]
    frame #0 {
      n610 = node-c288() -> (w3475:T17)  [unwired: 4 out]
      n611 = timed-loop "Rough control of MCL mirror stage (debugging)" {
        tunnel: w3472 -> [w3478]
        tunnel: [w3477] -> w3473
        timing: w3475 -> [_]
        timing-out: [_] -> w3474
        stop <- w3477 stop-if-true
        n612 = node-c288() -> ()  [unwired: 2 out]
        n613 = case shown="1" "MCL Mode" {
          tunnel: w3478 -> [_ w3481 w3583]
          frame #0 {
          }
          frame #1 {
            n614 = node-c288() -> (w3483:T17)  [unwired: 4 out]
            n615 = timed-loop "Oscillate MCL mirror" {
              timing: w3483 -> [_]
              timing-out: [_] -> w3482
              tunnel: w3481 -> [w3522]
              i -> [w3521]
              stop <- w3484 stop-if-true
              n616 = node-c288() -> (w3520:i64)  [unwired: 1 out]
              n617 = Multiply(x="AO1", y=32767.0) -> (x*y=w3516:dbl)
              n618 = Multiply(x="AO2", y=32767.0) -> (x*y=w3511:dbl)
              n619 = Divide(x=w3516, y=10.0) -> (x/y=w3517:dbl)
              n620 = Divide(x=w3511, y=10.0) -> (x/y=w3512:dbl)
              n621 = To Word Integer(number=w3517) -> (16bit integer=w3509:i16)
              n622 = To Word Integer(number=w3512) -> (16bit integer=w3508:i16)
              n623 = Divide(x=w3520, y=i64 1000) -> (x/y=w3491:dbl)
              n624 = Multiply(x=w3491, y=w3521) -> (x*y=w3502:dbl)
              n625 = Multiply(x="Osc. freq. (Hz) 2", y=6.283185307179586) -> (x*y=w3503:dbl)
              n626 = Multiply(x=w3503, y=w3502) -> (x*y=w3501:dbl)
              n627 = Sine(x=w3501) -> (sin(x)=w3500:dbl)
              n628 = Multiply(x=w3500, y="Osc. amp. (V)") -> (x*y=w3498:dbl)
              n629 = Add(x=w3498, y="Osc. center (V)") -> (x+y=w3496:dbl)
              n630 = Divide(x=w3496, y=10.0) -> (x/y=w3494:dbl)
              n631 = Multiply(x=w3494, y=32767.0) -> (x*y=w3489:dbl)
              n632 = Select(t=w3489, s="Scan axis", f=w3509) -> (s? t:f=w3507:dbl)
              n633 = Select(t=w3508, s="Scan axis", f=w3489) -> (s? t:f=w3506:dbl)
              n634 = local read "MCL Mode"() -> (w3488:u16)
              n635 = Not Equal?(x=w3488, y=u16 1) -> (x != y?=w3485:bool)
              n636 = local read "Stop All"() -> (w3486:bool)
              n637 = xnode "Read/Write Control"("FPGA VI Reference In"=w3522, "AO1"=w3507, "AO2"=w3506) -> ()  [unwired: 1 in, 2 out]
              n638 = Compound Arithmetic op=OR(w3486, w3485) -> (w3484:bool)
              n639 = node-c288() -> ()  [unwired: 2 out]
            }
            n640 = node-c288(w3482) -> ()  [unwired: 1 out]
          }
          frame #2 {
            n641 = case shown="True" "Start Scan" {
              tunnel: w3583 -> [_ w3595]
              frame #0 {
              }
              frame #1 {
                n642 = Subtract(x="End (V)", y="Begin (V)") -> (x-y=w3591:dbl)
                n643 = Decrement(x="N Points") -> (x-1=w3590:dbl)
                n644 = Divide(x=w3591, y=w3590) -> (x/y=w3588:dbl)
                n645 = for {
                  N: "N Points" -> [_]
                  tunnel: "Begin (V)" -> [w3608]
                  tunnel: w3595 -> [w3600]
                  tunnel: [w3599] -> w3594 mode=indexing
                  tunnel: w3588 -> [w3598]
                  tunnel: [w3596] -> w3587 mode=indexing
                  i -> [w3607]
                  n646 = Multiply(x=w3598, y=w3607) -> (x*y=w3606:dbl)
                  n647 = Add(x=w3608, y=w3606) -> (x+y=w3603:dbl)
                  n648 = local read "Scan axis"() -> (w3597:bool)
                  n649 = local read "AO1"() -> (w3605:dbl)
                  n650 = local read "AO2"() -> (w3604:dbl)
                  n651 = Select(t=w3603, s=w3597, f=w3605) -> (s? t:f=w3602:dbl)
                  n652 = Select(t=w3604, s=w3597, f=w3603) -> (s? t:f=w3601:dbl)
                  n653 = flat-sequence {
                    tunnel: w3602 -> [w3612]
                    tunnel: w3601 -> [w3611]
                    tunnel: w3600 -> [w3609]
                    tunnel: [w3677] -> w3599
                    tunnel: [w3676] -> w3596
                    frame #0 {
                      w3615 = 10.0 ("y")
                      w3610 = 32767.0 ("y")
                      n654 = Multiply(x=w3612, y=w3610) -> (x*y=w3618:dbl)
                      n655 = Multiply(x=w3611, y=w3610) -> (x*y=w3616:dbl)
                      n656 = Divide(x=w3618, y=w3615) -> (x/y=w3619:dbl)
                      n657 = Divide(x=w3616, y=w3615) -> (x/y=w3617:dbl)
                      n658 = To Word Integer(number=w3619) -> (16bit integer=w3613:i16)
                      n659 = To Word Integer(number=w3617) -> (16bit integer=w3614:i16)
                      n660 = xnode "Read/Write Control"("FPGA VI Reference In"=w3609, "AO1"=w3613, "AO2"=w3614) -> ()  [unwired: 1 in, 2 out]
                    }
                    frame #1 {
                      n661 = Wait (ms)(milliseconds to wait="DAQ Delay (ms)") -> ()  [unwired: 1 out]
                    }
                    frame #2 {
                      n662 = local read "Slow mean"() -> (w3677:dbl)
                      n663 = local read "Sigma"() -> (w3676:dbl)
                    }
                  }
                }
                n664 = Bundle("Begin (V)"="Begin (V)", w3588, w3594) -> (→"MCL Scan":cluster{"Begin (V)":dbl, dbl, dbl[]})  [unwired: 1 out]
                n665 = Bundle("Begin (V)"="Begin (V)", w3588, w3587) -> (→"MCL Scan 2":cluster{"Begin (V)":dbl, dbl, dbl[]})  [unwired: 1 out]
              }
            }
          }
        }
        n666 = local read "Stop All"() -> (w3477:bool)
        n667 = node-c288() -> ()  [unwired: 2 out]
      }
      n668 = node-c288(w3474) -> ()  [unwired: 1 out]
    }
    frame #1 {
    }
  }
  n669 = timed-loop "Mouse control: trap position (AOM deflection), set confocal spot from image" {
    tunnel: [w3681] -> w134
    tunnel: w77 -> [w3680]
    timing: w21 -> [_]
    timing-out: [_] -> w20
    stop <- w3681 stop-if-true
    n670 = node-c288() -> ()  [unwired: 2 out]
    n671 = event shown="[0] \"Pane\": Mouse Down" {
      selector: _ -> [_ _]
      dyn-events: _ -> [_ _]
      timeout: _ -> [_ _]
      tunnel: w3680 -> [w3684 _]
      event #0 {
        n672 = event-data() -> ("Time"=w3686:u32, "Coords"=w3685:T6, "Button"=w3687:u16)  [unwired: 6 out]
        n673 = case shown="1" w3687 {
          tunnel: w3686 -> [_ _ w3783]
          tunnel: w3685 -> [_ w3717 w3781]
          tunnel: w3684 -> [_ _ w3779]
          frame #0 {
          }
          frame #1 {
            n674 = property on="APD 1" class="ImageControl"() -> ("Displayed Image Position"=w3716:cluster{"Left":i32, "Top":i32})  [unwired: 2 in, 2 out]
            n675 = property on="Detection Laser X" class="ImageControl"() -> ("Displayed Image Position"=w3713:cluster{"Left":i32, "Top":i32})  [unwired: 2 in, 2 out]
            n676 = property on="Detection Laser Y" class="ImageControl"() -> ("Displayed Image Position"=w3712:cluster{"Left":i32, "Top":i32})  [unwired: 2 in, 2 out]
            n677 = property on="APD 1" class="ImageControl"() -> ("Displayed Image Size"=w3714:cluster{"Width":u32, "Height":u32})  [unwired: 2 in, 2 out]
            n678 = property on="Detection Laser X" class="ImageControl"() -> ("Displayed Image Size"=w3715:cluster{"Width":u32, "Height":u32})  [unwired: 2 in, 2 out]
            n679 = property on="Detection Laser Y" class="ImageControl"() -> ("Displayed Image Size"=w3711:cluster{"Width":u32, "Height":u32})  [unwired: 2 in, 2 out]
            n680 = Unbundle By Name(w3714) -> ("Width"=w3708:u32, "Height"=w3707:u32)
            n681 = Unbundle By Name(w3715) -> ("Width"=w3704:u32, "Height"=w3703:u32)
            n682 = Unbundle By Name(w3711) -> ("Width"=w3700:u32, "Height"=w3699:u32)
            n683 = Unbundle By Name(w3716) -> ("Left"=w3710:i32, "Top"=w3709:i32)
            n684 = Unbundle By Name(w3713) -> ("Left"=w3706:i32, "Top"=w3705:i32)
            n685 = Unbundle By Name(w3712) -> ("Left"=w3702:i32, "Top"=w3701:i32)
            n686 = Bundle("Left"=w3710, "Top"=w3709, "Width"=w3708, "Height"=w3707) -> (w3698:T25)  [unwired: 1 in]
            n687 = Bundle("Left"=w3706, "Top"=w3705, "Width"=w3704, "Height"=w3703) -> (w3697:T25)  [unwired: 1 in]
            n688 = Bundle("Left"=w3702, "Top"=w3701, "Width"=w3700, "Height"=w3699) -> (w3696:T25)  [unwired: 1 in]
            n689 = Build Cluster Array(w3698, w3697, w3696) -> (w3695:T26)
            n690 = for {
              tunnel: w3717 -> [w3728]
              tunnel: w3695 -> [w3729] mode=indexing
              shift-right: [w3726] -> w3693
              shift-left: TRUE -> [w3727]
              shift-right: [w3725] -> w3691
              shift-left: _ -> [w3721]
              shift-right: [w3724] -> w3690
              shift-left: _ -> [w3720]
              shift-right: [w3723] -> w3689
              shift-left: _ -> [w3719]
              shift-right: [w3722] -> w3688
              shift-left: _ -> [w3718]
              n691 = case shown="True" w3727 {
                selector: w3727 -> [w3734 _]
                tunnel: w3729 -> [_ w3743]
                tunnel: w3728 -> [_ w3741]
                tunnel: [w3734 w3739] -> w3726
                tunnel: [w3733 w3738] -> w3725
                tunnel: [w3732 w3737] -> w3724
                tunnel: [w3731 w3736] -> w3723
                tunnel: [w3730 w3735] -> w3722
                tunnel: w3721 -> [w3733 _]
                tunnel: w3720 -> [w3732 _]
                tunnel: w3719 -> [w3731 _]
                tunnel: w3718 -> [w3730 _]
                frame #0 {
                }
                frame #1 {
                  n692 = Unbundle(w3743) -> (w3742:T25)
                  n693 = call "isclickinwindow.vi"("Image Param"=w3742, "Point32"=w3741) -> ("4 Y"=w3735:i32, "3 Height"=w3736:i32, "2 X"=w3737:i32, "1 Width"=w3738:i32, "In image?"=w3740:bool)  [unwired: 1 in]
                  n694 = Not(x=w3740) -> (.not. x?=w3739:bool)
                }
              }
            }
            n695 = Not(x=w3693) -> (.not. x?=w3692:bool)
            n696 = case shown="True" w3692 {
              tunnel: w3690 -> [_ w3756]
              tunnel: w3688 -> [_ w3755]
              tunnel: w3691 -> [_ w3754]
              tunnel: w3689 -> [_ w3753]
              frame #0 {
              }
              frame #1 {
                w3749 = FALSE ("Get Point")
                n697 = local read "Scan lines (y)"() -> (w3758:u64)
                n698 = local read "Actual MCL Inc (V)"() -> (w3750:dbl)
                n699 = local read "Scan steps (MCL)"() -> (w3757:u64)
                n700 = Divide "Y Pix/step"(x=w3753, y=w3758) -> (x/y=w3765:dbl)
                n701 = Divide "Y V/pix"(x=w3750, y=w3765) -> (x/y=w3764:dbl)
                n702 = Divide "Y half step offset"(x=w3750, y=2.0) -> (x/y=w3766:dbl)
                n703 = Divide "X pix/step"(x=w3754, y=w3757) -> (x/y=w3763:dbl)
                n704 = Negate(x=w3766) -> (-x=w3767:dbl)
                n705 = local read "Initial Y"() -> (w3773:dbl)
                n706 = Multiply(x=w3755, y=w3764) -> (x*y=w3774:dbl)
                n707 = Divide "X half step offset"(x=w3750, y=2.0) -> (x/y=w3760:dbl)
                n708 = Divide "X V/pix"(x=w3750, y=w3763) -> (x/y=w3762:dbl)
                n709 = Multiply(x=w3750, y=w3757) -> (x*y=w3769:dbl)
                n710 = Compound Arithmetic op=ADD(w3767, w3774, w3773) -> (w3751:dbl)
                "Pointer Y (V)" <- w3751
                n711 = Multiply(x=w3762, y=w3756) -> (x*y=w3771:dbl)
                n712 = Negate(x=w3760) -> (-x=w3759:dbl)
                n713 = local read "Initial X"() -> (w3772:dbl)
                n714 = Negate(x=w3771) -> (-x=w3770:dbl)
                n715 = Compound Arithmetic op=ADD(w3759, w3769, w3772, w3770) -> (w3752:dbl)
                "Pointer X (V)" <- w3752
                n716 = Or(x="Set X Only", y="Set Confocal Spot (X-Y)") -> (x .or. y?=w3745:bool)
                n717 = Or(x="Set Confocal Spot (X-Y)", y="Set Y Only") -> (x .or. y?=w3744:bool)
                n718 = case shown="True" w3745 {
                  tunnel: w3752 -> [_ w3775]
                  frame #0 {
                  }
                  frame #1 {
                    n719 = property on="AO2" class="Slide (strict)"("Val(Sgnl)"=w3775) -> ()  [unwired: 2 in, 2 out]
                  }
                }
                n720 = case shown="True" w3744 {
                  tunnel: w3751 -> [_ w3776]
                  frame #0 {
                  }
                  frame #1 {
                    n721 = property on="AO1" class="Slide (strict)"("Val(Sgnl)"=w3776) -> ()  [unwired: 2 in, 2 out]
                  }
                }
                n722 = local write "Set Confocal Spot (X-Y)"(w3749) -> ()
                n723 = local write "Set X Only"(w3749) -> ()
                n724 = local write "Set Y Only"(w3749) -> ()
              }
            }
          }
          frame #2 {
            n725 = local read "BD 2 Frequency 1 (MHz)"() -> (w3777:dbl)
            n726 = local read "BD 1 Frequency 1 (MHz)"() -> (w3778:dbl)
            n727 = local write "Manipulating Trap"(TRUE ("Manipulating Trap")) -> ()
            n728 = local write "Coords"(T6 {"Horizontal"=0, "Vertical"=0} ("Coords")) -> ()
            n729 = while {
              tunnel: w3783 -> [w3788]
              tunnel: w3781 -> [w3787]
              tunnel: w3779 -> [w3786]
              tunnel: w3778 -> [w3785]
              tunnel: w3777 -> [w3784]
              stop <- w3789 stop-if-true
              n730 = event shown="[0] \"Pane\": Mouse Move" {
                selector: _ -> [_ _]
                dyn-events: _ -> [_ _]
                timeout: _ -> [_ _]
                tunnel: ["Force Manip Abort" w3853] -> w3789
                tunnel: w3788 -> [w3796 _]
                tunnel: w3787 -> [w3794 _]
                tunnel: w3786 -> [w3793 _]
                tunnel: w3785 -> [w3792 _]
                tunnel: w3784 -> [w3791 _]
                event #0 {
                  n731 = event-data() -> ("Time"=w3797:u32, "Coords"=w3798:T6)  [unwired: 3 out]
                  n732 = Less?(x=w3797, y=w3796) -> (x < y?=w3795:bool)
                  n733 = case "Makes sure old motion events prior to mouse click aren't used" shown="False" w3795 {
                    tunnel: w3798 -> [w3840 _]
                    tunnel: w3794 -> [w3841 _]
                    tunnel: w3793 -> [w3818 _]
                    tunnel: w3792 -> [w3814 _]
                    tunnel: w3791 -> [w3813 _]
                    frame #0 {
                      n734 = Subtract(x=w3840, y=w3841) -> (x-y=w3839:T6)
                      "Coords" <- w3839
                      n735 = local read "Y RF Frequency Limits (MHz)"() -> (w3799:T11)
                      n736 = To Double Precision Float(number=w3839) -> (double precision float=w3838:cluster{"Horizontal":dbl, "Vertical":dbl})
                      n737 = Multiply(x=cluster{"Horizontal":dbl, "Vertical":dbl} {"Horizontal"=-1.0, "Vertical"=1.0}, y="Manipulation Scaling") -> (x*y=w3834:cluster{"Horizontal":dbl, "Vertical":dbl})
                      n738 = local read "X RF Frequency Limits (MHz)"() -> (w3800:T11)
                      n739 = Multiply(x=w3838, y=w3834) -> (x*y=w3836:cluster{"Horizontal":dbl, "Vertical":dbl})
                      n740 = Unbundle By Name(w3836) -> ("Horizontal"=w3831:dbl, "Vertical"=w3835:dbl)
                      n741 = Unbundle By Name(w3799) -> ("Maximum"=w3802:dbl, "Minimum"=w3801:dbl)
                      n742 = Boolean To (0,1)(Boolean="Manip. X?") -> (0, 1=w3829:i16)
                      n743 = Boolean To (0,1)(Boolean="Manip. Y?") -> (0, 1=w3826:i16)
                      n744 = Multiply(x=w3835, y=w3826) -> (x*y=w3828:dbl)
                      n745 = Multiply(x=w3829, y=w3831) -> (x*y=w3832:dbl)
                      n746 = local read "BD 1 Frequency 2 (MHz)"() -> (w3816:dbl)
                      n747 = Unbundle By Name(w3800) -> ("Maximum"=w3804:dbl, "Minimum"=w3803:dbl)
                      n748 = local read "BD 2 Frequency 2 (MHz)"() -> (w3815:dbl)
                      n749 = Add(x=w3813, y=w3828) -> (x+y=w3806:dbl)
                      n750 = Add(x=w3814, y=w3832) -> (x+y=w3808:dbl)
                      n751 = In Range and Coerce(upper limit=w3804, x=w3808, lower limit=w3803) -> (coerced(x)=w3807:dbl)  [unwired: 1 out]
                      n752 = In Range and Coerce(upper limit=w3802, x=w3806, lower limit=w3801) -> (coerced(x)=w3805:dbl)  [unwired: 1 out]
                      n753 = Subtract(x=w3807, y=w3816) -> (x-y=w3825:dbl)
                      n754 = Subtract(x=w3805, y=w3815) -> (x-y=w3824:dbl)
                      n755 = Square(x=w3825) -> (x^2=w3823:dbl)
                      n756 = Square(x=w3824) -> (x^2=w3822:dbl)
                      n757 = Add(x=w3823, y=w3822) -> (x+y=w3821:dbl)
                      n758 = Square Root(x=w3821) -> (sqrt(x)=w3817:dbl)
                      n759 = In Range and Coerce(upper limit="Limit Max (MHz)", x=w3817, lower limit="Limit Min (MHz)") -> (In Range?=w3810:bool)  [unwired: 1 out]
                      n760 = Not(x="Limits Enable") -> (.not. x?=w3809:bool)
                      n761 = Or(x=w3810, y=w3809) -> (x .or. y?=w3811:bool)
                      n762 = case shown="True" w3811 {
                        tunnel: w3818 -> [_ w3851]
                        tunnel: w3817 -> [_ w3842]
                        tunnel: w3807 -> [_ w3849]
                        tunnel: w3816 -> [_ w3848]
                        tunnel: w3805 -> [_ w3847]
                        tunnel: w3815 -> [_ w3846]
                        tunnel: w3800 -> [_ w3844]
                        tunnel: w3799 -> [_ w3843]
                        frame #0 {
                        }
                        frame #1 {
                          n763 = local read "BD 1 Frequency 3 (MHz)"() -> (w3850:dbl)
                          n764 = local read "BD 2 Frequency 3 (MHz)"() -> (w3845:dbl)
                          n765 = local write "Trap Delta (MHz)"(w3842) -> ()
                          n766 = property on="Initial delta (MHz)" class="DigNum (strict)"("Val(Sgnl)"=w3842) -> ()  [unwired: 2 in, 2 out]
                          n767 = call "set RF board frequency - interlace.vi"("Board 2 Frequency Limits"=w3843, "Board 1 Frequency Limits"=w3844, "FPGA VI Reference In"=w3851, "Board 2 Frequency 3 (MHz)"=w3845, "Board 1 Frequency 3 (MHz)"=w3850, "Board 2 Frequency 2 (MHz)"=w3846, "Board 2 Frequency 1 (MHz)"=w3847, "Board 1 Frequency 2 (MHz)"=w3848, "Board 1 Frequency 1  (MHz)"=w3849) -> ()  [unwired: 1 in, 2 out]
                          n768 = local write "BD 2 Frequency 1 (MHz)"(w3847) -> ()
                          n769 = local write "BD 1 Frequency 1 (MHz)"(w3849) -> ()
                        }
                      }
                    }
                    frame #1 {
                    }
                  }
                }
                event #1 {
                  n770 = event-data() -> ("Button"=w3852:u16)  [unwired: 8 out]
                  n771 = case shown="3" w3852 {
                    tunnel: [FALSE TRUE] -> w3853
                    frame #0 {
                    }
                    frame #1 {
                      n772 = local write "Manipulating Trap"(FALSE ("Manipulating Trap")) -> ()
                    }
                  }
                }
              }
            }
          }
        }
      }
      event #1 {
        n773 = event-data() -> ()  [unwired: 6 out]
      }
    }
    n774 = local read "Stop All"() -> (w3681:bool)
    n775 = node-c288() -> ()  [unwired: 2 out]
  }
  n776 = timed-loop "Run Scripts, including: stage motion" {
    tunnel: w7 -> [w3857]
    tunnel: w6 -> [w3858]
    tunnel: [w3858] -> w5
    tunnel: [w3857] -> w4
    timing: w2 -> [_]
    timing-out: [_] -> w1
    stop <- w3859 stop-if-true
    n777 = node-c288() -> ()  [unwired: 1 in, 1 out]
    n778 = event shown="[5] \"Data Acq. Spot\": Value Change" {
      selector: _ -> [_ _ _ _ _ _ _ _ _]
      dyn-events: _ -> [_ _ _ _ _ _ _ _ _]
      timeout: _ -> [_ _ _ _ _ _ _ _ _]
      tunnel: ["Set Position" "Move to Position" "Upper Cap." "Lower Cap." _ "Data Acq. Spot" "Dump Beads" _ _] -> _
      tunnel: [_ _ _ _ _ _ _ _ w4084] -> w3859
      tunnel: w3857 -> [w3877 w3885 w3903 w3921 w3939 w3974 w4015 w4058 _]
      tunnel: w3858 -> [w3878 w3886 w3904 w3922 w3940 w3975 w4016 w4059 _]
      event #0 {
        n779 = event-data() -> ()  [unwired: 1 in, 5 out]
        n780 = Build Array("Set Position 1", "Set Position 2", "Set Position 3", "Set Position 4", "Set Position 5") -> (w3876:bool[])
        n781 = Boolean Array To Number(Boolean array=w3876) -> (number=w3875:u32)
        n782 = Logarithm Base 2(1:w3875) -> (0:w3867:dbl)
        n783 = call "Read Stage Position.vi"("error in"=w3877, "VISA resource name in"=w3878) -> ("Current Position"=w3882:cluster{dbl, dbl, dbl}, "error out"=w3881:errorcluster)  [unwired: 2 out]
        n784 = Decrement(x="Position") -> (x-1=w3865:dbl)
        n785 = Greater Or Equal?(x=w3867, y=0.0) -> (x >= y?=w3868:bool)
        n786 = local write "Stage Control Serial Error"(w3881) -> ()
        n787 = Cluster To Array(cluster=w3882) -> (array=w3879:dbl[])
        n788 = Select(t=w3867, s=w3868, f=w3865) -> (s? t:f=w3864:dbl)
        n789 = Increment(x=w3864) -> (x+1=w3863:dbl)
        n790 = Build Array (concatenate)(w3863, w3879) -> (w3862:dbl[])
        n791 = Replace Array Subset(array="Saved Stage Positions", new element=w3862, index (row)=w3864) -> (w3880:dbl[][])  [unwired: 1 in]
        n792 = local write "Saved Stage Positions"(w3880) -> ()
      }
      event #1 {
        n793 = event-data() -> ()  [unwired: 1 in, 5 out]
        n794 = flat-sequence {
          tunnel: w3886 -> [w3889]
          tunnel: w3885 -> [w3888]
          frame #0 {
            n795 = local read "Position"() -> (w3901:dbl)
            n796 = local read "Saved Stage Positions"() -> (w3899:dbl[][])
            n797 = Decrement(x=w3901) -> (x-1=w3898:dbl)
            n798 = Array Subset(array=w3899, index (row)=w3898, length (row)=1 ("length"), index (col)=1 ("index"), length (col)=3 ("length")) -> (w3895:dbl[][])
            n799 = Reshape Array(w3895, 3 ("dimension size")) -> (w3893:dbl[])
            n800 = Array To Cluster(array=w3893) -> (cluster=w3892:cluster{"[0]":dbl, "[1]":dbl, "[2]":dbl})
            n801 = call "Set Stage Position.vi"("Position"=w3892, "error in"=w3888, "VISA resource name in"=w3889) -> ("error out"=w3891:errorcluster)  [unwired: 2 out]
            n802 = local write "Stage Control Serial Error"(w3891) -> ()
            n803 = local write "Stage Moving"(TRUE ("Stage Moving")) -> ()
          }
          frame #1 {
            n804 = call <vilib>:"Beep.vi"() -> ()  [unwired: 3 in, 9 out]
            n805 = local write "Stage Moving"(FALSE ("Stage Moving")) -> ()
          }
        }
      }
      event #2 {
        n806 = event-data() -> ()  [unwired: 1 in, 5 out]
        n807 = flat-sequence {
          tunnel: w3904 -> [w3907]
          tunnel: w3903 -> [w3906]
          frame #0 {
            n808 = local read "Saved Stage Positions"() -> (w3917:dbl[][])
            n809 = Array Subset(array=w3917, index (row)=0 ("index"), length (row)=1 ("length"), index (col)=1 ("index"), length (col)=3 ("length")) -> (w3914:dbl[][])
            n810 = Reshape Array(w3914, 3 ("dimension size")) -> (w3912:dbl[])
            n811 = Array To Cluster(array=w3912) -> (cluster=w3911:cluster{"[0]":dbl, "[1]":dbl, "[2]":dbl})
            n812 = call "Set Stage Position.vi"("Position"=w3911, "error in"=w3906, "VISA resource name in"=w3907) -> ("error out"=w3910:errorcluster)  [unwired: 2 out]
            n813 = local write "Stage Control Serial Error"(w3910) -> ()
            n814 = local write "Stage Moving"(TRUE ("Stage Moving")) -> ()
          }
          frame #1 {
            n815 = local write "Stage Moving"(FALSE ("Stage Moving")) -> ()
            n816 = property on="Trap 2 (ON/OFF)" class="Bool (strict)"("Val(Sgnl)"=TRUE ("Value (Signaling)")) -> ()  [unwired: 2 in, 2 out]
            n817 = call <vilib>:"Beep.vi"() -> ()  [unwired: 3 in, 9 out]
          }
        }
      }
      event #3 {
        n818 = event-data() -> ()  [unwired: 1 in, 5 out]
        n819 = flat-sequence {
          tunnel: w3922 -> [w3925]
          tunnel: w3921 -> [w3924]
          frame #0 {
            n820 = local read "Saved Stage Positions"() -> (w3935:dbl[][])
            n821 = Array Subset(array=w3935, index (row)=1 ("index"), length (row)=1 ("length"), index (col)=1 ("index"), length (col)=3 ("length")) -> (w3932:dbl[][])
            n822 = Reshape Array(w3932, 3 ("dimension size")) -> (w3930:dbl[])
            n823 = Array To Cluster(array=w3930) -> (cluster=w3929:cluster{"[0]":dbl, "[1]":dbl, "[2]":dbl})
            n824 = call "Set Stage Position.vi"("Position"=w3929, "error in"=w3924, "VISA resource name in"=w3925) -> ("error out"=w3928:errorcluster)  [unwired: 2 out]
            n825 = local write "Stage Moving"(TRUE ("Stage Moving")) -> ()
            n826 = local write "Stage Control Serial Error"(w3928) -> ()
          }
          frame #1 {
            n827 = property on="Trap 1 (ON/OFF)" class="Bool (strict)"("Val(Sgnl)"=TRUE ("Value (Signaling)")) -> ()  [unwired: 2 in, 2 out]
            n828 = local write "Stage Moving"(FALSE ("Stage Moving")) -> ()
            n829 = call <vilib>:"Beep.vi"() -> ()  [unwired: 3 in, 9 out]
          }
        }
      }
      event #4 {
        n830 = event-data() -> ()  [unwired: 1 in, 5 out]
        n831 = flat-sequence {
          tunnel: w3939 -> [w3961]
          tunnel: w3940 -> [w3941]
          frame #0 {
            n832 = call "Read Stage Position.vi"("error in"=w3961, "VISA resource name in"=w3941) -> ("Current Position"=w3946:cluster{dbl, dbl, dbl}, "error out"=w3959:errorcluster, "VISA resource name out"=w3960:refnum<visa-resource-name>)  [unwired: 1 out]
            n833 = local read "Saved Stage Positions"() -> (w3970:dbl[][])
            n834 = Divide(x="z nudge increment (um)", y=1000.0) -> (x/y=w3958:dbl)
            n835 = Boolean To (0,1)(Boolean="+z") -> (0, 1=w3950:i16)
            n836 = Boolean To (0,1)(Boolean="-z") -> (0, 1=w3951:i16)
            n837 = Array Subset(array=w3970, index (row)=1 ("index"), length (row)=1 ("length"), index (col)=1 ("index"), length (col)=3 ("length")) -> (w3967:dbl[][])
            n838 = Multiply(x=w3950, y=w3958) -> (x*y=w3954:dbl)
            n839 = Multiply(x=w3951, y=w3958) -> (x*y=w3952:dbl)
            n840 = Unbundle(w3946) -> (w3944:dbl, w3943:dbl, w3947:dbl)
            n841 = Negate(x=w3952) -> (-x=w3953:dbl)
            n842 = Reshape Array(w3967, 3 ("dimension size")) -> (w3965:dbl[])
            n843 = Add(x=w3954, y=w3953) -> (x+y=w3955:dbl)
            n844 = Array To Cluster(array=w3965) -> ()  [unwired: 1 out]
            n845 = Add(x=w3955, y=w3947) -> (x+y=w3945:dbl)
            n846 = Bundle(cluster=w3946, w3944, w3943, w3945) -> (w3942:cluster{dbl, dbl, dbl})
            n847 = call "Set Stage Position.vi"("Position"=w3942, "error in"=w3959, "VISA resource name in"=w3960) -> ("error out"=w3964:errorcluster)  [unwired: 2 out]
            n848 = local write "Stage Moving"(TRUE ("Stage Moving")) -> ()
            n849 = local write "Stage Control Serial Error"(w3964) -> ()
          }
          frame #1 {
            n850 = local write "Stage Moving"(FALSE ("Stage Moving")) -> ()
            n851 = call <vilib>:"Beep.vi"() -> ()  [unwired: 3 in, 9 out]
          }
        }
      }
      event #5 {
        n852 = event-data() -> ()  [unwired: 1 in, 5 out]
        n853 = flat-sequence {
          tunnel: w3975 -> [w3978]
          tunnel: w3974 -> [w3977]
          tunnel: ["Cal @ (MHz)"] -> w3973
          tunnel: w3973 -> [w3998]
          frame #0 {
            n854 = local read "Saved Stage Positions"() -> (w3981:dbl[][])
            n855 = Array Subset(array=w3981, index (row)=2 ("index"), length (row)=1 ("length"), index (col)=1 ("index"), length (col)=3 ("length")) -> (w3984:dbl[][])
            n856 = Reshape Array(w3984, 3 ("dimension size")) -> (w3986:dbl[])
            n857 = local write "Stage Moving"(TRUE ("Stage Moving")) -> ()
            n858 = Array To Cluster(array=w3986) -> (cluster=w3987:cluster{"[0]":dbl, "[1]":dbl, "[2]":dbl})
            n859 = call "Set Stage Position.vi"("Position"=w3987, "error in"=w3977, "VISA resource name in"=w3978) -> ("error out"=w3988:errorcluster)  [unwired: 2 out]
            n860 = local write "Stage Control Serial Error"(w3988) -> ()
          }
          frame #1 {
            n861 = property on="Trap Delta (MHz)" class="DigNum (strict)"("Val(Sgnl)"="Cal @ (MHz)") -> ()  [unwired: 2 in, 2 out]
            n862 = local write "Stage Moving"(FALSE ("Stage Moving")) -> ()
            n863 = call <vilib>:"Beep.vi"() -> ()  [unwired: 3 in, 9 out]
          }
          frame #2 {
            n864 = Wait (ms)(milliseconds to wait=u32 500) -> ()  [unwired: 1 out]
          }
          frame #3 {
            n865 = property on="Save Calibration" class="Bool (strict)"("Val(Sgnl)"=TRUE ("Value (Signaling)")) -> ()  [unwired: 2 in, 2 out]
          }
          frame #4 {
            n866 = Wait (ms)(milliseconds to wait=u32 4000) -> ()  [unwired: 1 out]
          }
          frame #5 {
            n867 = while {
              stop <- w3995 stop-if-true
              n868 = local read "Saving..."() -> (w3996:bool)
              n869 = Wait (ms)(milliseconds to wait=u32 500) -> ()  [unwired: 1 out]
              n870 = Not(x=w3996) -> (.not. x?=w3995:bool)
            }
          }
          frame #6 {
            n871 = case shown="True" "W/ Offset" {
              tunnel: w3998 -> [_ w4003]
              frame #0 {
                n872 = Multiply(x="Cal read wait (s)", y=u32 1000 ("milliseconds to wait")) -> (x*y=w4001:u32)
                n873 = Wait (ms)(milliseconds to wait=w4001) -> ()  [unwired: 1 out]
              }
              frame #1 {
                n874 = flat-sequence {
                  tunnel: w4003 -> [w4011]
                  frame #0 {
                    n875 = property on="Trap Delta (MHz)" class="DigNum (strict)"("Val(Sgnl)"="Offset @ (MHz)") -> ()  [unwired: 2 in, 2 out]
                  }
                  frame #1 {
                    n876 = Wait (ms)(milliseconds to wait=u32 500) -> ()  [unwired: 1 out]
                  }
                  frame #2 {
                    n877 = property on="Trap Raster Scan" class="Bool (strict)"("Val(Sgnl)"=TRUE ("Value (Signaling)")) -> ()  [unwired: 2 in, 2 out]
                  }
                  frame #3 {
                    n878 = Wait (ms)(milliseconds to wait=u32 2000) -> ()  [unwired: 1 out]
                  }
                  frame #4 {
                    n879 = while {
                      stop <- w4009 stop-if-true
                      n880 = local read "Raster Scanning..."() -> (w4010:bool)
                      n881 = Wait (ms)(milliseconds to wait=u32 500) -> ()  [unwired: 1 out]
                      n882 = Not(x=w4010) -> (.not. x?=w4009:bool)
                    }
                  }
                  frame #5 {
                    n883 = property on="Trap Delta (MHz)" class="DigNum (strict)"("Val(Sgnl)"=w4011) -> ()  [unwired: 2 in, 2 out]
                  }
                }
              }
            }
          }
          frame #7 {
            n884 = property on="Read Cal" class="Bool (strict)"("Val(Sgnl)"=TRUE ("Value (Signaling)")) -> ()  [unwired: 2 in, 2 out]
          }
          frame #8 {
            n885 = Wait (ms)(milliseconds to wait=u32 500) -> ()  [unwired: 1 out]
          }
          frame #9 {
            n886 = property on="Fish for Tether" class="Bool (strict)"("Val(Sgnl)"=TRUE ("Value (Signaling)")) -> ()  [unwired: 2 in, 2 out]
          }
        }
      }
      event #6 {
        n887 = event-data() -> ()  [unwired: 1 in, 5 out]
        n888 = flat-sequence {
          tunnel: [w4031] -> w4021
          tunnel: [w4030] -> w4019
          tunnel: [w4029] -> w4017
          tunnel: w4016 -> [w4028]
          tunnel: w4015 -> [w4027]
          tunnel: [w4042] -> w4022
          tunnel: w4021 -> [w4042]
          tunnel: [w4041] -> w4020
          tunnel: w4019 -> [w4041]
          tunnel: [w4040] -> w4018
          tunnel: w4017 -> [w4040]
          tunnel: w4022 -> [w4047]
          tunnel: w4020 -> [w4046]
          tunnel: w4018 -> [w4048]
          frame #0 {
            w4024 = FALSE ("Fl. Triggered...")
            n889 = local read "Saving..."() -> (w4025:bool)
            n890 = local write "Fl. Triggered..."(w4024) -> ()
            n891 = local write "Stage Moving"(TRUE ("Stage Moving")) -> ()
            n892 = property on="Green Laser ON/Interlacing" class="Bool (strict)"("Val(Sgnl)"=w4024) -> ()  [unwired: 2 in, 2 out]
            n893 = local write "Stop Saving"(w4025) -> ()
          }
          frame #1 {
            n894 = local read "Saved Stage Positions"() -> (w4029:dbl[][])
            n895 = Array Subset(array=w4029, index (row)=3 ("index"), length (row)=1 ("length"), index (col)=1 ("index"), length (col)=3 ("length")) -> (w4036:dbl[][])
            n896 = Reshape Array(w4036, 3 ("dimension size")) -> (w4034:dbl[])
            n897 = Array To Cluster(array=w4034) -> (cluster=w4033:cluster{"[0]":dbl, "[1]":dbl, "[2]":dbl})
            n898 = call "Set Stage Position.vi"("Position"=w4033, "error in"=w4027, "VISA resource name in"=w4028) -> ("error out"=w4030:errorcluster, "VISA resource name out"=w4031:refnum<visa-resource-name>)  [unwired: 1 out]
          }
          frame #2 {
            w4043 = FALSE ("Value (Signaling)")
            n899 = property on="Trap 1 (ON/OFF)" class="Bool (strict)"("Val(Sgnl)"=w4043) -> ()  [unwired: 2 in, 2 out]
            n900 = property on="Trap 2 (ON/OFF)" class="Bool (strict)"("Val(Sgnl)"=w4043) -> ()  [unwired: 2 in, 2 out]
            n901 = call <vilib>:"Beep.vi"() -> ()  [unwired: 3 in, 9 out]
          }
          frame #3 {
            n902 = Array Subset(array=w4048, index (row)=1 ("index"), length (row)=1 ("length"), index (col)=1 ("index"), length (col)=3 ("length")) -> (w4052:dbl[][])
            n903 = Reshape Array(w4052, 3 ("dimension size")) -> (w4050:dbl[])
            n904 = Array To Cluster(array=w4050) -> (cluster=w4045:cluster{"[0]":dbl, "[1]":dbl, "[2]":dbl})
            n905 = call "Set Stage Position.vi"("Position"=w4045, "error in"=w4046, "VISA resource name in"=w4047) -> ("error out"=w4044:errorcluster)  [unwired: 2 out]
            n906 = local write "Stage Control Serial Error"(w4044) -> ()
          }
          frame #4 {
            n907 = local write "Stage Moving"(FALSE ("Stage Moving")) -> ()
            n908 = property on="Trap 1 (ON/OFF)" class="Bool (strict)"("Val(Sgnl)"=TRUE ("Value (Signaling)")) -> ()  [unwired: 2 in, 2 out]
            n909 = call <vilib>:"Beep.vi"() -> ()  [unwired: 3 in, 9 out]
          }
        }
      }
      event #7 {
        n910 = event-data() -> ()  [unwired: 1 in, 5 out]
        n911 = Or(x="Move to Position 5", y="Lower Ch. Cap.") -> (x .or. y?=w4061:bool)
        n912 = Build Array("Move to Position 1", "Move to Position 2", "Move to Position 3", "Move to Position 4", w4061) -> (w4064:bool[])
        n913 = Boolean Array To Number(Boolean array=w4064) -> (number=w4063:u32)
        n914 = Logarithm Base 2(1:w4063) -> (0:w4062:dbl)
        n915 = flat-sequence {
          tunnel: w4062 -> [w4073]
          tunnel: w4059 -> [w4071]
          tunnel: w4058 -> [w4070]
          frame #0 {
            n916 = local read "Saved Stage Positions"() -> (w4081:dbl[][])
            n917 = Array Subset(array=w4081, index (row)=w4073, length (row)=1 ("length"), index (col)=1 ("index"), length (col)=3 ("length")) -> (w4078:dbl[][])
            n918 = Reshape Array(w4078, 3 ("dimension size")) -> (w4076:dbl[])
            n919 = Array To Cluster(array=w4076) -> (cluster=w4075:cluster{"[0]":dbl, "[1]":dbl, "[2]":dbl})
            n920 = call "Set Stage Position.vi"("Position"=w4075, "error in"=w4070, "VISA resource name in"=w4071) -> ("error out"=w4074:errorcluster)  [unwired: 2 out]
            n921 = local write "Stage Moving"(TRUE ("Stage Moving")) -> ()
            n922 = local write "Stage Control Serial Error"(w4074) -> ()
          }
          frame #1 {
            n923 = call <vilib>:"Beep.vi"() -> ()  [unwired: 3 in, 9 out]
            n924 = local write "Stage Moving"(FALSE ("Stage Moving")) -> ()
          }
        }
      }
      event #8 {
        n925 = event-data() -> ()  [unwired: 1 in, 5 out]
        n926 = local read "Stop All"() -> (w4084:bool)
      }
    }
    n927 = node-c288() -> ()  [unwired: 1 in, 1 out]
  }
  n928 = flat-sequence "Video" {
    tunnel: [w4093] -> w3
    tunnel: w3 -> [w4133]
    frame #0 {
      n929 = while {
        stop <- w4086 continue-if-true
        n930 = call "Close Video Capture.vi"() -> ("error code OUT"=w4088:i32)
        n931 = Equal?(x=w4088, y=0) -> (x = y?=w4086:bool)
      }
      n932 = local write "Stop All"(FALSE ("Stop All")) -> ()
    }
    frame #1 {
      n933 = call "DMR_Init.vi"() -> ()  [unwired: 3 out]
    }
    frame #2 {
      # "Setting the destination format to Mono8 makes sure that the image can be displayed in the intensity plot."
      n934 = call "DMR_GetDevice.vi"("search string IN"="DE019116701") -> ("device handle OUT"=w4111:i32)  [unwired: 4 in, 2 out]
      n935 = call "DMR_OpenDevice.vi"("device handle IN"=w4111) -> ("driver handle OUT"=w4094:i32)  [unwired: 4 out]
      n936 = call "DMR_FindList.vi"("flags IN"=u32 0 ("flags"), "list name IN"="" ("String"), "list type IN"=T27."camera descriptions", "driver handle IN"=w4094) -> ("list handle OUT"=w4097:i32)  [unwired: 2 out]
      n937 = call "DMR_FindList.vi"("flags IN"=u32 0 ("flags"), "list name IN"="Base", "list type IN"=T27."setting", "driver handle IN"=w4094) -> ("list handle OUT"=w4095:i32)  [unwired: 2 out]
      n938 = call "OBJ_GetHandle.vi"("object name IN"="VideoStandard", "list handle IN"=w4097) -> ("object handle OUT"=w4091:i32)  [unwired: 3 out]
      n939 = call "OBJ_GetHandle.vi"("object name IN"="PixelFormat", "list handle IN"=w4095) -> ("object handle OUT"=w4105:i32)  [unwired: 3 out]
      n940 = call "OBJ_SetS.vi"("value index IN"=0, "value IN"="NTSC M", "object handle IN"=w4091) -> ()  [unwired: 2 out]
      n941 = call "OBJ_SetS.vi"("value index IN"=0, "value IN"="Mono8" ("value"), "object handle IN"=w4105) -> ()  [unwired: 2 out]
      n942 = call "OBJ_GetHandle.vi"("object name IN"="VideoChannel", "list handle IN"=w4095) -> ("object handle OUT"=w4101:i32)  [unwired: 3 out]
      n943 = while {
        tunnel: [w4116] -> w4093
        tunnel: w4094 -> [w4113]
        stop <- w4114 continue-if-true
        n944 = call "DMR_ImageRequestSingle.vi"("request control IN"=0, "driver handle IN"=w4113) -> ("error code OUT"=w4115:i32, "driver handle OUT"=w4116:i32)  [unwired: 2 out]
        n945 = Equal To 0?(x=w4115) -> (x = 0?=w4114:bool)
      }
      n946 = call "OBJ_SetI.vi"("value index IN"=0, "value IN"=3 ("Video channel"), "object handle IN"=w4101) -> ()  [unwired: 2 out]
    }
    frame #3 {
      w4121 = T12 0 items=["Grayscale (U8)", "Grayscale (I16)", "Grayscale (SGL)", "Complex (CSG)", "RGB (U32)", "HSL (U32)", "RGB (U64)"] ("Image Type")
      w4129 = T12 0 items=["Grayscale (U8)", "Grayscale (I16)", "Grayscale (SGL)", "Complex (CSG)", "RGB (U32)", "HSL (U32)", "RGB (U64)"] ("Image Type")
      n947 = for "Create Greyscale map" {
        N: 256 -> [_]
        tunnel: [w4135] -> w4118 mode=indexing
        workers-P: _ -> [_]
        i -> [w4138]
        n948 = To Unsigned Byte Integer(number=w4138) -> (unsigned 8bit integer=w4134:u8)
        n949 = Join Numbers(hi=w4134, lo=w4134) -> ((hi.lo)=w4137:u16)
        n950 = Join Numbers(hi=w4134, lo=w4134) -> ((hi.lo)=w4136:u16)
        n951 = Join Numbers(hi=w4137, lo=w4136) -> ((hi.lo)=w4135:u32)
      }
      n952 = call "IMAQ Create"("Image Name"="Scaled video", "Image Type"=w4121) -> ("New Image"=w4120:T1)  [unwired: 2 in, 2 out]
      n953 = call "IMAQ Create"("Image Name"="Main video", "Image Type"=w4129) -> ("New Image"=w4130:T1)  [unwired: 2 in, 2 out]
      n954 = node-c288() -> (w4128:T17)  [unwired: 4 out]
      n955 = Initialize Array(u32 0 ("Window Number (0...15)"), 480 ("dimension size"), 640 ("dimension size")) -> (w4123:u32[][])
      n956 = timed-loop {
        tunnel: w4133 -> [w4155]
        tunnel: [w4154] -> w4132
        tunnel: w4130 -> [w4153]
        timing: w4128 -> [_]
        timing-out: [_] -> w4127
        tunnel: w4123 -> [w4142]
        tunnel: w4120 -> [w4140]
        tunnel: w4118 -> [w4139]
        stop <- w4141 stop-if-true
        # "This block performs the \nactual image capture."
        n957 = node-c288() -> ()  [unwired: 2 out]
        n958 = local read "Stop All"() -> (w4141:bool)
        n959 = Reciprocal(x="Video Capture Rate (Hz)") -> (1/x=w4145:dbl)
        n960 = Multiply(x=w4145, y=1000.0) -> (x*y=w4143:dbl)
        n961 = call "DMR_ImageRequestWaitFor.vi"("queue number IN"=0, "timeout(ms) IN"=500, "driver handle IN"=w4155) -> ("error code OUT"=w4159:i32, "request number OUT"=w4156:i32, "driver handle OUT"=w4157:i32)
        n962 = feedback #1(T28 refnum ("Avi Refnum")) -> (w4147:T28)
        n963 = case shown="True" "New Video File" {
          tunnel: [T28 refnum ("Avi Refnum") w4176] -> w4149
          tunnel: [FALSE TRUE] -> w4150
          tunnel: w4147 -> [_ w4172]
          frame #0 {
          }
          frame #1 {
            n964 = call "Create new save file.vi"("Ext"=".avi" ("string"), "Index In"="Video Index") -> ("Path Out"=w4168:path, "Index Out"=w4169:dbl)  [unwired: 1 in]
            "Path Out" <- w4168
            n965 = Not Equal?(x=w4172, y=T28 refnum ("Avi Refnum")) -> (x != y?=w4173:bool)
            n966 = Increment(x=w4169) -> (x+1=w4178:dbl)
            n967 = case shown="True" w4173 {
              tunnel: w4172 -> [_ w4179]
              frame #0 {
              }
              frame #1 {
                n968 = call "IMAQ AVI Close"("Avi Refnum"=w4179) -> ()  [unwired: 1 in, 10 out]
              }
            }
            n969 = call "IMAQ AVI Create"("Frames Per Second"=u32 30, "AVI Path"=w4168) -> ("Avi Refnum"=w4176:T28)  [unwired: 5 in, 4 out]
            n970 = local write "Video Index"(w4178) -> ()
          }
        }
        n971 = Equal To 0?(x=w4159) -> (x = 0?=w4158:bool)
        n972 = Select(t=w4149, s=w4150, f=w4147) -> (s? t:f=w4148:T28)
        n973 = case shown="True" w4158 {
          tunnel: w4157 -> [w4180 w4205]
          tunnel: w4156 -> [_ w4204]
          tunnel: [w4180 w4201] -> w4154
          tunnel: w4153 -> [_ w4185]
          tunnel: w4142 -> [_ w4189]
          tunnel: w4148 -> [_ w4187]
          tunnel: w4140 -> [_ w4182]
          tunnel: w4139 -> [_ w4181]
          frame #0 {
          }
          frame #1 {
            w4195 = u32 0 ("X-offset IN")
            n974 = call "DMR_GetImageRequestBufferData.vi"("driver handle IN"=w4205, "request number IN"=w4204) -> ("width OUT"=w4194:i32, "height OUT"=w4193:i32, "driver handle OUT"=w4200:i32, "request number OUT"=w4199:i32, "bytes per pixel OUT"=w4196:i32)  [unwired: 13 out]
            n975 = call "DMR_GetImageRequestBufferImageData.vi"("driver handle IN"=w4200, "request number IN"=w4199, "bytes per pixel IN"=w4196, "X-offset IN"=w4195, "Y-offset IN"=w4195, "height IN"=w4193, "width IN"=w4194) -> ("driver handle OUT"=w4198:u32, "request number OUT"=w4197:u32, "image OUT"=w4190:u32[][])  [unwired: 10 out]
            n976 = call "DMR_ImageRequestUnlock.vi"("request number IN"=w4197, "driver handle IN"=w4198) -> ("driver handle OUT"=w4203:i32)  [unwired: 1 in, 2 out]
            n977 = case shown="True" "Averaging" {
              tunnel: w4190 -> [w4241 w4246]
              tunnel: [w4241 w4245] -> w4186
              tunnel: w4189 -> [_ w4243]
              frame #0 {
              }
              frame #1 {
                (unwired) 1
                w4251 = 1
                n978 = feedback #2(w4243) -> (w4242:u32[][])
                n979 = Add(x=w4246, y=w4242) -> (x+y=w4247:u32[][])
                n980 = Select(t=w4243, s="Reset Averaging", f=w4247) -> (s? t:f=w4249:u32[][])
                n981 = feedback #3(w4251) -> (w4244:i32)
                n982 = Divide(x=w4247, y=w4244) -> (x/y=w4248:dbl[][])
                n983 = Increment(x=w4244) -> (x+1=w4252:i32)
                n984 = To Unsigned Long Integer(number=w4248) -> (unsigned 32bit integer=w4245:u32[][])
                n985 = Select(t=w4251, s="Reset Averaging", f=w4252) -> (s? t:f=w4250:i32)
              }
            }
            n986 = call "DMR_ImageRequestSingle.vi"("request control IN"=0, "driver handle IN"=w4203) -> ("driver handle OUT"=w4201:i32)  [unwired: 3 out]
            n987 = disable-structure shown="Disabled" {
              disable-tunnel: w4186 -> [w4218 _]
              disable-tunnel: w4182 -> [w4217 _]
              frame #0 {
                n988 = To Double Precision Float(number=w4218) -> (double precision float=w4216:dbl[][])
                n989 = In Range and Coerce(upper limit="Intensity Upper", x=w4216, lower limit="Intensity Lower") -> (coerced(x)=w4215:dbl[][])  [unwired: 1 out]
                n990 = Subtract(x="Intensity Upper", y="Intensity Lower") -> (x-y=w4212:dbl)
                n991 = Subtract(x=w4215, y="Intensity Lower") -> (x-y=w4213:dbl[][])
                n992 = Divide(x=w4213, y=w4212) -> (x/y=w4214:dbl[][])
                n993 = Multiply(x=255.0, y=w4214) -> (x*y=w4210:dbl[][])
                n994 = To Unsigned Byte Integer(number=w4210) -> (unsigned 8bit integer=w4219:u8[][])
                n995 = call "IMAQ ArrayToImage"("Image Pixels (U8)"=w4219, "Image"=w4217) -> ("Image Out"=w4206:T1)  [unwired: 4 in, 5 out]
                n996 = First Call?() -> (First Call?: T/F=w4207:bool)
                n997 = case shown="True" w4207 {
                  tunnel: w4206 -> [w4220 w4231]
                  frame #0 {
                    n998 = flat-sequence {
                      tunnel: w4220 -> [w4226]
                      frame #0 {
                        w4223 = FALSE ("Get/Set Status? (Set)")
                        w4222 = 0 ("Window Number (0...15)")
                        n999 = call "IMAQ WindSize"("Get/Set Status? (Set)"=w4223, "Window Number"=w4222) -> ("Width & Height out"=→"Window Size":cluster{"Width":i32, "Height":i32})  [unwired: 4 in, 2 out]
                        n1000 = call "IMAQ WindMove"("Window Number (0...15)"=w4222, "Get/Set Status? (Set)"=w4223) -> ("Coordinates (screen)"=→"Window Position":cluster{"X Position":i32, "Y Position":i32})  [unwired: 3 in, 1 out]
                        n1001 = call "IMAQ WindDraw"("Resize to Image Size? (Y)"=FALSE, "Window Number (0...15)"=w4222, "Image"=w4226) -> ()  [unwired: 7 in, 2 out]
                      }
                      frame #1 {
                        n1002 = call "IMAQ WindZoom 2"("Center Point"="Center Point", "Zoom to Fit? (False)"=FALSE, "Zoom Factor"="Zoom Factor") -> ()  [unwired: 5 in, 4 out]
                      }
                    }
                  }
                  frame #1 {
                    n1003 = flat-sequence {
                      tunnel: w4231 -> [w4234]
                      tunnel: [w4232] -> w4230
                      tunnel: w4230 -> [w4236]
                      frame #0 {
                        w4233 = TRUE ("Resize to Image Size? (Y)")
                        w4232 = 0 ("Window Number (0...15)")
                        n1004 = call "IMAQ WindNonTearing"("Window Number"=w4232, "NonTearing? (True)"=w4233) -> ()  [unwired: 8 in, 2 out]
                        n1005 = call "IMAQ WindDraw"("Resize to Image Size? (Y)"=w4233, "Window Number (0...15)"=w4232, "Image"=w4234) -> ()  [unwired: 7 in, 2 out]
                      }
                      frame #1 {
                        n1006 = call "IMAQ WindSize"("Scrollbars? (N)"=FALSE, "Width & Height"="Initial Window Size", "Window Number"=w4236) -> ()  [unwired: 3 in, 3 out]
                        n1007 = call "IMAQ WindMove"("Window Number (0...15)"=w4236, "Coordinates (screen)"="Initial Window Position") -> ()  [unwired: 3 in, 2 out]
                      }
                    }
                  }
                }
              }
              frame #1 {
              }
            }
            n1008 = To Unsigned Byte Integer(number=w4186) -> (unsigned 8bit integer=w4184:u8[][])
            n1009 = call "IMAQ ArrayToImage"("Image Pixels (U8)"=w4184, "Image"=w4185) -> ("Image Out"=w4183:T1)  [unwired: 4 in, 5 out]
            "Primary Video Display" <- w4183
            n1010 = case shown="True" "Save Video" {
              tunnel: w4187 -> [_ w4240]
              tunnel: w4183 -> [_ w4239]
              frame #0 {
              }
              frame #1 {
                n1011 = call "IMAQ AVI Write Frame"("Image"=w4239, "Avi Refnum"=w4240) -> ()  [unwired: 2 in, 8 out]
              }
            }
            n1012 = case shown="True" "Save Image" {
              tunnel: w4184 -> [_ w4255]
              tunnel: w4181 -> [_ w4254]
              frame #0 {
              }
              frame #1 {
                n1013 = call <vilib>:"Flatten Pixmap.vi"("colors"=w4254, "8-bit pixmap"=w4255) -> ("image data"=w4261:T29)  [unwired: 4 in, 5 out]
                n1014 = call "Create new save file.vi"("Insert"="video_frame_" ("string"), "Ext"=".bmp" ("string"), "Index In"="Image Index") -> ("Path Out"=w4257:path, "Index Out"=w4262:dbl)
                n1015 = Increment(x=w4262) -> (x+1=w4256:dbl)
                n1016 = local write "Image Index"(w4256) -> ()
                n1017 = call <vilib>:"Write BMP File.vi"("image data"=w4261, "path to BMP file"=w4257) -> ()  [unwired: 1 in, 9 out]
              }
            }
          }
        }
        n1018 = node-c288(w4143) -> ()  [unwired: 1 out]
      }
      n1019 = node-c288(w4127) -> ()  [unwired: 1 out]
      n1020 = call "DMR_CloseDevice.vi"("driver handle IN"=w4132) -> ()  [unwired: 1 in, 4 out]
    }
    frame #4 {
      n1021 = call "DMR_Close.vi"() -> ()  [unwired: 1 out]
    }
  }
  n1022 = node-c288() -> (w17:T17)  [unwired: 4 out]
  n1023 = timed-loop "Oscillate AOD (debugging)" {
    tunnel: w77 -> [w4266]
    tunnel: [w4265] -> w22
    timing: w17 -> [_]
    timing-out: [_] -> w16
    stop <- w4265 stop-if-true
    n1024 = node-c288() -> ()  [unwired: 2 out]
    n1025 = event shown="[0] \"Oscillate Set 1\", \"Fish for Tether\": Value Change" {
      selector: _ -> [_ _ _]
      dyn-events: _ -> [_ _ _]
      timeout: _ -> [_ _ _]
      tunnel: w4266 -> [w4273 _ _]
      tunnel: [FALSE ("Stop All") _ w4520] -> w4265
      event #0 {
        n1026 = event-data() -> ()  [unwired: 6 out]
        n1027 = local read "Oscillate Set 1"() -> (w4272:bool)
        n1028 = Or(x=w4272, y="Fish for Tether") -> (x .or. y?=w4270:bool)
        n1029 = case shown="True" w4270 {
          tunnel: w4273 -> [_ w4275]
          tunnel: "Fish for Tether" -> [_ w4274]
          frame #0 {
          }
          frame #1 {
            n1030 = case shown="True" w4274 {
              frame #0 {
              }
              frame #1 {
                n1031 = local write "Scan axis 2"(TRUE) -> ()
                n1032 = local write "Tether"(FALSE ("Tether")) -> ()
              }
            }
            n1033 = node-c288() -> (w4277:T17)  [unwired: 4 out]
            n1034 = timed-loop "Oscillate AOD" {
              timing: w4277 -> [_]
              timing-out: [_] -> w4276
              tunnel: w4275 -> [w4287]
              tunnel: w4274 -> [w4286]
              i -> [w4289]
              stop <- w4285 stop-if-true
              n1035 = node-c288() -> (w4288:i64)  [unwired: 1 out]
              n1036 = flat-sequence {
                tunnel: w4289 -> [w4316]
                tunnel: w4288 -> [w4315]
                tunnel: w4287 -> [w4294]
                tunnel: w4286 -> [w4297]
                tunnel: [w4297] -> w4284
                tunnel: [w4296] -> w4283
                tunnel: [w4293] -> w4282
                tunnel: [w4290] -> w4280
                tunnel: w4284 -> [w4352]
                tunnel: w4283 -> [w4350]
                tunnel: w4282 -> [w4349]
                tunnel: [w4348] -> w4281
                tunnel: w4280 -> [w4347]
                tunnel: [w4400] -> w4285
                tunnel: w4281 -> [w4399]
                frame #0 {
                  n1037 = Divide(x=w4315, y=i64 1000) -> (x/y=w4310:dbl)
                  n1038 = Multiply(x=w4310, y=w4316) -> (x*y=w4312:dbl)
                  n1039 = local read "BD 1 Frequency 2 (MHz)"() -> (w4295:dbl)
                  n1040 = Multiply(x="Osc. freq. (Hz)", y=6.283185307179586) -> (x*y=w4313:dbl)
                  n1041 = Multiply(x=w4313, y=w4312) -> (x*y=w4292:dbl)
                  n1042 = local read "BD 1 Frequency 1 (MHz)"() -> (w4300:dbl)
                  n1043 = case shown="True" w4297 {
                    tunnel: w4292 -> [w4322 w4327]
                    tunnel: w4300 -> [_ w4338]
                    tunnel: w4295 -> [_ w4339]
                    tunnel: [w4319 w4333] -> w4298
                    tunnel: [FALSE w4330] -> w4293
                    tunnel: [0.0 w4323] -> w4290
                    frame #0 {
                      n1044 = Sine(x=w4322) -> (sin(x)=w4320:dbl)
                      n1045 = Multiply(x=w4320, y="Osc. amp. (MHz)") -> (x*y=w4319:dbl)
                    }
                    frame #1 {
                      n1046 = Cosine(x=w4327) -> (cos(x)=w4342:dbl)
                      n1047 = Subtract(x=w4339, y=w4338) -> (x-y=w4337:dbl)
                      n1048 = Decrement(x=w4342) -> (x-1=w4341:dbl)
                      n1049 = Subtract(x=w4337, y="Closest Delta (MHz)") -> (x-y=w4334:dbl)
                      n1050 = Divide(x=w4341, y=-2.0) -> (x/y=w4335:dbl)
                      n1051 = Multiply(x=w4335, y=w4334) -> (x*y=w4333:dbl)
                      n1052 = local read "Vec Mean of T1 T2"() -> (w4329:dbl[])
                      n1053 = Greater?(x=w4329, y="Stop F (pN)") -> (0:w4331:bool[])
                      n1054 = Or Array Elements(Boolean array=w4331) -> (logical OR=w4330:bool)
                      n1055 = Divide(x=w4327, y=6.283185307179586) -> (x/y=w4326:dbl)
                      n1056 = Round Toward +Infinity(x=w4326) -> (ceil(x): smallest int >= x=w4323:dbl)
                      "Attempts" <- w4323
                      n1057 = Greater?(x=w4323, y="Attempt Limit") -> (0:w4325:bool)
                      n1058 = case shown="True" w4325 {
                        frame #0 {
                        }
                        frame #1 {
                          n1059 = call <vilib>:"Beep.vi"() -> ()  [unwired: 3 in, 9 out]
                          n1060 = local write "Fish for Tether"(FALSE ("Fish for Tether")) -> ()
                          n1061 = local read "Messages"() -> (w4344:string)
                          n1062 = call "Update messages.vi"("Message to add"="Tether fishing timeout." ("Messages"), "Old message string"=w4344) -> ("New message string"=→"Messages":string)
                        }
                      }
                    }
                  }
                  n1063 = local read "BD 2 Frequency 1 (MHz)"() -> (w4299:dbl)
                  n1064 = Select(t=w4300, s="Scan axis 2", f=w4299) -> (s? t:f=w4303:dbl)
                  n1065 = Add(x=w4298, y=w4303) -> (x+y=w4296:dbl)
                  n1066 = Select(t=w4296, s="Scan axis 2", f=w4300) -> (s? t:f=w4306:dbl)
                  n1067 = Select(t=w4299, s="Scan axis 2", f=w4296) -> (s? t:f=w4305:dbl)
                  n1068 = local read "Y RF Frequency Limits (MHz)"() -> (w4301:T11)
                  n1069 = local read "X RF Frequency Limits (MHz)"() -> (w4302:T11)
                  n1070 = local read "BD 1 Frequency 3 (MHz)"() -> (w4309:dbl)
                  n1071 = local read "BD 2 Frequency 2 (MHz)"() -> (w4308:dbl)
                  n1072 = local read "BD 2 Frequency 3 (MHz)"() -> (w4307:dbl)
                  n1073 = call "set RF board frequency - interlace.vi"("Board 2 Frequency Limits"=w4301, "Board 1 Frequency Limits"=w4302, "FPGA VI Reference In"=w4294, "Board 2 Frequency 3 (MHz)"=w4307, "Board 1 Frequency 3 (MHz)"=w4309, "Board 2 Frequency 2 (MHz)"=w4308, "Board 2 Frequency 1 (MHz)"=w4305, "Board 1 Frequency 2 (MHz)"=w4295, "Board 1 Frequency 1  (MHz)"=w4306) -> ()  [unwired: 1 in, 2 out]
                }
                frame #1 {
                  n1074 = And(x=w4352, y=w4349) -> (x .and. y?=w4351:bool)
                  n1075 = case "Only if were fishing and now formed tether" shown="True" w4351 {
                    tunnel: w4350 -> [w4354 w4367]
                    tunnel: [w4353 w4366] -> w4348
                    tunnel: w4347 -> [_ w4362]
                    frame #0 {
                      n1076 = local read "Fish for Tether"() -> (w4353:bool)
                      n1077 = case shown="False" w4353 {
                        tunnel: w4354 -> [w4355 _]
                        frame #0 {
                          n1078 = property on="BD 1 Frequency 1 (MHz)" class="DigNum (strict)"("Val(Sgnl)"=w4355) -> ()  [unwired: 2 in, 2 out]
                        }
                        frame #1 {
                        }
                      }
                    }
                    frame #1 {
                      w4366 = FALSE ("Fish for Tether")
                      n1079 = call <vilib>:"Beep.vi"() -> ()  [unwired: 3 in, 9 out]
                      n1080 = Number To Decimal String(number=w4362, width (-)=i16 1) -> (decimal integer string=w4360:string)
                      n1081 = case shown="\"2\", \"3\", \"4\", \"5\", \"6\"" "Then..." {
                        selector: "Then..." -> [_ w4370]
                        tunnel: w4367 -> [w4369 _]
                        frame #0 {
                          n1082 = property on="BD 1 Frequency 1 (MHz)" class="DigNum (strict)"("Val(Sgnl)"=w4369) -> ()  [unwired: 2 in, 2 out]
                        }
                        frame #1 {
                          n1083 = flat-sequence {
                            tunnel: w4370 -> [w4372]
                            frame #0 {
                              n1084 = property on="Trap Delta (MHz)" class="DigNum (strict)"("Val(Sgnl)"="Move to Delta 1 (MHz)") -> ()  [unwired: 2 in, 2 out]
                            }
                            frame #1 {
                              n1085 = case shown="\"5\", \"6\"" w4372 {
                                selector: w4372 -> [w4375 w4385 _]
                                frame #0 {
                                n1086 = flat-sequence {
                                tunnel: w4375 -> [w4376]
                                tunnel: [w4376] -> w4373
                                tunnel: [w4378] -> w4374
                                tunnel: w4373 -> [w4378]
                                tunnel: w4374 -> [w4382]
                                frame #0 {
                                n1087 = property on="Green Laser ON/Interlacing" class="Bool (strict)"("Val(Sgnl)"=TRUE ("Value (Signaling)")) -> ()  [unwired: 2 in, 2 out]
                                }
                                frame #1 {
                                n1088 = Multiply(x="Wait Before Save (s)", y=u32 1000 ("x")) -> (x*y=w4380:u32)
                                n1089 = Wait (ms)(milliseconds to wait=w4380) -> ()  [unwired: 1 out]
                                }
                                frame #2 {
                                n1090 = property on="Start Saving" class="Bool (strict)"("Value"=TRUE ("Start Saving")) -> ()  [unwired: 2 in, 2 out]
                                n1091 = case shown="\"4\"" w4382 {
                                frame #0 {
                                }
                                frame #1 {
                                n1092 = property on="Fl. Triggered..." class="Bool (strict)"("Val(Sgnl)"=TRUE ("Value (Signaling)")) -> ()  [unwired: 2 in, 2 out]
                                }
                                }
                                }
                                }
                                }
                                frame #1 {
                                n1093 = flat-sequence {
                                tunnel: w4385 -> [w4388]
                                frame #0 {
                                n1094 = Wait (ms)(milliseconds to wait=u32 500) -> ()  [unwired: 1 out]
                                }
                                frame #1 {
                                n1095 = property on="Trap Raster Scan" class="Bool (strict)"("Val(Sgnl)"=TRUE ("Value (Signaling)")) -> ()  [unwired: 2 in, 2 out]
                                }
                                frame #2 {
                                n1096 = case shown="\"6\"" w4388 {
                                frame #0 {
                                }
                                frame #1 {
                                n1097 = flat-sequence {
                                frame #0 {
                                n1098 = Wait (ms)(milliseconds to wait=u32 500) -> ()  [unwired: 1 out]
                                }
                                frame #1 {
                                n1099 = while {
                                stop <- w4390 stop-if-true
                                n1100 = local read "Saving..."() -> (w4391:bool)
                                n1101 = Wait (ms)(milliseconds to wait=u32 100) -> ()  [unwired: 1 out]
                                n1102 = Not(x=w4391) -> (.not. x?=w4390:bool)
                                }
                                }
                                frame #2 {
                                n1103 = local read "Tether"() -> (w4393:bool)
                                n1104 = case shown="True" w4393 {
                                frame #0 {
                                }
                                frame #1 {
                                n1105 = flat-sequence {
                                frame #0 {
                                n1106 = property on="Trap Delta (MHz)" class="DigNum (strict)"("Val(Sgnl)"="Move to Delta 2 (MHz)") -> ()  [unwired: 2 in, 2 out]
                                }
                                frame #1 {
                                n1107 = Wait (ms)(milliseconds to wait=u32 500) -> ()  [unwired: 1 out]
                                }
                                frame #2 {
                                n1108 = property on="Green Laser ON/Interlacing" class="Bool (strict)"("Val(Sgnl)"=TRUE ("Green Laser ON/Interlacing")) -> ()  [unwired: 2 in, 2 out]
                                }
                                frame #3 {
                                n1109 = Wait (ms)(milliseconds to wait=u32 500) -> ()  [unwired: 1 out]
                                }
                                frame #4 {
                                n1110 = local write "Start Saving"(TRUE ("Start Saving")) -> ()
                                }
                                }
                                }
                                }
                                }
                                }
                                }
                                }
                                }
                                }
                                }
                                frame #2 {
                                }
                              }
                            }
                          }
                        }
                      }
                      n1111 = Concatenate Strings("Formed tether in ", w4360, " attempt(s)." ("string")) -> (w4357:string)
                      n1112 = local read "Messages"() -> (w4364:string)
                      n1113 = local write "Fish for Tether"(w4366) -> ()
                      n1114 = call "Update messages.vi"("Message to add"=w4357, "Old message string"=w4364) -> ("New message string"=w4363:string)
                      n1115 = local write "Messages"(w4363) -> ()
                      n1116 = Get Date/Time In Seconds() -> (seconds since 1Jan1904=→"Time tether formed":timestamp)
                      "Tether" <- "Tether Alarm?"
                    }
                  }
                }
                frame #2 {
                  n1117 = local read "Oscillate Set 1"() -> (w4404:bool)
                  n1118 = Or(x=w4404, y=w4399) -> (x .or. y?=w4401:bool)
                  n1119 = local read "Stop All"() -> (w4402:bool)
                  n1120 = Not(x=w4401) -> (.not. x?=w4403:bool)
                  n1121 = Compound Arithmetic op=OR(w4402, w4403) -> (w4400:bool)
                }
              }
              n1122 = node-c288() -> ()  [unwired: 2 out]
            }
            n1123 = node-c288(w4276) -> ()  [unwired: 1 out]
          }
        }
      }
      event #1 {
        n1124 = event-data() -> ()  [unwired: 7 out]
        n1125 = case shown="True" "Fl. Triggered..." {
          frame #0 {
          }
          frame #1 {
            n1126 = node-c288() -> (w4414:T17)  [unwired: 4 out]
            n1127 = timed-loop {
              timing: w4414 -> [_]
              timing-out: [_] -> w4413
              tunnel: "Action" -> [w4418]
              shift-right: [w4415] -> _
              shift-left: u8 255 -> [w4417]
              stop <- w4419 stop-if-true
              n1128 = node-c288() -> ()  [unwired: 2 out]
              n1129 = flat-sequence {
                tunnel: w4418 -> [w4427]
                tunnel: w4417 -> [w4423]
                tunnel: [w4422] -> w4416
                tunnel: [w4511] -> w4419
                tunnel: w4416 -> [w4510]
                tunnel: [w4510] -> w4415
                frame #0 {
                  n1130 = local read "Delta Fl. (Hz)"() -> (w4424:dbl)
                  n1131 = Multiply(x="Fl. Delta Thresh. (kHz)", y=1000.0) -> (x*y=w4426:dbl)
                  n1132 = Greater?(x=w4424, y=w4426) -> (0:w4428:bool)
                  n1133 = Or(x=w4428, y="Force Yank") -> (x .or. y?=w4421:bool)
                  n1134 = case shown="True" w4421 {
                    tunnel: w4427 -> [_ w4438]
                    tunnel: w4423 -> [w4430 w4434]
                    tunnel: [w4430 w4431] -> w4422
                    frame #0 {
                    }
                    frame #1 {
                      n1135 = flat-sequence {
                        tunnel: w4435 -> [w4444]
                        tunnel: [w4444] -> w4439
                        tunnel: w4438 -> [w4443]
                        tunnel: [w4443] -> w4437
                        tunnel: [w4442] -> w4436
                        tunnel: w4434 -> [w4441]
                        tunnel: [w4440] -> w4433
                        tunnel: w4439 -> [w4469]
                        tunnel: w4437 -> [w4468]
                        tunnel: w4436 -> [w4467]
                        tunnel: w4433 -> [w4466]
                        tunnel: [w4466] -> w4432
                        tunnel: w4432 -> [w4508]
                        tunnel: [w4508] -> w4431
                        frame #0 {
                          n1136 = call <vilib>:"Beep.vi"() -> ()  [unwired: 3 in, 9 out]
                          n1137 = local write "Waiting"(FALSE ("Waiting")) -> ()
                          n1138 = Increment(x=w4441) -> (x+1=w4440:u8)
                          n1139 = case shown="\"Yank\"" w4443 {
                            tunnel: w4440 -> [_ _ w4450]
                            frame #0 {
                              n1140 = property on="Confocal Image" class="Bool (strict)"("Val(Sgnl)"=TRUE ("Value (Signaling)")) -> ()  [unwired: 2 in, 2 out]
                            }
                            frame #1 {
                            }
                            frame #2 {
                              n1141 = flat-sequence {
                                tunnel: w4450 -> [w4453]
                                tunnel: [w4452] -> w4449
                                tunnel: ["N Array El"] -> w4448
                                tunnel: w4449 -> [w4463]
                                tunnel: w4448 -> [w4459]
                                frame #0 {
                                n1142 = Multiply(x="Yank Delay (s)", y=1000.0) -> (x*y=w4456:dbl)
                                n1143 = Quotient & Remainder(x=w4453, y="N Array El") -> (x-y*floor(x/y)=w4452:u8)  [unwired: 1 out]
                                n1144 = Wait (ms)(milliseconds to wait=w4456) -> ()  [unwired: 1 out]
                                }
                                frame #1 {
                                n1145 = Random Number (0-1)() -> (number: 0 to 1=w4460:dbl)
                                n1146 = Multiply(x=w4459, y=w4460) -> (x*y=w4458:dbl)
                                n1147 = Round Toward -Infinity(1:w4458) -> (0:w4457:dbl)
                                n1148 = Select(t=w4457, s="Random Choice", f=w4463) -> (s? t:f=w4461:dbl)
                                n1149 = Index Array(array="Yank to Delta Array (MHz)", index=w4461) -> (element=w4464:dbl)
                                n1150 = property on="Trap Delta (MHz)" class="DigNum (strict)"("Val(Sgnl)"=w4464) -> ()  [unwired: 2 in, 2 out]
                                }
                              }
                            }
                          }
                          n1151 = local read "Time (s)"() -> (w4442:dbl)
                          "Fl. High" <- TRUE ("Yanking")
                        }
                        frame #1 {
                          n1152 = node-c288() -> (w4471:T17)  [unwired: 4 out]
                          n1153 = timed-loop {
                            timing: w4471 -> [_]
                            timing-out: [_] -> w4470
                            tunnel: w4469 -> [w4484]
                            tunnel: w4468 -> [w4482]
                            tunnel: w4467 -> [w4481]
                            stop <- w4483 stop-if-true
                            n1154 = node-c288() -> ()  [unwired: 2 out]
                            n1155 = local read "Fl. Delta Thresh. (kHz)"() -> (w4476:dbl)
                            n1156 = local read "Fl. Triggered..."() -> (w4485:bool)
                            n1157 = local read "Delta Fl. (Hz)"() -> (w4475:dbl)
                            n1158 = local read "Stop All"() -> (w4479:bool)
                            n1159 = Not(x=w4485) -> (.not. x?=w4480:bool)
                            n1160 = Multiply(x=w4476, y=1000.0) -> (x*y=w4474:dbl)
                            n1161 = Negate(x=w4474) -> (-x=w4473:dbl)
                            n1162 = Less?(x=w4475, y=w4473) -> (x < y?=w4478:bool)
                            n1163 = Compound Arithmetic op=OR(w4478, w4479, w4480, "Force Reset") -> (w4483:bool)
                            n1164 = case shown="True" w4483 {
                              tunnel: w4484 -> [_ w4496]
                              tunnel: w4482 -> [_ w4495]
                              tunnel: w4481 -> [_ w4493]
                              frame #0 {
                              }
                              frame #1 {
                                n1165 = case shown="\"Yank\"" w4495 {
                                tunnel: w4496 -> [_ w4497]
                                frame #0 {
                                }
                                frame #1 {
                                n1166 = flat-sequence {
                                tunnel: [w4502] -> w4498
                                tunnel: w4497 -> [w4502]
                                tunnel: w4498 -> [w4503]
                                frame #0 {
                                n1167 = local read "Yank Delay (s)"() -> (w4501:dbl)
                                n1168 = Multiply(x=w4501, y=1000.0) -> (x*y=w4499:dbl)
                                n1169 = Wait (ms)(milliseconds to wait=w4499) -> ()  [unwired: 1 out]
                                }
                                frame #1 {
                                n1170 = property on="Trap Delta (MHz)" class="DigNum (strict)"("Val(Sgnl)"=w4503) -> ()  [unwired: 2 in, 2 out]
                                }
                                }
                                }
                                }
                                n1171 = local read "Time (s)"() -> (w4494:dbl)
                                n1172 = Subtract(x=w4494, y=w4493) -> (x-y=w4490:dbl)
                                "Duration (s)" <- w4490
                                n1173 = Number To Decimal String(number=w4490, width (-)=i16 0) -> (decimal integer string=w4488:string)
                                n1174 = Concatenate Strings(w4488, " s fluorescence event." ("string")) -> (w4486:string)
                                n1175 = local read "Messages"() -> (w4492:string)
                                n1176 = call "Update messages.vi"("Message to add"=w4486, "Old message string"=w4492) -> ("New message string"=w4491:string)
                                n1177 = call <vilib>:"Beep.vi"() -> ()  [unwired: 3 in, 9 out]
                                n1178 = local write "Messages"(w4491) -> ()
                              }
                            }
                            n1179 = node-c288() -> ()  [unwired: 2 out]
                          }
                          n1180 = node-c288(w4470) -> ()  [unwired: 1 out]
                        }
                        frame #2 {
                          n1181 = local write "Fl. High"(FALSE ("Yanking")) -> ()
                        }
                      }
                      n1182 = local read "Trap Delta (MHz)"() -> (w4435:dbl)
                    }
                  }
                }
                frame #1 {
                  n1183 = local read "Stop All"() -> (w4514:bool)
                  n1184 = local read "Fl. Triggered..."() -> (w4512:bool)
                  n1185 = Not(x=w4512) -> (.not. x?=w4513:bool)
                  n1186 = Or(x=w4513, y=w4514) -> (x .or. y?=w4511:bool)
                  n1187 = Not(x=w4511) -> (.not. x?=→"Waiting":bool)
                }
              }
              n1188 = node-c288() -> ()  [unwired: 2 out]
            }
            n1189 = node-c288(w4413) -> ()  [unwired: 1 out]
          }
        }
      }
      event #2 {
        n1190 = event-data() -> ()  [unwired: 7 out]
        n1191 = local read "Stop All"() -> (w4520:bool)
      }
    }
    n1192 = node-c288() -> ()  [unwired: 2 out]
  }
  n1193 = node-c288(i64 1 ("Period")) -> (w127:T17)  [unwired: 3 out]
  n1194 = timed-loop "Acquire Data" {
    tunnel: w74 -> [w4696]
    tunnel: w73 -> [w4695]
    tunnel: [w4733] -> w227
    tunnel: [w4727] -> w225
    timing: w127 -> [_]
    timing-out: [_] -> w126
    tunnel: w13 -> [w4528]
    tunnel: w9 -> [w4526]
    tunnel: w8 -> [w4525]
    stop <- "Stop All" stop-if-true
    w4578 = "NI_ChannelName" ("name")
    n1195 = node-c288() -> ()  [unwired: 2 out]
    n1196 = case "Reset data stream" shown="True" "Reset" {
      tunnel: w4696 -> [w6923 w6930]
      tunnel: w4695 -> [w6922 w6929]
      tunnel: [w6923 w6925] -> w4691
      tunnel: [w6922 w6924] -> w4690
      frame #0 {
      }
      frame #1 {
        w6928 = TRUE ("AI to FIFO")
        w6935 = FALSE ("AI to FIFO")
        n1197 = local write "Overflow (data lost)"(FALSE ("Overflow (data lost)")) -> ()
        n1198 = xnode "Read/Write Control"("FPGA VI Reference In"=w6930, "error in"=w6929, "AI to FIFO"=w6935, "APD to FIFO"=w6935) -> ("FPGA VI Reference Out"=w6933:T14, "error out"=w6934:errorcluster)
        n1199 = xnode "Invoke Method"("FPGA VI Reference In"=w6933, "error in"=w6934) -> ("FPGA VI Reference Out"=w6931:T14, "error out"=w6932:errorcluster)
        n1200 = xnode "Invoke Method"("FPGA VI Reference In"=w6931, "error in"=w6932) -> ("FPGA VI Reference Out"=w6927:T14, "error out"=w6926:errorcluster)
        n1201 = xnode "Read/Write Control"("FPGA VI Reference In"=w6927, "error in"=w6926, "AI to FIFO"=w6928, "APD to FIFO"=w6928) -> ("FPGA VI Reference Out"=w6925:T14, "error out"=w6924:errorcluster)
      }
    }
    n1202 = Or(x="Start AOD Scan", y="Trap Raster Scan") -> (x .or. y?=w4638:bool)
    n1203 = And(x="Save scans", y=w4638) -> (x .and. y?=w4687:bool)
    n1204 = case "Start AOM raster scan" shown="True" w4638 {
      tunnel: w4691 -> [w6161 w6171]
      tunnel: w4690 -> [w6160 w6170]
      tunnel: [w6161 w6164] -> w4689
      tunnel: [w6160 w6163] -> w4688
      frame #0 {
      }
      frame #1 {
        n1205 = case shown="True" "Restart DMA? (AOD)" {
          tunnel: [w6537 w6538] -> w6165
          tunnel: [w6536 w6539] -> w6166
          tunnel: w6171 -> [w6537 w6545]
          tunnel: w6170 -> [w6536 w6544]
          frame #0 {
          }
          frame #1 {
            w6541 = FALSE ("AI to FIFO")
            n1206 = xnode "Read/Write Control"("FPGA VI Reference In"=w6545, "error in"=w6544, "AI to FIFO"=w6541, "APD to FIFO"=w6541) -> ("FPGA VI Reference Out"=w6543:T14, "error out"=w6542:errorcluster)
            n1207 = xnode "Invoke Method"("FPGA VI Reference In"=w6543, "error in"=w6542) -> ("FPGA VI Reference Out"=w6547:T14, "error out"=w6546:errorcluster)
            n1208 = xnode "Invoke Method"("FPGA VI Reference In"=w6547, "error in"=w6546) -> ("FPGA VI Reference Out"=w6538:T14, "error out"=w6539:errorcluster)
            n1209 = local write "Overflow (data lost)"(FALSE ("Overflow (data lost)")) -> ()
          }
        }
        n1210 = case shown="True" "Move MCL Also?" {
          tunnel: w6166 -> [w6174 w6280]
          tunnel: w6165 -> [w6175 w6281]
          tunnel: [w6173 w6284] -> w6164
          tunnel: [w6172 w6283] -> w6163
          frame #0 {
            w6176 = TRUE ("AI to FIFO")
            n1211 = xnode "Read/Write Control"("FPGA VI Reference In"=w6175, "error in"=w6174, "AI to FIFO"=w6176, "APD to FIFO"=w6176, "Start scan"=w6176) -> ("FPGA VI Reference Out"=w6173:T14, "error out"=w6172:errorcluster)
          }
          frame #1 {
            w6277 = FALSE ("1D or 2D Scan?")
            w6282 = TRUE ("AI to FIFO")
            # "Count for MCL loop"
            # "N total cycles"
            # "N steps"
            # "V_int"
            n1212 = local read "Scan Range (nm)"() -> (w6259:dbl)
            n1213 = local read "Number of F/B Scans (AOD)"() -> (w6276:u16)
            n1214 = Sign(1:w6259) -> (0:w6258:dbl)
            n1215 = Compound Arithmetic op=MULTIPLY(w6259, "MCL Step Position Ratio", "MCL/AOM Scale Tweak") -> (w6263:dbl)
            n1216 = Negate(x=w6258) -> (-x=w6255:dbl)
            n1217 = Multiply(x=w6255, y="MCL Step Increment (V_int)") -> (x*y=w6257:dbl)
            n1218 = Divide(x=w6263, y="MCL X Cal (nm/V)") -> (x/y=w6269:dbl)
            n1219 = Multiply(x=32767.0 ("y"), y=w6269) -> (x*y=w6275:dbl)
            n1220 = local read "Total Counts (ticks)"() -> (w6260:u32)
            n1221 = local read "Cycles/step (AOD)"() -> (w6271:u64)
            n1222 = local read "Scan steps (AOD)"() -> (w6272:u64)
            n1223 = Divide(x=w6275, y=10.0) -> (x/y=w6268:dbl)
            n1224 = Divide(x=w6268, y="MCL Step Increment (V_int)") -> (x/y=w6266:dbl)
            n1225 = Absolute Value(x=w6266) -> (abs(x)=w6254:dbl)
            n1226 = Compound Arithmetic op=MULTIPLY(w6272, w6271, w6260) -> (w6267:u64)
            n1227 = local write "wait to reset values"(w6282) -> ()
            n1228 = local write "MCL Scanning"(w6282) -> ()
            n1229 = Divide(x=w6267, y=w6254) -> (x/y=w6264:dbl)
            "MCL Count" <- w6264
            n1230 = xnode "Read/Write Control"("FPGA VI Reference In"=w6281, "error in"=w6280, "Scan steps (MCL)"=w6254, "Number of scans (MCL)"=w6276, "Cycles per step (MCL)"=u64 1, "Scan freq.  increment (MCL)"=w6257, "1D or 2D Scan?"=w6277, "MCL Scan Axis"=w6277, "Cont. Scan (MCL)"=w6277, "MCL count"=w6264) -> ("FPGA VI Reference Out"=w6279:T14, "error out"=w6278:errorcluster)
            n1231 = xnode "Read/Write Control"("FPGA VI Reference In"=w6279, "error in"=w6278, "AI to FIFO"=w6282, "APD to FIFO"=w6282, "Start scan"=w6282, "Start scan (MCL)"=w6282) -> ("FPGA VI Reference Out"=w6284:T14, "error out"=w6283:errorcluster)
          }
        }
        n1232 = local write "Trap Raster Scan"(FALSE ("Trap Raster Scan")) -> ()
        "Raster Scanning..." <- TRUE ("Scanning...")
      }
    }
    n1233 = Compound Arithmetic op=OR("Start MCL Scan", "Confocal Image", "Confocal Linescan") -> (w4636:bool)
    n1234 = And(x="Save Data (MCL)", y=w4636) -> (x .and. y?=w4686:bool)
    n1235 = case "Start MCL raster scan" shown="True" w4636 {
      tunnel: w4689 -> [w5345 w5360]
      tunnel: w4688 -> [w5344 w5359]
      tunnel: [w5345 w5355] -> w4573
      tunnel: [w5344 w5354] -> w4572
      tunnel: [FALSE w5353] -> w4672
      tunnel: "Start MCL Scan" -> [_ w5348]
      tunnel: "Confocal Image" -> [_ w5347]
      tunnel: "Confocal Linescan" -> [_ _]
      frame #0 {
      }
      frame #1 {
        w5353 = TRUE
        n1236 = case shown="True" "Restart DMA? (MCL)" {
          tunnel: [w5597 w5600] -> w5358
          tunnel: [w5596 w5599] -> w5357
          tunnel: w5360 -> [w5597 w5605]
          tunnel: w5359 -> [w5596 w5604]
          frame #0 {
          }
          frame #1 {
            w5601 = FALSE ("AI to FIFO")
            n1237 = xnode "Read/Write Control"("FPGA VI Reference In"=w5605, "error in"=w5604, "AI to FIFO"=w5601, "APD to FIFO"=w5601) -> ("FPGA VI Reference Out"=w5603:T14, "error out"=w5602:errorcluster)
            n1238 = xnode "Invoke Method"("FPGA VI Reference In"=w5603, "error in"=w5602) -> ("FPGA VI Reference Out"=w5607:T14, "error out"=w5606:errorcluster)
            n1239 = xnode "Invoke Method"("FPGA VI Reference In"=w5607, "error in"=w5606) -> ("FPGA VI Reference Out"=w5600:T14, "error out"=w5599:errorcluster)
            n1240 = local write "Overflow (data lost)"(FALSE ("Overflow (data lost)")) -> ()
          }
        }
        n1241 = case shown="False" w5348 {
          selector: w5348 -> [_ w5364]
          tunnel: w5347 -> [w5363 _]
          tunnel: [w5363 w5364] -> w5346
          frame #0 {
            n1242 = property on="2D or 1D Scan" class="Bool (strict)"("Val(Sgnl)"=w5363) -> ()  [unwired: 2 in, 2 out]
            n1243 = property on="Confocal Image" class="Bool (strict)"("Value"=FALSE ("Start Confocal Map")) -> ()  [unwired: 2 in, 2 out]
          }
          frame #1 {
          }
        }
        n1244 = local write "MCL Scanning"(w5353) -> ()
        n1245 = local read "AO1"() -> (w5350:dbl)
        n1246 = local read "AO2"() -> (w5349:dbl)
        n1247 = case shown="True" "Center Scan" {
          tunnel: w5358 -> [w5371 w5480]
          tunnel: w5357 -> [w5370 w5479]
          tunnel: [w5369 w5478] -> w5355
          tunnel: [w5368 w5477] -> w5354
          tunnel: [w5366 w5464] -> w5352
          tunnel: [w5365 w5463] -> w5351
          tunnel: w5350 -> [w5366 w5469]
          tunnel: w5349 -> [w5365 w5472]
          tunnel: w5346 -> [_ _]
          frame #0 {
            w5367 = TRUE ("AI to FIFO")
            n1248 = xnode "Read/Write Control"("FPGA VI Reference In"=w5371, "error in"=w5370, "AI to FIFO"=w5367, "APD to FIFO"=w5367, "Start scan (MCL)"=w5367) -> ("FPGA VI Reference Out"=w5369:T14, "error out"=w5368:errorcluster)
          }
          frame #1 {
            w5476 = TRUE ("AI to FIFO")
            n1249 = local read "Scan steps (MCL)"() -> (w5455:u64)
            n1250 = local read "Scan lines (y)"() -> (w5451:u64)
            n1251 = local read "Fast Scan Dir"() -> (w5462:bool)
            n1252 = local read "Actual MCL Inc (V)"() -> (w5452:dbl)
            n1253 = Decrement(x=w5451) -> (x-1=w5450:u64)
            n1254 = Decrement(x=w5455) -> (x-1=w5454:u64)
            n1255 = Multiply(x=w5452, y=w5450) -> (x*y=w5449:dbl)
            n1256 = Divide(x=w5449, y=2.0) -> (x/y=w5459:dbl)
            n1257 = Multiply(x=w5452, y=w5454) -> (x*y=w5453:dbl)
            n1258 = Divide(x=w5453, y=2.0) -> (x/y=w5458:dbl)
            n1259 = Select(t=w5458, s=w5462, f=w5459) -> (s? t:f=w5457:dbl)
            n1260 = Select(t=w5459, s=w5462, f=w5458) -> (s? t:f=w5461:dbl)
            n1261 = Subtract(x=w5469, y=w5461) -> (x-y=w5460:dbl)
            n1262 = Subtract(x=w5472, y=w5457) -> (x-y=w5456:dbl)
            n1263 = local read "2D or 1D Scan"() -> (w5474:bool)
            n1264 = Not(x=w5462) -> (.not. x?=w5468:bool)
            n1265 = Not(x=w5474) -> (.not. x?=w5470:bool)
            n1266 = And(x=w5462, y=w5470) -> (x .and. y?=w5471:bool)
            n1267 = And(x=w5470, y=w5468) -> (x .and. y?=w5473:bool)
            n1268 = Select(t=w5472, s=w5473, f=w5456) -> (s? t:f=w5463:dbl)
            n1269 = Select(t=w5469, s=w5471, f=w5460) -> (s? t:f=w5464:dbl)
            n1270 = call "Volt to I16.vi"("Voltage In"=w5464) -> ("I16 Voltage Out"=w5467:i16)
            n1271 = call "Volt to I16.vi"("Voltage In"=w5463) -> ("I16 Voltage Out"=w5466:i16)
            n1272 = xnode "Read/Write Control"("FPGA VI Reference In"=w5480, "error in"=w5479, "AI to FIFO"=w5476, "APD to FIFO"=w5476, "Start scan (MCL)"=w5476, "AO1"=w5467, "AO2"=w5466) -> ("FPGA VI Reference Out"=w5478:T14, "error out"=w5477:errorcluster)
          }
        }
        "Initial Y" <- w5352
        "Initial X" <- w5351
        "wait to reset values" <- w5353
      }
    }
    n1273 = local read "APD Elements/DMA read"() -> (w4541:u32)
    n1274 = local read "Elements/DMA read"() -> (w4596:u32)
    n1275 = xnode "Get APD Data"("FPGA VI Reference In"=w4573, "error in"=w4572, "Number of Elements"=w4541, "Timeout (ms)"=-1) -> ("Data"=w4540:u32[], "Elements Remaining"=→"APD FIFO Elements Remaining":u32)  [unwired: 2 out]
    n1276 = xnode "Get Trap Data"("FPGA VI Reference In"=w4573, "error in"=w4572, "Number of Elements"=w4596, "Timeout (ms)"=-1 ("Timeout")) -> ("FPGA VI Reference Out"=w4575:T14, "error out"=w4574:errorcluster, "Data"=w4712:u32[], "Elements Remaining"=w4742:u32)
    "FIFO El. Rem." <- w4742
    n1277 = local read "FIFO Depth"() -> (w4744:u32)
    n1278 = Subtract(x=w4744, y=w4596) -> (x-y=w4743:u32)
    n1279 = Divide(x=w4742, y=w4743) -> (x/y=w4741:dbl)
    "Buffer Status" <- w4741
    n1280 = Equal?(x=w4741, y=1.0) -> (x = y?=w4739:bool)
    n1281 = case "Alert buffer overflow" shown="True" w4739 {
      frame #0 {
      }
      frame #1 {
        n1282 = call <vilib>:"Beep.vi"() -> ()  [unwired: 3 in, 9 out]
        "Overflow (data lost)" <- TRUE ("Overflow (data lost)")
      }
    }
    n1283 = local read "FPGA Averaging"() -> (w4595:bool)
    n1284 = case "Special unpacking case if no averaging done by FPGA" shown="False" w4595 {
      tunnel: w4712 -> [w5757 w5783]
      tunnel: [w5728 w5758] -> w4711
      frame #0 {
        n1285 = Decimate 1D Array(w5757) -> (w5756:u32[], w5755:u32[], w5754:u32[], w5753:u32[])
        n1286 = Split Number(x=w5756) -> (hi(x)=w5752:u16[], lo(x)=w5751:u16[])
        n1287 = Split Number(x=w5755) -> (hi(x)=w5750:u16[], lo(x)=w5749:u16[])
        n1288 = Split Number(x=w5754) -> (hi(x)=w5748:u16[], lo(x)=w5747:u16[])
        n1289 = Split Number(x=w5753) -> (hi(x)=w5746:u16[], lo(x)=w5745:u16[])
        n1290 = To Word Integer(number=w5752) -> (16bit integer=w5744:i16[])
        n1291 = To Word Integer(number=w5751) -> (16bit integer=w5743:i16[])
        n1292 = To Word Integer(number=w5750) -> (16bit integer=w5742:i16[])
        n1293 = To Word Integer(number=w5749) -> (16bit integer=w5741:i16[])
        n1294 = To Word Integer(number=w5748) -> (16bit integer=w5740:i16[])
        n1295 = To Word Integer(number=w5747) -> (16bit integer=w5739:i16[])
        n1296 = To Word Integer(number=w5746) -> (16bit integer=w5738:i16[])
        n1297 = To Word Integer(number=w5745) -> (16bit integer=w5737:i16[])
        n1298 = To Double Precision Float(number=w5744) -> (double precision float=w5736:dbl[])
        n1299 = To Double Precision Float(number=w5743) -> (double precision float=w5735:dbl[])
        n1300 = To Double Precision Float(number=w5742) -> (double precision float=w5734:dbl[])
        n1301 = To Double Precision Float(number=w5741) -> (double precision float=w5733:dbl[])
        n1302 = To Double Precision Float(number=w5740) -> (double precision float=w5732:dbl[])
        n1303 = To Double Precision Float(number=w5739) -> (double precision float=w5731:dbl[])
        n1304 = To Double Precision Float(number=w5738) -> (double precision float=w5730:dbl[])
        n1305 = To Double Precision Float(number=w5737) -> (double precision float=w5729:dbl[])
        n1306 = Interleave 1D Arrays(w5736, w5735, w5734, w5733, w5732, w5731, w5730, w5729) -> (w5728:dbl[])
      }
      frame #1 {
        n1307 = Decimate 1D Array(w5783) -> (w5774:u32[], w5772:u32[], w5770:u32[], w5768:u32[], w5766:u32[], w5764:u32[], w5762:u32[], w5760:u32[])
        n1308 = To Long Integer(number=w5774) -> (32bit integer=w5782:i32[])
        n1309 = To Long Integer(number=w5772) -> (32bit integer=w5781:i32[])
        n1310 = To Long Integer(number=w5770) -> (32bit integer=w5780:i32[])
        n1311 = To Long Integer(number=w5768) -> (32bit integer=w5779:i32[])
        n1312 = To Long Integer(number=w5766) -> (32bit integer=w5778:i32[])
        n1313 = To Long Integer(number=w5764) -> (32bit integer=w5777:i32[])
        n1314 = To Long Integer(number=w5762) -> (32bit integer=w5776:i32[])
        n1315 = To Long Integer(number=w5760) -> (32bit integer=w5775:i32[])
        n1316 = To Double Precision Float(number=w5782) -> (double precision float=w5773:dbl[])
        n1317 = To Double Precision Float(number=w5781) -> (double precision float=w5771:dbl[])
        n1318 = To Double Precision Float(number=w5780) -> (double precision float=w5769:dbl[])
        n1319 = To Double Precision Float(number=w5779) -> (double precision float=w5767:dbl[])
        n1320 = To Double Precision Float(number=w5778) -> (double precision float=w5765:dbl[])
        n1321 = To Double Precision Float(number=w5777) -> (double precision float=w5763:dbl[])
        n1322 = To Double Precision Float(number=w5776) -> (double precision float=w5761:dbl[])
        n1323 = To Double Precision Float(number=w5775) -> (double precision float=w5759:dbl[])
        n1324 = Interleave 1D Arrays(w5773, w5771, w5769, w5767, w5765, w5763, w5761, w5759) -> (w5758:dbl[])
      }
    }
    n1325 = local read "FPGA Ave."() -> (w4594:dbl)
    n1326 = feedback #4(i16 -1 ("Trap Sets")) -> (w4592:i16)
    n1327 = feedback #5("" ("Detector Type")) -> (w4589:string)
    n1328 = Not Equal?(x=w4589, y="Detector Type") -> (x != y?=w4587:bool)
    n1329 = local read "Trap Sets"() -> (w4591:i16)
    n1330 = Not Equal?(x=w4592, y=w4591) -> (x != y?=w4586:bool)
    n1331 = Or(x=w4587, y=w4586) -> (x .or. y?=w4585:bool)
    n1332 = Divide(x=w4711, y=w4594) -> (x/y=w4719:dbl[])
    n1333 = case "Deinterlace trap data, average down PSD" shown="2" w4591 {
      tunnel: w4719 -> [w5802 w5867]
      tunnel: [w5799 w5864] -> w4579
      tunnel: [w5802 w5866] -> w4718
      tunnel: "Detector Type" -> [w5801 w5862]
      tunnel: [w5800 w5865] -> w4577
      tunnel: [w5798 w5863] -> w4710
      frame #0 {
        n1334 = Divide(x=w5802, y=3276.7) -> (x/y=w5803:dbl[])
        n1335 = Decimate 1D Array(w5803) -> (w5812:dbl[], w5811:dbl[], w5810:dbl[], w5809:dbl[], w5808:dbl[], w5807:dbl[], w5806:dbl[], w5805:dbl[])
        n1336 = case shown="\"IR-QPD + PSD + FB-QPD position\"" w5801 {
          tunnel: w5812 -> [w5836 w5861]
          tunnel: w5811 -> [w5835 w5860]
          tunnel: w5810 -> [w5820 w5838]
          tunnel: w5809 -> [w5821 w5848]
          tunnel: w5808 -> [w5834 w5859]
          tunnel: w5807 -> [w5833 w5858]
          tunnel: w5806 -> [w5817 w5839]
          tunnel: w5805 -> [w5816 w5837]
          tunnel: [w5815 w5845] -> w5800
          tunnel: [w5814 w5844] -> w5799
          tunnel: [w5813 w5843] -> w5798
          frame #0 {
            w5813 = 0  # Channel pattern
            n1337 = Divide(x=w5836, y=w5821) -> (x/y=w5823:dbl[])
            n1338 = Divide(x=w5835, y=w5821) -> (x/y=w5822:dbl[])
            n1339 = Divide(x=w5834, y=w5817) -> (x/y=w5819:dbl[])
            n1340 = Divide(x=w5833, y=w5816) -> (x/y=w5818:dbl[])
            n1341 = Build Array(w5823, w5822, w5821, w5820, w5819, w5818, w5817, w5816) -> (w5814:dbl[][])
            n1342 = Bundle("T1 Y", "T1 X", "T1 Sum", "FB Sum", "PSD Y", "PSD X", "PSD Y Sum", "PSD X Sum") -> (w5832:T37)  [unwired: 1 out]
            n1343 = Cluster To Array(cluster=w5832) -> (array=w5815:string[])
          }
          frame #1 {
            w5843 = 3  # Channel pattern
            n1344 = Negate(x=w5839) -> (-x=w5840:dbl[])
            n1345 = Divide(x=w5861, y=w5848) -> (x/y=w5850:dbl[])
            n1346 = Divide(x=w5860, y=w5848) -> (x/y=w5849:dbl[])
            n1347 = Divide(x=w5859, y=w5839) -> (x/y=w5847:dbl[])
            n1348 = Divide(x=w5858, y=w5840) -> (x/y=w5846:dbl[])
            n1349 = Build Array(w5850, w5849, w5848, w5837, w5838, w5847, w5846, w5839) -> (w5844:dbl[][])
            n1350 = Bundle("T1 Y", "T1 X", "T1 Sum", "FB X", "FB Sum", "PSD Y", "PSD X", "PSD Y Sum") -> (w5857:T37)  [unwired: 1 out]
            n1351 = Cluster To Array(cluster=w5857) -> (array=w5845:string[])
          }
        }
      }
      frame #1 {
        n1352 = case shown="\"IR-QPD + PSD + FB-QPD X position\"" w5862 {
          tunnel: w5867 -> [w5928 w5995 w6065]
          tunnel: [w5908 w5980 w6052] -> w5866
          tunnel: [w5894 w5971 w6043] -> w5865
          tunnel: [w5893 w5931 w6010] -> w5864
          tunnel: [w5887 w5969 w6041] -> w5863
          frame #0 {
            w5887 = 1  # Channel pattern
            # "time average x2 the 4th signal and the 4 psd signals (detection laser)"
            # "deinterlace 3 signals from qpd"
            n1353 = Decimate 1D Array(w5928) -> (w5927:dbl[], w5926:dbl[], w5892:dbl[], w5925:dbl[], w5915:dbl[], w5913:dbl[], w5912:dbl[], w5910:dbl[])
            n1354 = Decimate 1D Array(w5892) -> (w5891:dbl[], w5890:dbl[])
            n1355 = Decimate 1D Array(w5927) -> (w5924:dbl[], w5896:dbl[])
            n1356 = Decimate 1D Array(w5926) -> (w5923:dbl[], w5921:dbl[])
            n1357 = Decimate 1D Array(w5925) -> (w5922:dbl[], w5920:dbl[])
            n1358 = call "downsample 1D array - double.vi"("Ave N"=2.0, "Array In"=w5915) -> ("Array Out"=w5914:dbl[])  [unwired: 1 out]
            n1359 = call "downsample 1D array - double.vi"("Ave N"=2.0, "Array In"=w5913) -> ("Array Out"=w5895:dbl[])  [unwired: 1 out]
            n1360 = call "downsample 1D array - double.vi"("Ave N"=2.0, "Array In"=w5912) -> ("Array Out"=w5911:dbl[])  [unwired: 1 out]
            n1361 = call "downsample 1D array - double.vi"("Ave N"=2.0, "Array In"=w5910) -> ("Array Out"=w5909:dbl[])  [unwired: 1 out]
            n1362 = Interleave 1D Arrays(w5924, w5923, w5922, w5896, w5921, w5920, w5891, w5890, w5914, w5895, w5911, w5909) -> (w5908:dbl[])
            n1363 = Divide(x=w5908, y=3276.7) -> (x/y=w5907:dbl[])
            n1364 = Decimate 1D Array(w5907) -> (w5906:dbl[], w5905:dbl[], w5904:dbl[], w5903:dbl[], w5902:dbl[], w5901:dbl[], w5889:dbl[], w5888:dbl[], w5900:dbl[], w5899:dbl[], w5898:dbl[], w5897:dbl[])
            n1365 = Divide(x=w5906, y=w5904) -> (x/y=w5874:dbl[])
            n1366 = Divide(x=w5905, y=w5904) -> (x/y=w5873:dbl[])
            n1367 = Divide(x=w5903, y=w5901) -> (x/y=w5872:dbl[])
            n1368 = Divide(x=w5902, y=w5901) -> (x/y=w5871:dbl[])
            n1369 = Divide(x=w5900, y=w5898) -> (x/y=w5870:dbl[])
            n1370 = Divide(x=w5899, y=w5897) -> (x/y=w5869:dbl[])
            n1371 = Build Array(w5874, w5873, w5904, w5872, w5871, w5901, w5889, w5888, w5870, w5869, w5898, w5897) -> (w5893:dbl[][])
            n1372 = Bundle("T1 Y", "T1 X", "T1 Sum", "T2 Y", "T2 X", "T2 Sum", "T1 FB Sum", "T2 FB Sum", "PSD Y", "PSD X", "PSD Y Sum", "PSD X Sum") -> (w5875:T38)  [unwired: 1 out]
            n1373 = Cluster To Array(cluster=w5875) -> (array=w5894:string[])
          }
          frame #1 {
            w5969 = 2  # Channel pattern
            # "time average x2 the 3 psd signals (detection laser)"
            # "deinterlace 3 signals from qpds"
            n1374 = Decimate 1D Array(w5995) -> (w5994:dbl[], w5993:dbl[], w5970:dbl[], w5992:dbl[], w5983:dbl[], w5982:dbl[], w5981:dbl[], w5957:dbl[])
            n1375 = Decimate 1D Array(w5970) -> (w5952:dbl[], w5950:dbl[])
            n1376 = Decimate 1D Array(w5994) -> (w5991:dbl[], w5972:dbl[])
            n1377 = Decimate 1D Array(w5993) -> (w5990:dbl[], w5988:dbl[])
            n1378 = Decimate 1D Array(w5992) -> (w5989:dbl[], w5987:dbl[])
            n1379 = Decimate 1D Array(w5957) -> (w5953:dbl[], w5951:dbl[])
            n1380 = call "downsample 1D array - double.vi"("Ave N"=2.0, "Array In"=w5983) -> ("Array Out"=w5956:dbl[])  [unwired: 1 out]
            n1381 = call "downsample 1D array - double.vi"("Ave N"=2.0, "Array In"=w5982) -> ("Array Out"=w5955:dbl[])  [unwired: 1 out]
            n1382 = call "downsample 1D array - double.vi"("Ave N"=2.0, "Array In"=w5981) -> ("Array Out"=w5954:dbl[])  [unwired: 1 out]
            n1383 = Interleave 1D Arrays(w5991, w5990, w5989, w5972, w5988, w5987, w5953, w5952, w5951, w5950, w5956, w5955, w5954) -> (w5980:dbl[])
            n1384 = Divide(x=w5980, y=3276.7) -> (x/y=w5979:dbl[])
            n1385 = Decimate 1D Array(w5979) -> (w5978:dbl[], w5977:dbl[], w5976:dbl[], w5975:dbl[], w5974:dbl[], w5973:dbl[], w5942:dbl[], w5940:dbl[], w5939:dbl[], w5937:dbl[], w5936:dbl[], w5935:dbl[], w5932:dbl[])
            n1386 = Negate(x=w5932) -> (-x=w5930:dbl[])
            n1387 = Divide(x=w5936, y=w5932) -> (x/y=w5934:dbl[])
            n1388 = Divide(x=w5935, y=w5930) -> (x/y=w5933:dbl[])
            n1389 = Divide(x=w5978, y=w5976) -> (x/y=w5961:dbl[])
            n1390 = Divide(x=w5977, y=w5976) -> (x/y=w5960:dbl[])
            n1391 = Divide(x=w5975, y=w5973) -> (x/y=w5959:dbl[])
            n1392 = Divide(x=w5974, y=w5973) -> (x/y=w5958:dbl[])
            n1393 = Divide(x=w5942, y=w5940) -> (x/y=w5941:dbl[])
            n1394 = Divide(x=w5939, y=w5937) -> (x/y=w5938:dbl[])
            n1395 = Build Array(w5961, w5960, w5976, w5959, w5958, w5973, w5941, w5940, w5938, w5937, w5934, w5933, w5932) -> (w5931:dbl[][])
            n1396 = Bundle("T1 Y", "T1 X", "T1 Sum", "T2 Y", "T2 X", "T2 Sum", "T1 FB X", "T1 FB Sum", "T2 FB X", "T2 FB Sum", "PSD Y", "PSD X", "PSD Y Sum") -> (w5962:T39)  [unwired: 1 out]
            n1397 = Cluster To Array(cluster=w5962) -> (array=w5971:string[])
          }
          frame #2 {
            w6041 = 4  # Channel pattern
            # "time average x2 the 3 psd signals (detection laser)"
            # "deinterlace 3 signals from qpds"
            n1398 = Decimate 1D Array(w6065) -> (w6064:dbl[], w6063:dbl[], w6042:dbl[], w6062:dbl[], w6008:dbl[], w6054:dbl[], w6053:dbl[], w6030:dbl[])
            n1399 = Decimate 1D Array "Feedback Sum"(w6042) -> (w6026:dbl[], w6024:dbl[])
            n1400 = Decimate 1D Array "QPD Y"(w6064) -> (w6061:dbl[], w6044:dbl[])
            n1401 = Decimate 1D Array "QPD X"(w6063) -> (w6060:dbl[], w6058:dbl[])
            n1402 = Decimate 1D Array "Feedback Y"(w6008) -> (w6007:dbl[], w6006:dbl[])
            n1403 = Decimate 1D Array "QPD Sum"(w6062) -> (w6059:dbl[], w6057:dbl[])
            n1404 = Decimate 1D Array "Feedback X"(w6030) -> (w6027:dbl[], w6025:dbl[])
            n1405 = call "downsample 1D array - double.vi"("Ave N"=2.0, "Array In"=w6054) -> ("Array Out"=w6029:dbl[])  [unwired: 1 out]
            n1406 = call "downsample 1D array - double.vi"("Ave N"=2.0, "Array In"=w6053) -> ("Array Out"=w6028:dbl[])  [unwired: 1 out]
            n1407 = Interleave 1D Arrays(w6061, w6060, w6059, w6044, w6058, w6057, w6007, w6027, w6026, w6006, w6025, w6024, w6029, w6028) -> (w6052:dbl[])
            n1408 = Divide(x=w6052, y=3276.7) -> (x/y=w6051:dbl[])
            n1409 = Decimate 1D Array(w6051) -> (w6050:dbl[], w6049:dbl[], w6048:dbl[], w6047:dbl[], w6046:dbl[], w6045:dbl[], w6003:dbl[], w6017:dbl[], w6001:dbl[], w6002:dbl[], w6015:dbl[], w5999:dbl[], w6013:dbl[], w6011:dbl[])
            n1410 = Negate(x=w6011) -> (-x=w6009:dbl[])
            n1411 = Divide(x=w6013, y=w6009) -> (x/y=w6012:dbl[])
            n1412 = Divide(x=w6002, y=w5999) -> (x/y=w5998:dbl[])
            n1413 = Divide(x=w6003, y=w6001) -> (x/y=w6000:dbl[])
            n1414 = Divide(x=w6050, y=w6048) -> (x/y=w6034:dbl[])
            n1415 = Divide(x=w6049, y=w6048) -> (x/y=w6033:dbl[])
            n1416 = Divide(x=w6047, y=w6045) -> (x/y=w6032:dbl[])
            n1417 = Divide(x=w6046, y=w6045) -> (x/y=w6031:dbl[])
            n1418 = Divide(x=w6017, y=w6001) -> (x/y=w6016:dbl[])
            n1419 = Divide(x=w6015, y=w5999) -> (x/y=w6014:dbl[])
            n1420 = Build Array(w6034, w6033, w6048, w6032, w6031, w6045, w6000, w6016, w6001, w5998, w6014, w5999, w6012, w6011) -> (w6010:dbl[][])
            n1421 = Bundle("T1 Y", "T1 X", "T1 Sum", "T2 Y", "T2 X", "T2 Sum", "T1 FB Y", "T1 FB X", "T1 FB Sum", "T2 FB Y", "T2 FB X", "T2 FB Sum", "PSD X", "PSD Y Sum") -> (w5997:T40)  [unwired: 1 out]
            n1422 = Cluster To Array(cluster=w5997) -> (array=w6043:string[])
          }
        }
      }
    }
    n1423 = case "Update these things only if detector type or number of traps changes" shown="True" w4585 {
      tunnel: w4577 -> [_ w4870]
      frame #0 {
      }
      frame #1 {
        n1424 = property on="High Res. Display" class="Ring (strict)"("Strings []"=w4870) -> ()  [unwired: 2 in, 2 out]
        n1425 = Build Array (concatenate)(w4870, "none") -> (w4863:string[])
        n1426 = property on="FFT 1 Choice 1" class="Ring (strict)"("Strings []"=w4863) -> ()  [unwired: 2 in, 2 out]
        n1427 = property on="FFT 1 Choice 2" class="Ring (strict)"("Strings []"=w4863) -> ()  [unwired: 2 in, 2 out]
        n1428 = property on="FFT 2 Choice 1" class="Ring (strict)"("Strings []"=w4863) -> ()  [unwired: 2 in, 2 out]
        n1429 = property on="FFT 2 Choice 2" class="Ring (strict)"("Strings []"=w4863) -> ()  [unwired: 2 in, 2 out]
        n1430 = Bundle("APD 1", "APD 2") -> (w4866:cluster{string, string})  [unwired: 1 out]
        n1431 = Cluster To Array(cluster=w4866) -> (array=w4864:string[])
        n1432 = Build Array (concatenate)(w4864, w4863) -> (w4868:string[])
        n1433 = Array Size(array=w4868) -> (size(s)=w4869:i32)
        n1434 = property on="Signals to Plot" class="LstBox (strict)"("Item Names"=w4868) -> ()  [unwired: 2 in, 2 out]
        n1435 = property on="Signals to Plot" class="LstBox (strict)"("Number of Rows"=w4869) -> ()  [unwired: 2 in, 2 out]
        n1436 = property on="All Signals" class="WFChart (strict)"("LegNumRows"=w4869) -> ()  [unwired: 2 in, 2 out]
      }
    }
    n1437 = local read "Data points/scans (MCL)"() -> (w4681:dbl)
    n1438 = Increment(x=w4681) -> (x+1=w4682:dbl)
    n1439 = feedback #6(w4682) -> (w4685:dbl)
    n1440 = Select(t=0, s=w4672, f=w4685) -> (s? t:f=w4678:dbl)
    n1441 = To Word Integer(number=w4718) -> (16bit integer=w4745:i16[])
    n1442 = Decimate 1D Array(w4540) -> (w4571:u32[], w4708:u32[])
    n1443 = To Double Precision Float(number=w4571) -> (double precision float=w4570:dbl[])
    n1444 = Array Size(array=w4570) -> (size(s)=w4684:i32)
    n1445 = Add(x=w4684, y=w4678) -> (x+y=w4679:dbl)
    n1446 = Greater?(x=w4679, y=w4681) -> (0:w4680:bool)
    n1447 = local read "DMA Update Period (s)"() -> (w4598:dbl)
    n1448 = Select(t=w4678, s=w4680, f=w4679) -> (s? t:f=w4677:dbl)
    n1449 = Build Array(w4571, w4708) -> (w4669:u32[][])
    n1450 = local read "MCL Scanning"() -> (w4675:bool)
    n1451 = local read "Data Period (s)"() -> (w4556:dbl)
    n1452 = To Double Precision Float(number=w4669) -> (double precision float=w4670:dbl[][])
    n1453 = Not(x=w4680) -> (.not. x?=w4674:bool)
    n1454 = local read "APD Integration Time (s)"() -> (w4597:dbl)
    n1455 = And(x=w4674, y=w4675) -> (x .and. y?=w4676:bool)
    n1456 = feedback #7(0.0) -> (w4705:dbl)
    n1457 = Add(x=w4598, y=w4705) -> (x+y=w4714:dbl)
    n1458 = Or(x=w4676, y=w4672) -> (x .or. y?=w4673:bool)
    n1459 = Multiply(x=w4556, y="Trap Disp. Downsample") -> (x*y=w4554:dbl)
    "Display Period (s)" <- w4554
    n1460 = Equal?(x="Tab Control 6", y=T30."High Res Display") -> (x = y?=w4582:bool)
    n1461 = for {
      tunnel: [w5797] -> w4704 mode=indexing
      tunnel: w4705 -> [w5796]
      tunnel: "Trap Disp. Downsample" -> [w5793]
      tunnel: w4579 -> [w5791] mode=indexing
      tunnel: w4556 -> [w5790]
      tunnel: w4577 -> [w5789] mode=indexing
      tunnel: w4578 -> [w5788]
      tunnel: [w5787] -> w4527 mode=indexing
      tunnel: w4554 -> [w5786]
      workers-P: _ -> [_]
      n1462 = Bundle By Name("Y"=w5791, "dt"=w5790) -> (w5792:waveform(dbl))  [unwired: 1 out]
      n1463 = Set Waveform Attribute(5:w5789, 6:w5788, 7:w5792) -> (3:w5787:waveform(dbl))  [unwired: 1 in, 2 out]
      n1464 = call "downsample 1D array - double.vi"("Ave N"=w5793, "Array In"=w5791) -> ("Array Out"=w5794:dbl[])  [unwired: 1 out]
      n1465 = To Time Stamp(1:w5796) -> (0:w5795:timestamp)
      n1466 = Bundle By Name(cluster=w5787, "t0"=w5795, "Y"=w5794, "dt"=w5786) -> (w5797:waveform(dbl))
    }
    n1467 = case "For plotting results of scanning MCL" shown="True" w4673 {
      tunnel: w4672 -> [_ w5320]
      tunnel: w4570 -> [_ w5333]
      tunnel: w4681 -> [_ _]
      tunnel: w4527 -> [_ w5304]
      tunnel: w4528 -> [_ w5236]
      tunnel: w4526 -> [_ w5234]
      tunnel: w4525 -> [_ w5233]
      frame #0 {
      }
      frame #1 {
        w5241 = u32 0 items=["Horizontal", "Vertical", "Central", "1st Diagonal", "2nd Diagonal"] ("Type of Symmetry")
        w5244 = u32 0 items=["Horizontal", "Vertical", "Central", "1st Diagonal", "2nd Diagonal"] ("Type of Symmetry")
        w5274 = u32 0 items=["Horizontal", "Vertical", "Central", "1st Diagonal", "2nd Diagonal"] ("Type of Symmetry")
        n1468 = Index Array(array=w5304, index=10) -> (element=w5310:waveform(dbl))
        n1469 = Index Array(array=w5304, index=11) -> (element=w5307:waveform(dbl))
        n1470 = Index Array(array=w5304, index="Channel") -> (element=w5306:waveform(dbl))
        n1471 = local read "Cycles/step (MCL)"() -> (w5258:u64)
        n1472 = Unbundle By Name(w5310) -> ("Y"=w5260:dbl[])
        n1473 = Unbundle By Name(w5307) -> ("Y"=w5262:dbl[])
        n1474 = Unbundle By Name(w5306) -> ("Y"=w5267:dbl[])
        n1475 = call "downsample 1D array - double.vi"("Ave N"=w5258, "Array In"=w5260) -> ("Array Out"=w5259:dbl[])  [unwired: 1 out]
        n1476 = call "downsample 1D array - double.vi"("Ave N"=w5258, "Array In"=w5262) -> ("Array Out"=w5261:dbl[])  [unwired: 1 out]
        n1477 = call "downsample 1D array - double.vi"("Ave N"=w5258, "Array In"=w5267) -> ("Array Out"=w5266:dbl[])  [unwired: 1 out]
        n1478 = feedback #8(w5333) -> (w5334:dbl[])
        n1479 = Build Array (concatenate)(w5334, w5333) -> (w5312:dbl[])
        n1480 = Select(t=w5333, s=w5320, f=w5312) -> (s? t:f=w5317:dbl[])
        n1481 = feedback #9(w5259) -> (w5321:dbl[])
        n1482 = Build Array (concatenate)(w5321, w5259) -> (w5309:dbl[])
        n1483 = feedback #10(w5266) -> (w5331:dbl[])
        n1484 = Build Array (concatenate)(w5331, w5266) -> (w5330:dbl[])
        n1485 = feedback #11(w5261) -> (w5323:dbl[])
        n1486 = Build Array (concatenate)(w5323, w5261) -> (w5324:dbl[])
        n1487 = Select(t=w5259, s=w5320, f=w5309) -> (s? t:f=w5263:dbl[])
        n1488 = Select(t=w5266, s=w5320, f=w5330) -> (s? t:f=w5265:dbl[])
        n1489 = Select(t=w5261, s=w5320, f=w5324) -> (s? t:f=w5264:dbl[])
        n1490 = local read "N APD Samp/step"() -> (w5316:dbl)
        n1491 = local read "Scan steps (MCL)"() -> (w5271:u64)
        n1492 = local read "Scan lines (y)"() -> (w5303:u64)
        n1493 = call "integrate 1D array interval - double.vi"("Ave N"=w5316, "Array In"=w5317) -> ("Array Out"=w5315:dbl[])  [unwired: 1 out]
        n1494 = Array Size(array=w5315) -> (size(s)=w5319:i32)
        n1495 = Multiply(x=w5271, y=u64 2) -> (x*y=w5318:u64)
        n1496 = Multiply(x=w5303, y=w5318) -> (x*y=w5328:u64)
        n1497 = Subtract(x=w5328, y=w5319) -> (x-y=w5257:u64)
        n1498 = call <vilib>:"Mean.vi"("X"=w5315) -> ("mean"=w5254:dbl)  [unwired: 1 out]
        n1499 = call <vilib>:"Mean.vi"("X"=w5263) -> ("mean"=w5247:dbl)  [unwired: 1 out]
        n1500 = call <vilib>:"Mean.vi"("X"=w5265) -> ("mean"=w5252:dbl)  [unwired: 1 out]
        n1501 = call <vilib>:"Mean.vi"("X"=w5264) -> ("mean"=w5250:dbl)  [unwired: 1 out]
        n1502 = Initialize Array(1.0 ("element"), w5257) -> (w5248:dbl[])
        n1503 = Multiply(x=w5248, y=w5254) -> (x*y=w5255:dbl[])
        n1504 = Multiply(x=w5248, y=w5250) -> (x*y=w5251:dbl[])
        n1505 = Multiply(x=w5248, y=w5252) -> (x*y=w5253:dbl[])
        n1506 = Multiply(x=w5248, y=w5247) -> (x*y=w5249:dbl[])
        n1507 = Build Array (concatenate)(w5315, w5255) -> (w5327:dbl[])
        n1508 = Build Array (concatenate)(w5263, w5249) -> (w5322:dbl[])
        n1509 = Build Array (concatenate)(w5265, w5253) -> (w5326:dbl[])
        n1510 = Build Array (concatenate)(w5264, w5251) -> (w5325:dbl[])
        n1511 = Reshape Array(w5327, w5303, w5318) -> (w5301:dbl[][])
        n1512 = Reshape Array(w5322, w5303, w5318) -> (w5284:dbl[][])
        n1513 = Reshape Array(w5326, w5303, w5318) -> (w5276:dbl[][])
        n1514 = Reshape Array(w5325, w5303, w5318) -> (w5291:dbl[][])
        n1515 = Index Array(array=w5301, index (row)=0) -> (element=→"Waveform Graph":dbl[])  [unwired: 1 in]
        n1516 = Array Subset(array=w5291, index (col)=0 ("index"), length (col)=w5271) -> (w5296:dbl[][])  [unwired: 2 in]
        n1517 = Array Subset(array=w5301, index (col)=0 ("index"), length (col)=w5271) -> (w5300:dbl[][])  [unwired: 2 in]
        n1518 = Array Subset(array=w5291, index (col)=w5271) -> (w5294:dbl[][])  [unwired: 3 in]
        n1519 = Array Subset(array=w5301, index (col)=w5271) -> (w5298:dbl[][])  [unwired: 3 in]
        n1520 = Array Subset(array=w5276, index (col)=0 ("index"), length (col)=w5271) -> (w5282:dbl[][])  [unwired: 2 in]
        n1521 = Array Subset(array=w5276, index (col)=w5271) -> (w5280:dbl[][])  [unwired: 3 in]
        n1522 = Array Subset(array=w5284, index (col)=0 ("index"), length (col)=w5271) -> (w5289:dbl[][])  [unwired: 2 in]
        n1523 = Array Subset(array=w5284, index (col)=w5271) -> (w5287:dbl[][])  [unwired: 3 in]
        n1524 = for {
          tunnel: w5296 -> [w5340] mode=indexing
          tunnel: [w5339] -> w5295 mode=indexing
          workers-P: _ -> [_]
          n1525 = Reverse 1D Array(array=w5340) -> (reversed array=w5339:dbl[])
        }
        n1526 = for {
          tunnel: w5300 -> [w5342] mode=indexing
          tunnel: [w5341] -> w5299 mode=indexing
          workers-P: _ -> [_]
          n1527 = Reverse 1D Array(array=w5342) -> (reversed array=w5341:dbl[])
        }
        n1528 = for {
          tunnel: w5282 -> [w5336] mode=indexing
          tunnel: [w5335] -> w5281 mode=indexing
          workers-P: _ -> [_]
          n1529 = Reverse 1D Array(array=w5336) -> (reversed array=w5335:dbl[])
        }
        n1530 = for {
          tunnel: w5289 -> [w5338] mode=indexing
          tunnel: [w5337] -> w5288 mode=indexing
          workers-P: _ -> [_]
          n1531 = Reverse 1D Array(array=w5338) -> (reversed array=w5337:dbl[])
        }
        n1532 = Add(x=w5295, y=w5294) -> (x+y=w5293:dbl[][])
        n1533 = Add(x=w5299, y=w5298) -> (x+y=w5273:dbl[][])
        n1534 = Add(x=w5281, y=w5280) -> (x+y=w5279:dbl[][])
        n1535 = Add(x=w5288, y=w5287) -> (x+y=w5286:dbl[][])
        n1536 = Divide(x=w5279, y=2) -> (x/y=w5277:dbl[][])
        n1537 = Divide(x=w5293, y=2) -> (x/y=w5237:dbl[][])
        n1538 = To Single Precision Float(number=w5273) -> (single precision float=w5272:sgl[][])
        n1539 = Divide(x=w5286, y=2) -> (x/y=w5239:dbl[][])
        n1540 = Transpose 2D Array(2D array=w5277) -> (transposed array=→"Data map":dbl[][])
        n1541 = To Single Precision Float(number=w5237) -> (single precision float=w5243:sgl[][])
        n1542 = To Single Precision Float(number=w5239) -> (single precision float=w5240:sgl[][])
        n1543 = call "IMAQ ArrayToImage"("Image Pixels (Float)"=w5272, "Image"=w5236) -> ("Image Out"=w5275:T1)  [unwired: 8 in, 1 out]
        n1544 = call "IMAQ ArrayToImage"("Image Pixels (Float)"=w5243, "Image"=w5234) -> ("Image Out"=w5245:T1)  [unwired: 8 in, 1 out]
        n1545 = call "IMAQ Symmetry"("Type of Symmetry"=w5274, "Image Src"=w5275) -> ("Image Dst Out"=w5269:T1)  [unwired: 3 in, 1 out]
        n1546 = call "IMAQ ArrayToImage"("Image Pixels (Float)"=w5240, "Image"=w5233) -> ("Image Out"=w5242:T1)  [unwired: 8 in, 1 out]
        n1547 = call "IMAQ Symmetry"("Type of Symmetry"=w5244, "Image Src"=w5245) -> ("Image Dst Out"=→"Detection Laser X":T1)  [unwired: 3 in, 1 out]
        n1548 = call "IMAQ Symmetry"("Type of Symmetry"=w5241, "Image Src"=w5242) -> ("Image Dst Out"=→"Detection Laser Y":T1)  [unwired: 3 in, 1 out]
        n1549 = call "IMAQ Set Simple Calibration"("Calibration Axis Info"=T31 {"Origin Pixel"={"X"=0.0, "Y"=0.0}, "Angle Relative to Horizontal (deg)"=0.0, "Axis Reference"=0}, "Grid Descriptor"=T32 {"X Step"=0.3, "Y Step"=0.3, "Unit"=enum."Undefined"}, "Image"=w5269) -> ("Calibrated Image"=→"APD 1":T1)  [unwired: 7 in, 1 out]
      }
    }
    n1550 = Reciprocal(x=w4554) -> (1/x=→"Trap Disp. Freq. (Hz)":dbl)
    n1551 = case shown="True" w4582 {
      tunnel: w4527 -> [_ w4839]
      frame #0 {
      }
      frame #1 {
        n1552 = Index Array(array=w4839, index="High Res. Display") -> (element=w4840:waveform(dbl))
        n1553 = call <vilib>:"Std Deviation and Variance.vi"("X"=w4840) -> ("mean"=w4847:dbl, "standard deviation"=w4852:dbl)  [unwired: 1 in, 1 out]
        "Mean Intensity" <- w4847
        "Sigma" <- w4852
        n1554 = Subtract(x=w4840, y=w4847) -> (x-y=w4846:waveform(dbl))
        n1555 = Select(t=w4846, s="Subtract mean", f=w4840) -> (s? t:f=→"1 Channel":waveform(dbl))
        n1556 = Divide(x=w4852, y=w4847) -> (x/y=→"Sigma/Mean":dbl)
        n1557 = feedback #12(1) -> (w4841:i32)
        n1558 = Greater Or Equal?(x=w4841, y="Slow mean N ave.") -> (x >= y?=w4854:bool)
        n1559 = Increment(x=w4841) -> (x+1=w4856:i32)
        n1560 = Select(t=1, s=w4854, f=w4856) -> (s? t:f=w4843:i32)
        n1561 = feedback #13() -> (w4844:waveform(dbl))  [unwired: 1 out]
        n1562 = case shown="Default" w4841 {
          tunnel: [w4859 w4862] -> w4845
          tunnel: w4844 -> [w4861 _]
          tunnel: w4840 -> [w4860 w4862]
          frame #0 {
            n1563 = call-poly <vilib>:"Append Waveforms.vi"("waveform B"=w4860, "waveform A"=w4861) -> ("waveform out"=w4859:waveform(dbl))  [unwired: 1 in, 8 out]
          }
          frame #1 {
          }
        }
        n1564 = case shown="True" w4854 {
          tunnel: w4845 -> [_ w4858]
          frame #0 {
          }
          frame #1 {
            n1565 = call <vilib>:"Mean.vi"("X"=w4858) -> ("mean"=→"Slow mean":dbl)  [unwired: 1 out]
          }
        }
      }
    }
    n1566 = case "For computing FFTs for display" shown="True" "Compute FFT" {
      tunnel: w4527 -> [_ w6682]
      frame #0 {
      }
      frame #1 {
        n1567 = Build Array("FFT 1 Choice 1", "FFT 1 Choice 2", "FFT 2 Choice 1", "FFT 2 Choice 2") -> (w6675:u16[])
        n1568 = Array Size(array=w6682) -> (size(s)=w6681:i32)
        n1569 = feedback #14(u16[] [100, 100, 100, 100]) -> (w6676:u16[])
        n1570 = feedback #15("# Spectra to Ave.") -> (w6673:dbl)
        n1571 = Not Equal?(x="# Spectra to Ave.", y=w6673) -> (x != y?=w6672:bool)
        n1572 = Not Equal?(x=w6675, y=w6676) -> (x != y?=w6674:bool)
        n1573 = feedback #16(1.0) -> (w6659:dbl)
        n1574 = Compound Arithmetic op=OR("Reset FFT", w6674, w6672) -> (w6657:bool)
        n1575 = Select(t=1.0, s=w6657, f=w6659) -> (s? t:f=w6661:dbl)
        n1576 = Greater?(x=w6661, y="# Spectra to Ave.") -> (0:w6680:bool)
        n1577 = Increment(x=w6661) -> (x+1=w6660:dbl)
        n1578 = local read "DMA Update Period (s)"() -> (w6655:dbl)
        n1579 = Multiply(x="# Spectra to Ave.", y=w6655) -> (x*y=→"Ave. Time (s)":dbl)
        n1580 = Build Array(cluster{"f0":dbl, "df":dbl, "magnitude":dbl[]} {"f0"=0.0, "df"=0.0, "magnitude"=[]} ("PSD")) -> (w6664:cluster{"f0":dbl, "df":dbl, "magnitude":dbl[]}[])
        n1581 = Build Array(w6664, w6664, w6664, w6664) -> (w6666:T41)
        n1582 = feedback #17(w6666) -> (w6671:T41)
        n1583 = for {
          N: 4 -> [_]
          tunnel: w6675 -> [w6704] mode=indexing
          tunnel: w6682 -> [w6705]
          tunnel: w6681 -> [w6707]
          tunnel: w6657 -> [w6700]
          tunnel: w6680 -> [w6699]
          tunnel: "# Spectra to Ave." -> [w6698]
          tunnel: [w6697] -> w6670 mode=indexing
          tunnel: w6671 -> [w6702] mode=indexing
          tunnel: [w6701] -> w6658 mode=indexing
          tunnel: w6661 -> [w6696]
          n1584 = Less?(x=w6704, y=w6707) -> (x < y?=w6706:bool)
          n1585 = Index Array(array=w6705, index=w6704) -> (element=w6703:waveform(dbl))
          n1586 = case shown="True" w6706 {
            tunnel: w6703 -> [_ w6724]
            tunnel: w6702 -> [w6709 w6722]
            tunnel: [w6709 w6710] -> w6701
            tunnel: w6700 -> [_ w6721]
            tunnel: w6699 -> [_ w6714]
            tunnel: w6698 -> [_ w6713]
            tunnel: [cluster{"f0":dbl, "df":dbl, "magnitude":dbl[]} {"f0"=0.0, "df"=0.0, "magnitude"=[]} ("PSD") w6715] -> w6697
            tunnel: w6696 -> [_ w6712]
            frame #0 {
            }
            frame #1 {
              n1587 = call <vilib>:"Std Deviation and Variance.vi"("X"=w6724) -> ("mean"=w6725:dbl)  [unwired: 1 in, 2 out]
              n1588 = Subtract(x=w6724, y=w6725) -> (x-y=w6723:waveform(dbl))
              n1589 = xnode "Spectral Measurements"("Signals"=w6723) -> ("PSD"=w6717:cluster{"f0":dbl, "df":dbl, "magnitude":dbl[]})  [unwired: 1 in, 1 out]
              n1590 = case shown="False" w6721 {
                tunnel: w6722 -> [w6734 _]
                tunnel: [w6730 w6739] -> w6710
                tunnel: w6717 -> [w6733 w6740]
                tunnel: w6714 -> [w6732 _]
                frame #0 {
                  n1591 = Build Array (concatenate)(w6734, w6733) -> (w6731:cluster{"f0":dbl, "df":dbl, "magnitude":dbl[]}[])
                  n1592 = case shown="True" w6732 {
                    tunnel: w6731 -> [w6735 w6738]
                    tunnel: [w6735 w6736] -> w6730
                    frame #0 {
                    }
                    frame #1 {
                      n1593 = Delete From Array(array=w6738, index=0) -> (array with subset deleted=w6736:cluster{"f0":dbl, "df":dbl, "magnitude":dbl[]}[])  [unwired: 1 in, 1 out]
                    }
                  }
                }
                frame #1 {
                  n1594 = Build Array(w6740) -> (w6739:cluster{"f0":dbl, "df":dbl, "magnitude":dbl[]}[])
                }
              }
              n1595 = for {
                tunnel: w6710 -> [w6729] mode=indexing
                tunnel: [w6728] -> w6720 mode=indexing
                workers-P: _ -> [_]
                n1596 = Unbundle By Name(w6729) -> ("magnitude"=w6728:dbl[])
              }
              n1597 = Transpose 2D Array(2D array=w6720) -> (transposed array=w6719:dbl[][])
              n1598 = for {
                tunnel: w6719 -> [w6727] mode=indexing
                tunnel: [w6726] -> w6718 mode=indexing
                workers-P: _ -> [_]
                n1599 = Add Array Elements(numeric array=w6727) -> (sum=w6726:dbl)
              }
              n1600 = Select(t=w6713, s=w6714, f=w6712) -> (s? t:f=w6711:dbl)
              n1601 = Divide(x=w6718, y=w6711) -> (x/y=w6716:dbl[])
              n1602 = Bundle By Name(cluster=w6717, "magnitude"=w6716) -> (w6715:cluster{"f0":dbl, "df":dbl, "magnitude":dbl[]})
            }
          }
        }
        n1603 = case shown="True" w6657 {
          tunnel: w6658 -> [w6689 w6695]
          tunnel: [w6689 w6690] -> w6656
          frame #0 {
          }
          frame #1 {
            n1604 = Array Subset(array=w6695, index (row)=0 ("index"), length (row)=4 ("length"), index (col)=0 ("index"), length (col)=1 ("length")) -> (w6690:T41)
          }
        }
        n1605 = Split 1D Array(array=w6670, index=2) -> (first subarray=→"FFT 1":cluster{"f0":dbl, "df":dbl, "magnitude":dbl[]}[], second subarray=→"FFT 2":cluster{"f0":dbl, "df":dbl, "magnitude":dbl[]}[])
      }
    }
    n1606 = Bundle("APD 1", "APD 2") -> (w4702:cluster{string, string})  [unwired: 1 out]
    n1607 = Cluster To Array(cluster=w4702) -> (array=w4699:string[])
    n1608 = for {
      tunnel: w4670 -> [w5717] mode=indexing
      tunnel: w4705 -> [w5726]
      tunnel: w4597 -> [w5725]
      tunnel: [w5721] -> w4703 mode=indexing
      tunnel: "APD Disp. Scale" -> [w5722]
      tunnel: w4578 -> [w5720]
      tunnel: w4699 -> [w5719] mode=indexing
      tunnel: "APD Disp. Downsample" -> [w5715]
      tunnel: [w5718] -> w4698
      workers-P: _ -> [_]
      n1609 = call "integrate 1D array interval - double.vi"("Ave N"=w5715, "Array In"=w5717) -> ("Array Out"=w5716:dbl[])  [unwired: 1 out]
      n1610 = Multiply(x=w5725, y=w5715) -> (x*y=w5718:dbl)
      n1611 = Divide(x=w5716, y=w5722) -> (x/y=w5723:dbl[])
      n1612 = To Time Stamp(1:w5726) -> (0:w5727:timestamp)
      n1613 = Bundle By Name("t0"=w5727, "Y"=w5723, "dt"=w5718) -> (w5724:waveform(dbl))  [unwired: 1 out]
      n1614 = Set Waveform Attribute(5:w5719, 6:w5720, 7:w5724) -> (3:w5721:waveform(dbl))  [unwired: 1 in, 2 out]
    }
    "APD Display Period (s)" <- w4698
    n1615 = Reciprocal(x=w4698) -> (1/x=→"APD Display Freq. (Hz)":dbl)
    n1616 = feedback #18(w4571) -> (w4668:u32[])
    n1617 = Build Array (concatenate)(w4668, w4571) -> (w4665:u32[])
    n1618 = Array Size(array=w4665) -> (size(s)=w4662:i32)
    n1619 = Array Size(array=w4571) -> (size(s)=w4664:i32)
    n1620 = local read "APD Integration Time (s)"() -> (w4531:dbl)
    n1621 = Build Array (concatenate)(w4703, w4704) -> (w4523:waveform(dbl)[])
    "All Signals" <- w4523
    n1622 = Multiply(x=w4664, y="APD Ave N") -> (x*y=w4663:dbl)
    n1623 = Greater?(x=w4662, y=w4663) -> (0:w4666:bool)
    n1624 = Index Array(array=w4523, index=0) -> (element=w4655:waveform(dbl))
    n1625 = case shown="True" w4666 {
      tunnel: w4665 -> [w5227 w5232]
      tunnel: [w5227 w5228] -> w4603
      tunnel: w4663 -> [_ w5230]
      tunnel: w4662 -> [_ w5231]
      frame #0 {
      }
      frame #1 {
        n1626 = Subtract(x=w5231, y=w5230) -> (x-y=w5229:dbl)
        n1627 = Array Subset(array=w5232, index=w5229, length=w5230) -> (w5228:u32[])
      }
    }
    n1628 = Multiply(x="APD Disp. Scale", y=w4655) -> (x*y=w4533:waveform(dbl))
    n1629 = Multiply(x="APD Disp. Downsample", y=w4531) -> (x*y=w4529:dbl)
    n1630 = Divide(x=w4533, y=w4529) -> (x/y=w4522:waveform(dbl))
    "APD 1 Chart" <- w4522
    n1631 = Index Array(array=w4523, index=3) -> (element=w4614:waveform(dbl))
    n1632 = Index Array(array=w4523, index=6) -> (element=w4611:waveform(dbl))
    n1633 = Array Size(array=w4603) -> (size(s)=w4660:i32)
    n1634 = Add Array Elements(numeric array=w4603) -> (sum=w4671:u32)
    n1635 = call <vilib>:"Std Deviation and Variance.vi"("X"=w4603) -> ("standard deviation"=w4602:dbl)  [unwired: 1 in, 2 out]
    n1636 = Divide(x="T1 offset_x (mV)", y=1000.0) -> (x/y=w4615:dbl)
    n1637 = Multiply(x=w4597, y=w4660) -> (x*y=w4661:dbl)
    "Int. Time (s)" <- w4661
    n1638 = Divide(x=w4671, y=w4661) -> (x/y=w4600:dbl)
    "APD 1 Rate (Hz)" <- w4600
    n1639 = Divide(x=w4602, y=w4597) -> (x/y=w4601:dbl)
    "Rate sigma (Hz)" <- w4601
    n1640 = Divide(x=w4601, y=w4600) -> (x/y=→"sigma/mean":dbl)
    n1641 = Divide(x="T2 offset_x (mV)", y=1000.0) -> (x/y=w4613:dbl)
    n1642 = case shown="0, Default" "Calibration" {
      tunnel: "T1 alpha_x (nm/V)" -> [_ w5204 w5225]
      tunnel: "T1 kappa_x (pN/nm)" -> [_ _ w5215]
      tunnel: "T2 alpha_x (nm/V)" -> [_ w5203 w5223]
      tunnel: "T2 kappa_x (pN/nm)" -> [_ _ w5216]
      tunnel: w4614 -> [w5186 w5201 w5221]
      tunnel: w4611 -> [w5185 w5199 w5219]
      tunnel: [w5186 w5198 w5218] -> w4644
      tunnel: [w5185 w5197 w5217] -> w4643
      tunnel: ["T1 X (V)" ("Label.Text") "T1 X (nm)" ("Label.Text") "T1 X (pN)" ("Label.Text")] -> w4632
      tunnel: ["T2 X (V)" ("Label.Text") "T2 X (nm)" ("Label.Text") "T2 X (pN)" ("Label.Text")] -> w4631
      tunnel: ["Position (V)" ("Label.Text") "Position (nm)" ("Label.Text") "Force (pN)" ("Label.Text")] -> w4633
      tunnel: w4613 -> [_ w5189 w5208]
      tunnel: w4615 -> [_ w5192 w5210]
      tunnel: ["Mean (V)" ("Label.Text") "Mean (nm)" ("Label.Text") "Mean (pN)" ("Label.Text")] -> w4628
      tunnel: ["Difference (V)" ("Label.Text") "Difference (nm)" ("Label.Text") "Difference (pN)" ("Label.Text")] -> w4534
      frame #0 {
      }
      frame #1 {
        n1643 = Unbundle By Name(w5201) -> ("Y"=w5205:dbl[])
        n1644 = Unbundle By Name(w5199) -> ("Y"=w5190:dbl[])
        n1645 = Subtract(x=w5205, y=w5192) -> (x-y=w5193:dbl[])
        n1646 = Subtract(x=w5190, y=w5189) -> (x-y=w5191:dbl[])
        n1647 = Multiply(x=w5191, y=w5203) -> (x*y=w5200:dbl[])
        n1648 = Multiply(x=w5204, y=w5193) -> (x*y=w5202:dbl[])
        n1649 = Bundle By Name(cluster=w5199, "Y"=w5200) -> (w5197:waveform(dbl))
        n1650 = Bundle By Name(cluster=w5201, "Y"=w5202) -> (w5198:waveform(dbl))
      }
      frame #2 {
        n1651 = Unbundle By Name(w5221) -> ("Y"=w5226:dbl[])
        n1652 = Unbundle By Name(w5219) -> ("Y"=w5224:dbl[])
        n1653 = Subtract(x=w5224, y=w5208) -> (x-y=w5209:dbl[])
        n1654 = Subtract(x=w5226, y=w5210) -> (x-y=w5211:dbl[])
        n1655 = Compound Arithmetic op=MULTIPLY(w5209, w5223, w5216) -> (w5220:dbl[])
        n1656 = Compound Arithmetic op=MULTIPLY(w5215, w5225, w5211) -> (w5222:dbl[])
        n1657 = Bundle By Name(cluster=w5219, "Y"=w5220) -> (w5217:waveform(dbl))
        n1658 = Bundle By Name(cluster=w5221, "Y"=w5222) -> (w5218:waveform(dbl))
      }
    }
    n1659 = feedback #19(u16 1 ("Calibration")) -> (w4635:u16)
    n1660 = case shown="True" "Read Lateness and Rel Phase" {
      tunnel: w4575 -> [w4872 w4890]
      tunnel: w4574 -> [w4873 w4889]
      tunnel: [w4872 w4888] -> w4606
      tunnel: [w4873 w4887] -> w4605
      frame #0 {
      }
      frame #1 {
        n1661 = xnode "Read/Write Control"("FPGA VI Reference In"=w4890, "error in"=w4889) -> ("FPGA VI Reference Out"=w4888:T14, "error out"=w4887:errorcluster, "GI Relative phase"=→"GI relative phase":i16, "Relative phase"=→"Relative phase (AI1)":i16, "AI Late Counter"=→"Late Counter (AI1)":u32, "GI Late Counter"=→"GI Late Counter":u32, "MCL Late Counter"=→"MCL Late Counter":u32, "MCL Relative Phase"=→"Relative Phase (MCL)":i16, "APD Acq Relative Phase"=→"APD Acq Relative Phase":i16, "APD Gate Relative Phase"=→"APD Gate Relative Phase":i16, "APD Acq Late Counter"=→"APD Acq Late Counter":u32, "APD Gate Late Counter"=→"APD Gate Late Counter":u32, "Green FB Relative Phase"=→"Relative phase (Green FB)":i16, "GI Relative phase 2"=→"GI relative phase 2":i16, "GI Late Counter 2"=→"GI Late Counter 2":u32)
      }
    }
    n1662 = Not Equal?(x=w4635, y="Calibration") -> (x != y?=w4580:bool)
    n1663 = Unbundle By Name(w4614) -> ("Y"=w4617:dbl[])
    n1664 = Unbundle By Name(w4611) -> ("Y"=w4620:dbl[])
    n1665 = Subtract(x=w4617, y=w4615) -> (x-y=w4618:dbl[])
    n1666 = Subtract(x=w4620, y=w4613) -> (x-y=w4619:dbl[])
    n1667 = Multiply(x=w4619, y="T2 alpha_x (nm/V)") -> (x*y=w4610:dbl[])
    n1668 = Multiply(x="T1 alpha_x (nm/V)", y=w4618) -> (x*y=w4609:dbl[])
    n1669 = Multiply(x=w4643, y=-1.0) -> (x*y=w4622:waveform(dbl))
    n1670 = Subtract(x=w4610, y=w4609) -> (x-y=w4608:dbl[])
    n1671 = Unbundle By Name(w4643) -> ("Y"=w4562:dbl[])
    n1672 = Unbundle By Name(w4644) -> ("Y"=w4563:dbl[])
    n1673 = Build Array(w4644, w4622) -> (→"Force":waveform(dbl)[])
    n1674 = Subtract(x=w4608, y="Offset (nm)") -> (x-y=w4560:dbl[])
    n1675 = call <vilib>:"Mean.vi"("X"=w4562) -> ("mean"=w4538:dbl)  [unwired: 1 out]
    "T2 X" <- w4538
    n1676 = Absolute Value(x=w4563) -> (abs(x)=w4564:dbl[])
    n1677 = Absolute Value(x=w4562) -> (abs(x)=w4565:dbl[])
    n1678 = call <vilib>:"Mean.vi"("X"=w4563) -> ("mean"=w4539:dbl)  [unwired: 1 out]
    "T1 X" <- w4539
    n1679 = Add(x=w4564, y=w4565) -> (x+y=w4566:dbl[])
    n1680 = Bundle By Name(cluster=w4614, "Y"=w4560) -> (w4521:waveform(dbl))
    "Bead Separation" <- w4521
    n1681 = Divide(x=w4566, y=2.0) -> (x/y=→"Vec Mean of T1 T2":dbl[])
    n1682 = case shown="True" w4580 {
      tunnel: w4633 -> [_ w5179]
      tunnel: w4632 -> [_ w5178]
      tunnel: w4631 -> [_ w5177]
      tunnel: w4628 -> [_ w5176]
      tunnel: w4534 -> [_ w5175]
      frame #0 {
      }
      frame #1 {
        n1683 = property on="Force" class="WFChart (strict)"("YScale.NameLbl.Text"=w5179) -> ()  [unwired: 2 in, 2 out]
        n1684 = property on="T2 X" class="DigNum (strict)"("Caption.Text"=w5177) -> ()  [unwired: 2 in, 2 out]
        n1685 = property on="T1 X" class="DigNum (strict)"("Caption.Text"=w5178) -> ()  [unwired: 2 in, 2 out]
        n1686 = property on="Mean" class="DigNum (strict)"("Caption.Text"=w5176) -> ()  [unwired: 2 in, 2 out]
        n1687 = property on="Difference" class="DigNum (strict)"("Caption.Text"=w5175) -> ()  [unwired: 2 in, 2 out]
      }
    }
    n1688 = local read "Tether"() -> (w4569:bool)
    n1689 = Absolute Value(x=w4539) -> (abs(x)=w4536:dbl)
    n1690 = Absolute Value(x=w4538) -> (abs(x)=w4535:dbl)
    n1691 = local read "Display Period (s)"() -> (w4553:dbl)
    n1692 = Add(x=w4536, y=w4535) -> (x+y=w4630:dbl)
    n1693 = Subtract(x=w4536, y=w4535) -> (x-y=→"Difference":dbl)
    n1694 = feedback #20(w4560) -> (w4559:dbl[])
    n1695 = Divide(x=w4630, y=2.0) -> (x/y=w4568:dbl)
    "Mean" <- w4568
    n1696 = case shown="True" w4569 {
      tunnel: w4568 -> [_ w4823]
      frame #0 {
      }
      frame #1 {
        n1697 = Greater?(x="Lost Tether Alarm Threshold (pN)", y=w4823) -> (0:w4821:bool)
        n1698 = case shown="True" w4821 {
          frame #0 {
          }
          frame #1 {
            n1699 = flat-sequence {
              frame #0 {
                # "stop only if saving"
                n1700 = local read "Saving..."() -> (w4835:bool)
                n1701 = And(x=w4835, y="TA Cancel Save?") -> (x .and. y?=w4834:bool)
                n1702 = local write "Stop Saving"(w4834) -> ()
              }
              frame #1 {
                n1703 = case shown="True" "TA Green Off?" {
                  frame #0 {
                  }
                  frame #1 {
                    w4838 = FALSE ("Fl. Triggered...")
                    n1704 = local write "Fl. Triggered..."(w4838) -> ()
                    n1705 = property on="Green Laser ON/Interlacing" class="Bool (strict)"("Val(Sgnl)"=w4838) -> ()  [unwired: 2 in, 2 out]
                  }
                }
              }
            }
            n1706 = local read "Time tether formed"() -> (w4829:timestamp)
            n1707 = Get Date/Time In Seconds() -> (seconds since 1Jan1904=w4830:timestamp)
            n1708 = Subtract(x=w4830, y=w4829) -> (x-y=w4828:dbl)
            n1709 = Number To Decimal String(number=w4828) -> (decimal integer string=w4825:string)  [unwired: 1 out]
            n1710 = local read "Messages"() -> (w4832:string)
            n1711 = call <vilib>:"Beep.vi"() -> ()  [unwired: 3 in, 9 out]
            n1712 = Concatenate Strings("Lost tether (" ("Message to add"), w4825, " s)." ("string")) -> (w4827:string)
            n1713 = local write "Tether"(FALSE ("Tether")) -> ()
            n1714 = call "Update messages.vi"("Message to add"=w4827, "Old message string"=w4832) -> ("New message string"=w4831:string)
            n1715 = local write "Messages"(w4831) -> ()
          }
        }
      }
    }
    n1716 = Build Array (concatenate)(w4560, w4559) -> (w4558:dbl[])
    n1717 = Divide(x="Bead Sep. Int. Time (s)", y=w4553) -> (x/y=w4552:dbl)
    n1718 = Split 1D Array(array=w4558, index=w4552) -> (first subarray=w4551:dbl[])  [unwired: 1 out]
    n1719 = xnode "Read/Write Control"("FPGA VI Reference In"=w4606, "error in"=w4605) -> ("FPGA VI Reference Out"=w4734:T14, "error out"=w4728:errorcluster, "AI2 Y Sum Set 1"=w4724:i16, "AI2 Y Sum Set 2"=w4723:i16, "Scanning"=→"AOD Scanning":bool, "Scan I"=→"AOD Scan I":u64, "Scanning MCL"=w4726:bool, "Scan I (MCL)"=→"MCL Scan I":u64, "Green FB Signals"=w4653:T36)  [unwired: 1 out]
    "MCL Scanning" <- w4726
    n1720 = call <vilib>:"Mean.vi"("X"=w4551) -> ("mean"=w4550:dbl)  [unwired: 1 out]
    "Bead Mean (nm)" <- w4550
    n1721 = Subtract(x=w4551, y=w4550) -> (x-y=w4549:dbl[])
    n1722 = Square(x=w4549) -> (x^2=w4548:dbl[])
    n1723 = call <vilib>:"Mean.vi"("X"=w4548) -> ("mean"=w4547:dbl)  [unwired: 1 out]
    n1724 = Square Root(x=w4547) -> (sqrt(x)=w4546:dbl)
    n1725 = Multiply(x=10.0, y=w4546) -> (x*y=→"RMS (Ang)":dbl)
    n1726 = flat-sequence "To save data" {
      tunnel: [w7123] -> w4747
      tunnel: [w7124] -> w4746
      tunnel: w4687 -> [w7117]
      tunnel: w4556 -> [w7121]
      tunnel: ["Save Calibration"] -> w4715
      tunnel: w4710 -> [w7120]
      tunnel: [w7113] -> w4709
      tunnel: [w7110] -> w4707
      tunnel: [w7107] -> w4706
      tunnel: w4686 -> [w7109]
      tunnel: w4577 -> [w7103]
      tunnel: [w7103] -> w4576
      tunnel: ["Start Saving"] -> w4524
      tunnel: w4747 -> [w7313]
      tunnel: w4746 -> [w7312]
      tunnel: w4745 -> [w7311]
      tunnel: w4715 -> [w7310]
      tunnel: w4709 -> [w7308]
      tunnel: w4707 -> [w7307]
      tunnel: w4706 -> [w7306]
      tunnel: w4540 -> [w7305]
      tunnel: w4598 -> [w7304]
      tunnel: w4576 -> [w7303]
      tunnel: w4524 -> [w7302]
      tunnel: w4522 -> [w7301]
      tunnel: w4521 -> [w7300]
      frame #0 {
        n1727 = Or(x="Save N Sets", y="Start Saving") -> (x .or. y?=w7104:bool)
        n1728 = To Double Precision Float(number=w7120) -> (double precision float=w7114:dbl)
        n1729 = Build Array(w7104, "Save Calibration", w7117, w7109) -> (w7119:bool[])
        n1730 = Compound Arithmetic op=OR("Save Calibration", w7117, w7104, w7109) -> (w7122:bool)
        n1731 = Boolean Array To Number(Boolean array=w7119) -> (number=w7116:u32)
        n1732 = feedback #21(refnum<k0> refnum) -> (w7125:refnum<file>)
        n1733 = feedback #22(FALSE ("Save APD Data\nwith Trap Data")) -> (w7108:bool)
        n1734 = feedback #23(refnum<k0> refnum) -> (w7111:refnum<file>)
        n1735 = feedback #24(0) -> (w7127:i32)
        n1736 = feedback #25() -> (w7115:u32)  [unwired: 1 out]
        n1737 = case shown="True" w7122 {
          tunnel: [w7132 1] -> w7123
          tunnel: w7127 -> [w7134 _]
          tunnel: [w7133 w7147] -> w7124
          tunnel: w7125 -> [w7133 _]
          tunnel: w7121 -> [_ w7167]
          tunnel: w7114 -> [_ w7165]
          tunnel: w7116 -> [_ w7168]
          tunnel: [w7131 w7146] -> w7113
          tunnel: w7115 -> [w7131 _]
          tunnel: [w7130 w7143] -> w7110
          tunnel: w7111 -> [w7130 _]
          tunnel: [w7129 w7142] -> w7107
          tunnel: w7108 -> [w7129 _]
          tunnel: "Start Saving" -> [_ w7140]
          tunnel: w7103 -> [_ w7139]
          frame #0 {
            n1738 = Increment(x=w7134) -> (x+1=w7132:i32)
          }
          frame #1 {
            w7135 = FALSE ("Start Saving")
            w7141 = 9.0  # File Version
            w7150 = FALSE ("prepend array or string size? (T)")
            w7148 = T20."big-endian, network order" ("byte order (0:big-endian, network order)")
            n1739 = Array Size(array=w7139) -> (size(s)=w7138:i32)
            n1740 = local read "BD 1 Frequency 1 (MHz)"() -> (w7164:dbl)
            n1741 = local read "BD 2 Frequency 1 (MHz)"() -> (w7163:dbl)
            n1742 = local read "BD 1 Frequency 2 (MHz)"() -> (w7162:dbl)
            n1743 = local read "BD 2 Frequency 2 (MHz)"() -> (w7161:dbl)
            n1744 = local read "BD 1 Frequency 3 (MHz)"() -> (w7160:dbl)
            n1745 = local read "BD 2 Frequency 3 (MHz)"() -> (w7159:dbl)
            n1746 = To Double Precision Float(number=w7138) -> (double precision float=w7137:dbl)
            n1747 = local write "Save Calibration"(w7135) -> ()
            n1748 = local write "Start Saving"(w7135) -> ()
            n1749 = Build Array(w7164, w7163, w7162, w7161, w7160, w7159) -> (w7158:dbl[])
            n1750 = case shown="1, Default" w7168 {
              tunnel: w7167 -> [w7212 w7226 w7241 w7278]
              tunnel: w7137 -> [w7217 w7233 w7261 w7297]
              tunnel: w7165 -> [w7216 w7232 w7260 w7296]
              tunnel: [w7213 w7228 w7252 w7288] -> w7156
              tunnel: [w7202 "Cal sets to save" w7242 w7279] -> w7146
              tunnel: w7158 -> [w7214 w7229 w7254 w7290]
              tunnel: "Save APD Data\nwith Trap Data" -> [w7211 _ w7237 w7275]
              tunnel: [w7211 w7222 w7237 w7275] -> w7142
              tunnel: w7141 -> [w7205 w7220 w7235 w7273]
              tunnel: w7140 -> [w7204 _ _ _]
              frame #0 {
                w7208 = 0.0 ("f")
                # "timeseries"
                n1751 = local read "Save ave N"() -> (w7219:dbl)
                n1752 = Multiply(x=w7219, y=w7212) -> (x*y=w7218:dbl)
                n1753 = Boolean To (0,1)(Boolean=w7211) -> (0, 1=w7210:i16)
                n1754 = To Double Precision Float(number=w7210) -> (double precision float=w7209:dbl)
                n1755 = Build Array(w7205, w7212, w7218, w7217, w7216, 0.0 ("f")) -> (w7215:dbl[])
                n1756 = Build Array(w7209, w7208, w7208, w7208, w7208) -> (w7206:dbl[])
                n1757 = Select(t=u32 4000000000, s=w7204, f="N sets to save") -> (s? t:f=w7202:u32)
                n1758 = Build Array (concatenate)(w7215, w7214, w7206) -> (w7213:dbl[])
              }
              frame #1 {
                w7223 = 0.0 ("f")
                w7222 = FALSE ("Save APD Data\nwith Trap Data")
                # "calibration"
                n1759 = Boolean To (0,1)(Boolean=w7222) -> (0, 1=w7225:i16)
                n1760 = To Double Precision Float(number=w7225) -> (double precision float=w7224:dbl)
                n1761 = Build Array(w7224, w7223, w7223, w7223, w7223) -> (w7221:dbl[])
                n1762 = Build Array(w7220, w7226, w7226, w7233, w7232, 1.0 ("t")) -> (w7230:dbl[])
                n1763 = Build Array (concatenate)(w7230, w7229, w7221) -> (w7228:dbl[])
                "Calibrating Trap..." <- TRUE ("Calibrating...")
              }
              frame #2 {
                w7238 = 0.0 ("f")
                # "scan dir (x/y = 0/1)"
                # "cycles/step"
                # "n scans (f/b)"
                # "steps"
                # "freq. range"
                # "AOD raster scan"
                n1764 = local read "Number of F/B Scans (AOD)"() -> (w7246:u16)
                n1765 = local read "Cycles/step (AOD)"() -> (w7248:u64)
                n1766 = local read "Scan Range (MHz)"() -> (w7251:dbl)
                n1767 = local read "Scan steps (AOD)"() -> (w7250:u64)
                n1768 = local read "Scan BD"() -> (w7258:bool)
                n1769 = local read "Save ave N"() -> (w7263:dbl)
                n1770 = Boolean To (0,1)(Boolean=w7258) -> (0, 1=w7257:i16)
                n1771 = To Double Precision Float(number=w7246) -> (double precision float=w7245:dbl)
                n1772 = To Double Precision Float(number=w7250) -> (double precision float=w7249:dbl)
                n1773 = To Double Precision Float(number=w7248) -> (double precision float=w7247:dbl)
                n1774 = To Double Precision Float(number=w7257) -> (double precision float=w7256:dbl)
                n1775 = Boolean To (0,1)(Boolean=w7237) -> (0, 1=w7240:i16)
                n1776 = Multiply(x=w7263, y=w7241) -> (x*y=w7262:dbl)
                n1777 = To Double Precision Float(number=w7240) -> (double precision float=w7239:dbl)
                n1778 = Build Array(w7239, w7238, w7238, w7238, w7238) -> (w7236:dbl[])
                n1779 = local read "N sets should be saved"() -> (w7243:dbl)
                n1780 = Build Array(w7256, w7251, w7249, w7247, w7245) -> (w7253:dbl[])
                n1781 = Build Array(w7235, w7241, w7262, w7261, w7260, 2.0 ("t")) -> (w7255:dbl[])
                n1782 = Round Toward +Infinity(x=w7243) -> (ceil(x): smallest int >= x=w7244:dbl)
                n1783 = Build Array (concatenate)(w7255, w7254, w7236, w7253) -> (w7252:dbl[])
                n1784 = To Unsigned Long Integer(number=w7244) -> (unsigned 32bit integer=w7242:u32)
              }
              frame #3 {
                w7270 = 0.0 ("f")
                # "MCL raster scan"
                n1785 = local read "Number of scans (MCL)"() -> (w7265:u64)
                n1786 = local read "Scan lines (y)"() -> (w7264:u64)
                n1787 = local read "2D or 1D Scan"() -> (w7267:bool)
                n1788 = local read "Scan Range (V)\n(of steps)"() -> (w7287:dbl)
                n1789 = local read "Fast Scan Dir"() -> (w7294:bool)
                n1790 = local read "Cycles/step (MCL)"() -> (w7284:u64)
                n1791 = local read "Scan steps (MCL)"() -> (w7286:u64)
                n1792 = Select(t=w7264, s=w7267, f=w7265) -> (s? t:f=w7266:u64)
                n1793 = Boolean To (0,1)(Boolean=w7267) -> (0, 1=w7269:i16)
                n1794 = local read "Save ave N"() -> (w7299:dbl)
                n1795 = local read "Initial X"() -> (w7272:dbl)
                n1796 = local read "Initial Y"() -> (w7271:dbl)
                n1797 = To Double Precision Float(number=w7269) -> (double precision float=w7268:dbl)
                n1798 = Boolean To (0,1)(Boolean=w7294) -> (0, 1=w7293:i16)
                n1799 = To Double Precision Float(number=w7266) -> (double precision float=w7282:dbl)
                n1800 = To Double Precision Float(number=w7286) -> (double precision float=w7285:dbl)
                n1801 = To Double Precision Float(number=w7284) -> (double precision float=w7283:dbl)
                n1802 = To Double Precision Float(number=w7293) -> (double precision float=w7292:dbl)
                n1803 = Boolean To (0,1)(Boolean=w7275) -> (0, 1=w7277:i16)
                n1804 = Multiply(x=w7299, y=w7278) -> (x*y=w7298:dbl)
                n1805 = To Double Precision Float(number=w7277) -> (double precision float=w7276:dbl)
                n1806 = local read "N sets should be saved (MCL)"() -> (w7280:dbl)
                n1807 = Build Array(w7276, w7268, w7270, w7270, w7270) -> (w7274:dbl[])
                n1808 = Build Array(w7292, w7287, w7285, w7283, w7282, w7272, w7271) -> (w7289:dbl[])
                n1809 = Build Array(w7273, w7278, w7298, w7297, w7296, 3.0 ("t")) -> (w7291:dbl[])
                n1810 = Round Toward +Infinity(x=w7280) -> (ceil(x): smallest int >= x=w7281:dbl)
                n1811 = Build Array (concatenate)(w7291, w7290, w7274, w7289) -> (w7288:dbl[])
                n1812 = To Unsigned Long Integer(number=w7281) -> (unsigned 32bit integer=w7279:u32)
              }
            }
            n1813 = local read "Index"() -> (w7173:dbl)
            n1814 = call "Create new save file.vi"("Insert"="", "Ext"=".dat", "Index In"=w7173) -> ("Path Out"=w7144:path, "Index Out"=w7145:dbl)
            n1815 = local write "Save file name"(w7144) -> ()
            n1816 = local write "Index"(w7145) -> ()
            n1817 = local write "Save index"(w7145) -> ()
            n1818 = Array Size(array=w7156) -> (size(s)=w7157:i32)
            n1819 = Open/Create/Replace File(file path (use dialog)=w7144, operation (0:open)=T21."create", access (0:read/write)=enum16{"read/write", "read-only", "write-only"}."write-only") -> (refnum out=w7170:refnum<file>)  [unwired: 1 in, 4 out]
            n1820 = local write "Saving..."(TRUE ("Saving...")) -> ()
            n1821 = To Double Precision Float(number=w7157) -> (double precision float=w7155:dbl)
            n1822 = String Length(string="Comment (data description)") -> (length=w7153:i32)
            n1823 = To Double Precision Float(number=w7153) -> (double precision float=w7152:dbl)
            n1824 = Deny Access(7:w7170) -> (3:w7169:refnum<file>)  [unwired: 1 in, 2 out]
            n1825 = Build Array (concatenate)(w7155, w7156, w7152) -> (w7154:dbl[])
            n1826 = case "If fluorescence data to be saved" shown="True" w7142 {
              tunnel: w7144 -> [_ w7200]
              tunnel: [refnum<k0> refnum w7180] -> w7143
              frame #0 {
              }
              frame #1 {
                w7179 = 0.0
                n1827 = local read "APD Integration Time (s)"() -> (w7185:dbl)
                n1828 = local read "N APD Samp/step"() -> (w7178:dbl)
                n1829 = Path To String(path=w7200) -> (string=w7199:string)
                n1830 = String Length(string=w7199) -> (length=w7198:i32)
                n1831 = Subtract(x=w7198, y=4) -> (x-y=w7196:i32)
                n1832 = String Subset(string=w7199, length (rest)=w7196) -> (substring=w7195:string)  [unwired: 1 out]
                n1833 = Build Array(w7185, w7178, w7179, w7179, w7179, w7179, w7179, w7179) -> (w7182:dbl[])
                n1834 = Concatenate Strings(w7195, "_fl.dat" ("string")) -> (w7193:string)
                n1835 = Array Size(array=w7182) -> (size(s)=w7184:i32)
                n1836 = String To Path(string=w7193) -> (path=w7189:path)
                n1837 = Open/Create/Replace File(file path (use dialog)=w7189, operation (0:open)=T21."create", access (0:read/write)=enum16{"read/write", "read-only", "write-only"}."write-only") -> (refnum out=w7190:refnum<file>)  [unwired: 1 in, 4 out]
                n1838 = Deny Access(7:w7190) -> (3:w7186:refnum<file>)  [unwired: 1 in, 2 out]
                n1839 = To Double Precision Float(number=w7184) -> (double precision float=w7183:dbl)
                n1840 = Build Array (concatenate)(w7183, w7182) -> (w7181:dbl[])
                n1841 = Write to Binary File(file (use dialog)=w7186, data=w7181, 5:FALSE ("prepend array or string size? (T)"), 9:T20."big-endian, network order" ("byte order (0:big-endian, network order)")) -> (refnum out=w7180:refnum<file>)  [unwired: 1 in, 3 out]
              }
            }
            n1842 = Write to Binary File(file (use dialog)=w7169, data=w7154, 5:w7150, 9:w7148) -> (refnum out=w7151:refnum<file>)  [unwired: 1 in, 3 out]
            n1843 = Write to Binary File(file (use dialog)=w7151, data="Comment (data description)", 5:w7150, 9:w7148) -> (refnum out=w7147:refnum<file>)  [unwired: 1 in, 3 out]
          }
        }
      }
      frame #1 {
        n1844 = local read "Saving..."() -> (w7309:bool)
        n1845 = case shown="True" w7309 {
          tunnel: w7313 -> [_ w7320]
          tunnel: w7312 -> [_ w7334]
          tunnel: w7311 -> [_ w7330]
          tunnel: w7310 -> [_ w7329]
          tunnel: w7308 -> [_ w7328]
          tunnel: w7307 -> [_ w7323]
          tunnel: w7306 -> [_ w7322]
          tunnel: w7305 -> [_ w7321]
          tunnel: w7304 -> [_ w7319]
          tunnel: w7303 -> [_ w7317]
          tunnel: w7302 -> [_ w7316]
          tunnel: w7301 -> [_ w7315]
          tunnel: w7300 -> [_ w7314]
          frame #0 {
          }
          frame #1 {
            n1846 = Multiply(x=w7320, y=w7319) -> (x*y=→"Time (s)":dbl)
            n1847 = Less Or Equal?(x=w7320, y=w7328) -> (x <= y?=w7332:bool)
            n1848 = Or(x="Stop Saving", y="Abort save 2") -> (x .or. y?=w7324:bool)
            n1849 = Not(x=w7324) -> (.not. x?=w7333:bool)
            n1850 = And(x=w7332, y=w7333) -> (x .and. y?=w7331:bool)
            n1851 = case shown="True" w7331 {
              tunnel: w7334 -> [w7339 w7383]
              tunnel: [0.0 w7386] -> w7327
              tunnel: w7320 -> [_ w7384]
              tunnel: w7328 -> [_ w7385]
              tunnel: w7330 -> [_ w7380]
              tunnel: w7329 -> [_ _]
              tunnel: w7323 -> [w7337 w7371]
              tunnel: w7322 -> [w7336 w7372]
              tunnel: w7321 -> [_ w7370]
              tunnel: w7317 -> [_ w7369]
              tunnel: w7316 -> [_ w7342]
              tunnel: w7315 -> [_ w7362]
              tunnel: w7314 -> [_ w7361]
              frame #0 {
                w7335 = FALSE
                n1852 = Close File(refnum=w7339) -> ()  [unwired: 1 in, 2 out]
                n1853 = case shown="True" w7336 {
                  tunnel: w7337 -> [_ w7340]
                  frame #0 {
                  }
                  frame #1 {
                    n1854 = Close File(refnum=w7340) -> ()  [unwired: 1 in, 2 out]
                  }
                }
                n1855 = local write "Raster Scanning..."(w7335) -> ()
                n1856 = local write "Calibrating Trap..."(w7335) -> ()
                n1857 = call <vilib>:"Beep.vi"() -> ()  [unwired: 3 in, 9 out]
                n1858 = local write "Stop Saving"(w7335) -> ()
                "Saving..." <- w7335
              }
              frame #1 {
                n1859 = local read "Calibrating Trap..."() -> (w7373:bool)
                n1860 = case shown="True" w7372 {
                  tunnel: w7371 -> [_ w7390]
                  tunnel: w7370 -> [_ w7389]
                  frame #0 {
                  }
                  frame #1 {
                    n1861 = Write to Binary File(file (use dialog)=w7390, data=w7389, 5:FALSE ("prepend array or string size? (T)"), 9:T20."big-endian, network order" ("byte order (0:big-endian, network order)")) -> ()  [unwired: 1 in, 4 out]
                  }
                }
                n1862 = Greater?(x="Save ave N", y=1.0) -> (0:w7376:bool)
                n1863 = Not(x=w7373) -> (.not. x?=w7375:bool)
                n1864 = And(x=w7375, y=w7376) -> (x .and. y?=w7377:bool)
                n1865 = case shown="True" w7377 {
                  tunnel: w7380 -> [w7393 w7405]
                  tunnel: [w7393 w7397] -> w7374
                  tunnel: "Save ave N" -> [_ w7398]
                  tunnel: w7369 -> [_ w7396]
                  frame #0 {
                  }
                  frame #1 {
                    n1866 = Array Size(array=w7405) -> (size(s)=w7399:i32)
                    n1867 = Array Size(array=w7396) -> (size(s)=w7395:i32)
                    n1868 = Divide(x=w7399, y=w7395) -> (x/y=w7403:dbl)
                    n1869 = Reshape Array(w7405, w7403, w7395) -> (w7404:i16[][])
                    n1870 = Transpose 2D Array(2D array=w7404) -> (transposed array=w7402:i16[][])
                    n1871 = for {
                      tunnel: w7402 -> [w7408] mode=indexing
                      tunnel: [w7407] -> w7394 mode=indexing
                      tunnel: w7398 -> [w7406]
                      workers-P: _ -> [_]
                      n1872 = call "downsample 1D array - I16.vi"("Ave N"=w7406, "Array In"=w7408) -> ("Array Out"=w7407:i16[])  [unwired: 1 out]
                    }
                    n1873 = Transpose 2D Array(2D array=w7394) -> (transposed array=w7401:i16[][])
                    n1874 = Divide(x=w7399, y=w7398) -> (x/y=w7400:dbl)
                    n1875 = Reshape Array(w7401, w7400) -> (w7397:i16[])
                  }
                }
                n1876 = Unbundle By Name(w7361) -> ("Y"=w7366:dbl[])
                n1877 = Unbundle By Name(w7362) -> ("Y"=w7349:dbl[])
                n1878 = Array Size(array=w7349) -> (size(s)=→"size(s) of 1 acq array":i32)
                n1879 = Write to Binary File(file (use dialog)=w7383, data=w7374, 5:FALSE ("prepend array or string size? (T)"), 9:T20."big-endian, network order" ("byte order (0:big-endian, network order)")) -> ()  [unwired: 1 in, 4 out]
                n1880 = feedback #26(w7366) -> (w7365:dbl[])
                n1881 = Build Array (concatenate)(w7365, w7366) -> (w7364:dbl[])
                n1882 = Select(t=w7366, s=w7342, f=w7364) -> (s? t:f=w7363:dbl[])
                "Trap Delta Graph" <- w7363
                n1883 = feedback #27(w7349) -> (w7368:dbl[])
                n1884 = Build Array (concatenate)(w7368, w7349) -> (w7367:dbl[])
                n1885 = Select(t=w7349, s=w7342, f=w7367) -> (s? t:f=w7357:dbl[])
                "APD 1 Graph" <- w7357
                n1886 = Divide(x=w7384, y=w7385) -> (x/y=w7387:dbl)
                n1887 = Array Size(array=w7357) -> (size(s)=w7359:i32)
                "size(s) APD array" <- w7359
                n1888 = Multiply(x=w7387, y=100.0) -> (x*y=w7386:dbl)
                n1889 = Subtract(x=w7359, y="N pts to average") -> (x-y=w7356:i32)
                n1890 = Multiply(x="N pts to average", y=u16 2) -> (x*y=w7358:u16)
                n1891 = Subtract(x=w7359, y=w7358) -> (x-y=w7355:i32)
                n1892 = Array Subset(array=w7357, index=w7356, length="N pts to average") -> (w7353:dbl[])
                n1893 = Array Subset(array=w7357, index=w7355, length="N pts to average") -> (w7352:dbl[])
                n1894 = call <vilib>:"Mean.vi"("X"=w7353) -> ("mean"=w7351:dbl)  [unwired: 1 out]
                n1895 = call <vilib>:"Mean.vi"("X"=w7352) -> ("mean"=w7350:dbl)  [unwired: 1 out]
                n1896 = Subtract(x=w7351, y=w7350) -> (x-y=w7347:dbl)
                "Delta Fl. (Hz)" <- w7347
                n1897 = Initialize Array(w7347, 1 ("dimension size")) -> (w7344:dbl[])
                n1898 = feedback #28(w7344) -> (w7345:dbl[])
                n1899 = Build Array (concatenate)(w7345, w7344) -> (w7343:dbl[])
                n1900 = Select(t=w7344, s=w7342, f=w7343) -> (s? t:f=w7341:dbl[])
                "APD 1 Graph 2" <- w7341
              }
            }
            "Progress" <- w7327
            "Progress 2" <- w7327
          }
        }
      }
    }
    n1901 = local read "AI2 (V)"() -> (w4725:cluster{"Set 1":dbl, "Set 2":dbl})
    n1902 = Bundle By Name(cluster=w4725, "Set 1"=w4724, "Set 2"=w4723) -> (w4721:cluster{"Set 1":dbl, "Set 2":dbl})
    n1903 = Divide(x=w4721, y=3276.7) -> (x/y=w4720:cluster{"Set 1":dbl, "Set 2":dbl})
    n1904 = local write "AI2 (V)"(w4720) -> ()
    n1905 = Divide(x=w4653, y=3276.7) -> (x/y=w4649:T42)
    n1906 = Unbundle By Name(w4649) -> ("Green FB Ch 0"=w4652:dbl, "Green FB Ch 1"=w4651:dbl, "Green FB Ch 2"=w4650:dbl)
    n1907 = Divide(x=w4652, y=w4650) -> (x/y=w4648:dbl)
    n1908 = Divide(x=w4651, y=w4650) -> (x/y=w4647:dbl)
    n1909 = Bundle By Name(cluster=w4649, "Green FB Ch 0"=w4648, "Green FB Ch 1"=w4647) -> (w4627:T42)
    "Green FB Signals (V)" <- w4627
    n1910 = Unbundle By Name(w4627) -> ("Green FB Ch 2"=→"Green FB Plot":dbl)
    n1911 = local read "wait to reset values"() -> (w4729:bool)
    n1912 = Not(x=w4726) -> (.not. x?=w4730:bool)
    n1913 = And(x=w4730, y=w4729) -> (x .and. y?=w4731:bool)
    n1914 = case "Part of MCL raster scanning: returns to initial positions after scan done" shown="True" w4731 {
      tunnel: w4734 -> [w6068 w6075]
      tunnel: [w6068 w6074] -> w4733
      tunnel: w4728 -> [w6067 w6073]
      tunnel: [w6067 w6072] -> w4727
      frame #0 {
      }
      frame #1 {
        w6083 = 10.0 ("y")
        w6082 = 32767.0 ("y")
        # "to return scan values\nafter a synchronous \nAOM scan"
        n1915 = local read "AO2"() -> (w6076:dbl)
        n1916 = local read "AO1"() -> (w6077:dbl)
        n1917 = Multiply(x=w6077, y=w6082) -> (x*y=w6079:dbl)
        n1918 = local write "wait to reset values"(FALSE ("wait to reset values")) -> ()
        n1919 = Multiply(x=w6076, y=w6082) -> (x*y=w6081:dbl)
        n1920 = Divide(x=w6079, y=w6083) -> (x/y=w6078:dbl)
        n1921 = Divide(x=w6081, y=w6083) -> (x/y=w6080:dbl)
        n1922 = To Word Integer(number=w6078) -> (16bit integer=w6084:i16)
        n1923 = To Word Integer(number=w6080) -> (16bit integer=w6085:i16)
        n1924 = local read "Total Counts (ticks)"() -> (w6069:u32)
        n1925 = xnode "Read/Write Control"("FPGA VI Reference In"=w6075, "error in"=w6073, "AO1"=w6084, "AO2"=w6085, "MCL count"=w6069) -> ("FPGA VI Reference Out"=w6074:T14, "error out"=w6072:errorcluster)
        n1926 = local read "Scan Range (V)\n(of steps)"() -> (w6070:dbl)
        n1927 = property on="Scan Range (V)\n(of steps)" class="DigNum (strict)"("Val(Sgnl)"=w6070) -> ()  [unwired: 2 in, 2 out]
      }
    }
    n1928 = node-c288() -> ()  [unwired: 2 out]
  }
  n1929 = node-c288(w18) -> ()  [unwired: 1 out]
  n1930 = node-c288(w20) -> ()  [unwired: 1 out]
  n1931 = node-c288(w1) -> ()  [unwired: 1 out]
  n1932 = VISA Close(VISA resource name=w5, error in (no error)=w4) -> (error out=w62:errorcluster)
  n1933 = call <vilib>:"Simple Error Handler.vi"("error in (no error)"=w62) -> ()  [unwired: 1 in, 8 out]
  n1934 = node-c288(w16) -> ()  [unwired: 1 out]
  n1935 = node-c288(w126) -> ()  [unwired: 1 out]
  n1936 = flat-sequence {
    tunnel: w225 -> [w7484]
    tunnel: w227 -> [w7485]
    tunnel: [w7483] -> w205
    tunnel: [w7482] -> w204
    tunnel: w183 -> [_]
    tunnel: w181 -> [_]
    tunnel: w134 -> [_]
    tunnel: w22 -> [_]
    tunnel: w205 -> [w7543]
    tunnel: w204 -> [w7544]
    frame #0 {
      w7481 = FALSE ("AI to FIFO")
      n1937 = xnode "Read/Write Control"("FPGA VI Reference In"=w7485, "error in"=w7484, "AI to FIFO"=w7481, "APD to FIFO"=w7481) -> ("FPGA VI Reference Out"=w7483:T14, "error out"=w7482:errorcluster)
    }
    frame #1 {
      n1938 = xnode "Close FPGA VI Reference"("FPGA VI Reference In"=w7543, "error in"=w7544) -> ("error out"=→"error out":errorcluster)
    }
  }
